vi "Register gRPC Messages.vi"(8 "error in (no error)":errorcluster, 11 "gRPC ID":T1) -> (0 "error out":errorcluster, 3 "gRPC ID Out":T1)   [LabVIEW 2025, in "xnet-grpc_client.lvlib"]
uses:
  xnet-grpc_client.lvlib
  <vilib>/gRPC/LabVIEW gRPC Library/Shared/grpcId.ctl
  <vilib>/gRPC/LabVIEW gRPC Library/Server API/typeDefs/Message Metadata.ctl
  <vilib>/gRPC/LabVIEW gRPC Library/Server API/typeDefs/Message Element Metadata.ctl
  <vilib>/gRPC/LabVIEW gRPC Library/Server API/typeDefs/Message Element Type.ctl
  <vilib>/gRPC/LabVIEW gRPC Library/Server API/typeDefs/Enum Metadata.ctl
  <vilib>/gRPC/LabVIEW gRPC Library/grpc-lvsupport-release.lvlib
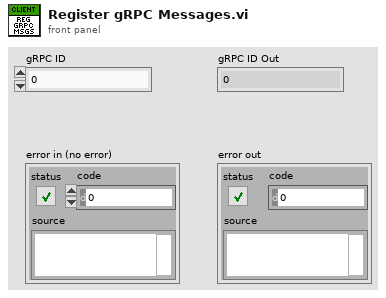
[diagram p1: front panel]
types:
  T1 = typedef "grpc-lvsupport-release.lvlib/grpcId.ctl" = u64
  T2 = typedef "grpc-lvsupport-release.lvlib/Enum Metadata.ctl" = cluster{"Version":i32, "Name":string, "Type Url":string, "Enum Values":string, "Allow Alias":bool}
  T3 = typedef "grpc-lvsupport-release.lvlib/Message Metadata.ctl" = cluster{"Version":i32, "Name":string, "Type Url":string, "Elements":T4[], "Has Oneof":bool}
  T4 = typedef "grpc-lvsupport-release.lvlib/Message Element Metadata.ctl" = cluster{"Field Name":string, "Embedded Message Name":string, "Protobuf Index":i32, "MessageElementType":T5, "Repeated":bool, "Is in Oneof":bool, "Oneof Container Name":string}
  T5 = typedef "grpc-lvsupport-release.lvlib/Message Element Type.ctl" = enum32{"Int32Value", "FloatValue", "DoubleValue", "BoolValue", "StringValue", "MessageValue", "Int64Value", "UInt32Value", "UInt64Value", "EnumValue", "Bytes", "Fixed64", "Fixed32", "SFixed64", "SFixed32", "SInt64", "SInt32"}
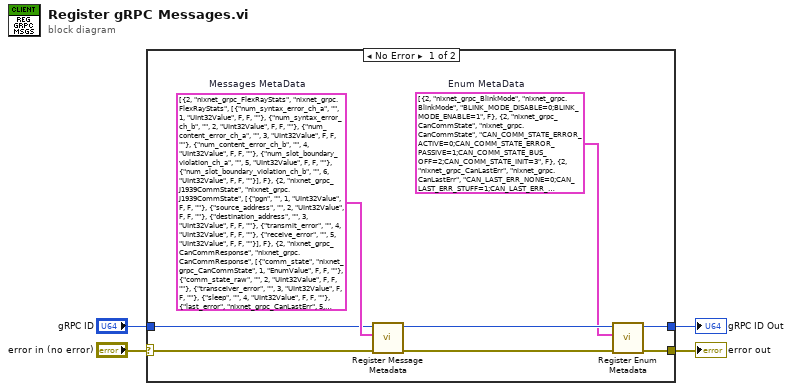
[diagram p0: block diagram]
diagram:
  n1 = case shown="No Error" "error in (no error)" {
    selector: "error in (no error)" -> [w10 w13]
    tunnel: [w9 w12] -> w1
    tunnel: [w6 w13] -> w4
    tunnel: "gRPC ID" -> [w9 w12]
    frame No Error {
      w5 = T2[] [{"Version"=2, "Name"="nixnet_grpc_BlinkMode", "Type Url"="nixnet_grpc.BlinkMode", "Enum Values"="BLINK_MODE_DISABLE=0;BLINK_MODE_ENABLE=1", "Allow Alias"=FALSE}, {"Version"=2, "Name"="nixnet_grpc_CanCommState", "Type Url"="nixnet_grpc.CanCommState", "Enum Values"="CAN_COMM_STATE_ERROR_ACTIVE=0;CAN_COMM_STATE_ERROR_PASSIVE=1;CAN_COMM_STATE_BUS_OFF=2;CAN_COMM_STATE_INIT=3", "Allow Alias"=FALSE}, {"Version"=2, "Name"="nixnet_grpc_CanLastErr", "Type Url"="nixnet_grpc.CanLastErr", "Enum Values"="CAN_LAST_ERR_NONE=0;CAN_LAST_ERR_STUFF=1;CAN_LAST_ERR_FORM=2;CAN_LAST_ERR_ACK=3;CAN_LAST_ERR_BIT_1=4;CAN_LAST_ERR_BIT_0=5;CAN_LAST_ERR_CRC=6", "Allow Alias"=FALSE}, {"Version"=2, "Name"="nixnet_grpc_CopyMode", "Type Url"="nixnet_grpc.CopyMode", "Enum Values"="COPY_MODE_DB_MERGE_COPY_USE_SOURCE=0;COPY_MODE_DB_MERGE_COPY_USE_TARGET=1;COPY_MODE_DB_MERGE_MERGE_USE_SOURCE=2;COPY_MODE_DB_MERGE_MERGE_USE_TARGET=3", "Allow Alias"=FALSE}, {"Version"=2, "Name"="nixnet_grpc_CreateSessionMode", "Type Url"="nixnet_grpc.CreateSessionMode", "Enum Values"="CREATE_SESSION_MODE_SIGNAL_IN_SINGLE_POINT=0;CREATE_SESSION_MODE_SIGNAL_IN_WAVEFORM=1;CREATE_SESSION_MODE_SIGNAL_IN_XY=2;CREATE_SESSION_MODE_SIGNAL_OUT_SINGLE_POINT=3;CREATE_SESSION_MODE_SIGNAL_OUT_WAVEFORM=4;CREATE_SESSION_MODE_SIGNAL_OUT_XY=5;CREATE_SESSION_MODE_FRAME_IN_STREAM=6;CREATE_SESSION_MODE_FRAME_IN_QUEUED=7;CREATE_SESSION_MODE_FRAME_IN_SINGLE_POINT=8;CREATE_SESSION_MODE_FRAME_OUT_STREAM=9;CREATE_SESSION_MODE_FRAME_OUT_QUEUED=10;CREATE_SESSION_MODE_FRAME_OUT_SINGLE_POINT=11;CREATE_SESSION_MODE_SIGNAL_CONVERSION_SINGLE_POINT=12", "Allow Alias"=FALSE}, {"Version"=2, "Name"="nixnet_grpc_DBProperty", "Type Url"="nixnet_grpc.DBProperty", "Enum Values"="DB_PROPERTY_UNSPECIFIED=0;DB_PROPERTY_DATABASE_CLST_REFS=100663298;DB_PROPERTY_DATABASE_NAME=50331649;DB_PROPERTY_DATABASE_SHOW_INVALID_FROM_OPEN=33554435;DB_PROPERTY_CLST_BAUD_RATE_64=151060481;DB_PROPERTY_CLST_APPLICATION_PROTOCOL=65651;DB_PROPERTY_CLST_BAUD_RATE=65537;DB_PROPERTY_CLST_CAN_FD_BAUD_RATE_64=151060497;DB_PROPERTY_CLST_CAN_FD_BAUD_RATE=65553;DB_PROPERTY_CLST_CAN_FD_ISO_MODE=65652;DB_PROPERTY_CLST_CAN_IO_MODE=65552;DB_PROPERTY_CLST_COMMENT=50397192;DB_PROPERTY_CLST_CONFIG_STATUS=65545;DB_PROPERTY_CLST_DATABASE_REF=83951618;DB_PROPERTY_CLST_ECU_REFS=100728835;DB_PROPERTY_CLST_FLEX_RAY_ACT_PT_OFF=65568;DB_PROPERTY_CLST_FLEX_RAY_ALW_PASS_ACT=65650;DB_PROPERTY_CLST_FLEX_RAY_CAS_RX_L_MAX=65569;DB_PROPERTY_CLST_FLEX_RAY_CHANNELS=65570;DB_PROPERTY_CLST_FLEX_RAY_CLST_DRIFT_DMP=65571;DB_PROPERTY_CLST_FLEX_RAY_COLD_ST_ATS=65572;DB_PROPERTY_CLST_FLEX_RAY_CYCLE=65573;DB_PROPERTY_CLST_FLEX_RAY_DYN_SEG_START=65574;DB_PROPERTY_CLST_FLEX_RAY_DYN_SLOT_IDL_PH=65575;DB_PROPERTY_CLST_FLEX_RAY_LATEST_GUAR_DYN=65579;DB_PROPERTY_CLST_FLEX_RAY_LATEST_USABLE_DYN=65578;DB_PROPERTY_CLST_FLEX_RAY_LIS_NOISE=65576;DB_PROPERTY_CLST_FLEX_RAY_MACRO_PER_CYCLE=65577;DB_PROPERTY_CLST_FLEX_RAY_MACROTICK=16842800;DB_PROPERTY_CLST_FLEX_RAY_MAX_WO_CLK_COR_FAT=65585;DB_PROPERTY_CLST_FLEX_RAY_MAX_WO_CLK_COR_PAS=65586;DB_PROPERTY_CLST_FLEX_RAY_MINISLOT=65588;DB_PROPERTY_CLST_FLEX_RAY_MINISLOT_ACT_PT=65587;DB_PROPERTY_CLST_FLEX_RAY_NIT=65590;DB_PROPERTY_CLST_FLEX_RAY_NIT_START=65591;DB_PROPERTY_CLST_FLEX_RAY_NM_VEC_LEN=65589;DB_PROPERTY_CLST_FLEX_RAY_NUM_MINISLT=65592;DB_PROPERTY_CLST_FLEX_RAY_NUM_STAT_SLT=65593;DB_PROPERTY_CLST_FLEX_RAY_OFF_COR_ST=65600;DB_PROPERTY_CLST_FLEX_RAY_PAYLD_LEN_DYN_MAX=65601;DB_PROPERTY_CLST_FLEX_RAY_PAYLD_LEN_MAX=65602;DB_PROPERTY_CLST_FLEX_RAY_PAYLD_LEN_ST=65603;DB_PROPERTY_CLST_FLEX_RAY_STAT_SLOT=65605;DB_PROPERTY_CLST_FLEX_RAY_SYM_WIN=65606;DB_PROPERTY_CLST_FLEX_RAY_SYM_WIN_START=65607;DB_PROPERTY_CLST_FLEX_RAY_SYNC_NODE_MAX=65608;DB_PROPERTY_CLST_FLEX_RAY_TSS_TX=65609;DB_PROPERTY_CLST_FLEX_RAY_USE_WAKEUP=33620053;DB_PROPERTY_CLST_FLEX_RAY_WAKE_SYM_RX_IDL=65616;DB_PROPERTY_CLST_FLEX_RAY_WAKE_SYM_RX_LOW=65617;DB_PROPERTY_CLST_FLEX_RAY_WAKE_SYM_RX_WIN=65618;DB_PROPERTY_CLST_FLEX_RAY_WAKE_SYM_TX_IDL=65619;DB_PROPERTY_CLST_FLEX_RAY_WAKE_SYM_TX_LOW=65620;DB_PROPERTY_CLST_FRM_REFS=100728836;DB_PROPERTY_CLST_LIN_SCHEDULES=100728944;DB_PROPERTY_CLST_LIN_TICK=16842865;DB_PROPERTY_CLST_NAME=50397189;DB_PROPERTY_CLST_PDU_REFS=100728840;DB_PROPERTY_CLST_PD_US_REQD=33619978;DB_PROPERTY_CLST_PROTOCOL=65542;DB_PROPERTY_CLST_SIG_REFS=100728839;DB_PROPERTY_FRM_APPLICATION_PROTOCOL=131172;DB_PROPERTY_FRM_CAN_EXT_ID=33685520;DB_PROPERTY_FRM_CAN_IO_MODE=131174;DB_PROPERTY_FRM_CAN_TIMING_TYPE=131089;DB_PROPERTY_FRM_CAN_TX_TIME=16908306;DB_PROPERTY_FRM_CLUSTER_REF=84017153;DB_PROPERTY_FRM_COMMENT=50462722;DB_PROPERTY_FRM_CONFIG_STATUS=131081;DB_PROPERTY_FRM_DEFAULT_PAYLOAD=167903237;DB_PROPERTY_FRM_FLEX_RAY_BASE_CYCLE=131104;DB_PROPERTY_FRM_FLEX_RAY_CH_ASSIGN=131105;DB_PROPERTY_FRM_FLEX_RAY_CYCLE_REP=131106;DB_PROPERTY_FRM_FLEX_RAY_IN_CYC_REP_CH_ASSIGNS=134348850;DB_PROPERTY_FRM_FLEX_RAY_IN_CYC_REP_ENABLED=33685552;DB_PROPERTY_FRM_FLEX_RAY_IN_CYC_REP_IDS=134348849;DB_PROPERTY_FRM_FLEX_RAY_PREAMBLE=33685539;DB_PROPERTY_FRM_FLEX_RAY_STARTUP=33685540;DB_PROPERTY_FRM_FLEX_RAY_SYNC=33685541;DB_PROPERTY_FRM_FLEX_RAY_TIMING_TYPE=131110;DB_PROPERTY_FRM_ID=131075;DB_PROPERTY_FRM_LIN_CHECKSUM=131152;DB_PROPERTY_FRM_MUX_DATA_MUX_SIG_REF=84017217;DB_PROPERTY_FRM_MUX_IS_MUXED=33685568;DB_PROPERTY_FRM_MUX_STATIC_SIG_REFS=100794434;DB_PROPERTY_FRM_MUX_SUBFRAME_REFS=100794435;DB_PROPERTY_FRM_NAME=50462724;DB_PROPERTY_FRM_PDU_START_BITS=134348897;DB_PROPERTY_FRM_PDU_UPDATE_BITS=134348899;DB_PROPERTY_FRM_PDU_REFS=100794464;DB_PROPERTY_FRM_PAYLOAD_LEN=131079;DB_PROPERTY_FRM_SIG_REFS=100794376;DB_PROPERTY_FRM_VARIABLE_PAYLOAD=33685605;DB_PROPERTY_SIG_BYTE_ORDR=196609;DB_PROPERTY_SIG_COMMENT=50528258;DB_PROPERTY_SIG_CONFIG_STATUS=196617;DB_PROPERTY_SIG_DATA_TYPE=196611;DB_PROPERTY_SIG_DEFAULT=16973828;DB_PROPERTY_SIG_FRAME_REF=84082693;DB_PROPERTY_SIG_MAX=16973830;DB_PROPERTY_SIG_MIN=16973831;DB_PROPERTY_SIG_MUX_IS_DATA_MUX=33751088;DB_PROPERTY_SIG_MUX_IS_DYNAMIC=33751089;DB_PROPERTY_SIG_MUX_VALUE=196658;DB_PROPERTY_SIG_MUX_SUBFRM_REF=84082739;DB_PROPERTY_SIG_NAME=50528264;DB_PROPERTY_SIG_NAME_UNIQUE_TO_CLUSTER=50528272;DB_PROPERTY_SIG_NUM_BITS=196626;DB_PROPERTY_SIG_PDU_REF=84082705;DB_PROPERTY_SIG_SCALE_FAC=16973843;DB_PROPERTY_SIG_SCALE_OFF=16973844;DB_PROPERTY_SIG_START_BIT=196629;DB_PROPERTY_SIG_UNIT=50528278;DB_PROPERTY_SUBFRM_CONFIG_STATUS=262153;DB_PROPERTY_SUBFRM_DYN_SIG_REFS=100925441;DB_PROPERTY_SUBFRM_FRM_REF=84148226;DB_PROPERTY_SUBFRM_MUX_VALUE=262147;DB_PROPERTY_SUBFRM_NAME=50593796;DB_PROPERTY_SUBFRM_NAME_UNIQUE_TO_CLUSTER=50593799;DB_PROPERTY_SUBFRM_PDU_REF=84148229;DB_PROPERTY_ECU_CLST_REF=84213761;DB_PROPERTY_ECU_COMMENT=50659333;DB_PROPERTY_ECU_CONFIG_STATUS=327689;DB_PROPERTY_ECU_FLEX_RAY_IS_COLDSTART=33882128;DB_PROPERTY_ECU_FLEX_RAY_CONNECTED_CHS=327700;DB_PROPERTY_ECU_FLEX_RAY_STARTUP_FRAME_REF=84213777;DB_PROPERTY_ECU_FLEX_RAY_WAKEUP_CHS=327699;DB_PROPERTY_ECU_FLEX_RAY_WAKEUP_PTRN=327698;DB_PROPERTY_ECU_RX_FRM_REFS=100990979;DB_PROPERTY_ECU_TX_FRM_REFS=100990980;DB_PROPERTY_ECU_LIN_CONFIG_NAD=327715;DB_PROPERTY_ECU_LIN_FUNCTION_ID=327717;DB_PROPERTY_ECU_LIN_INITIAL_NAD=327714;DB_PROPERTY_ECU_LIN_MASTER=33882144;DB_PROPERTY_ECU_LINP2MIN=17104934;DB_PROPERTY_ECU_LIN_PROTOCOL_VER=327713;DB_PROPERTY_ECU_LINS_TMIN=17104935;DB_PROPERTY_ECU_LIN_SUPPLIER_ID=327716;DB_PROPERTY_ECU_NAME=50659330;DB_PROPERTY_ECU_J1939_NODE_NAME=151322665;DB_PROPERTY_ECU_J1939_PREFERRED_ADDRESS=327720;DB_PROPERTY_LIN_SCHED_CLST_REF=84279301;DB_PROPERTY_LIN_SCHED_COMMENT=50724870;DB_PROPERTY_LIN_SCHED_CONFIG_STATUS=393223;DB_PROPERTY_LIN_SCHED_ENTRIES=101056513;DB_PROPERTY_LIN_SCHED_NAME=50724866;DB_PROPERTY_LIN_SCHED_PRIORITY=393219;DB_PROPERTY_LIN_SCHED_RUN_MODE=393220;DB_PROPERTY_LIN_SCHED_ENTRY_COLLISION_RES_SCHED=84344833;DB_PROPERTY_LIN_SCHED_ENTRY_DELAY=17235970;DB_PROPERTY_LIN_SCHED_ENTRY_EVENT_ID=458755;DB_PROPERTY_LIN_SCHED_ENTRY_FRAMES=101122052;DB_PROPERTY_LIN_SCHED_ENTRY_NAME=50790406;DB_PROPERTY_LIN_SCHED_ENTRY_NAME_UNIQUE_TO_CLUSTER=50790408;DB_PROPERTY_LIN_SCHED_ENTRY_NC_FF_DATA_BYTES=168230921;DB_PROPERTY_LIN_SCHED_ENTRY_SCHED=84344839;DB_PROPERTY_LIN_SCHED_ENTRY_TYPE=458757;DB_PROPERTY_PDU_CLUSTER_REF=84410372;DB_PROPERTY_PDU_COMMENT=50855938;DB_PROPERTY_PDU_CONFIG_STATUS=524295;DB_PROPERTY_PDU_DEFAULT_PAYLOAD=168296453;DB_PROPERTY_PDU_FRM_REFS=101187590;DB_PROPERTY_PDU_MUX_DATA_MUX_SIG_REF=84410377;DB_PROPERTY_PDU_MUX_IS_MUXED=34078728;DB_PROPERTY_PDU_MUX_STATIC_SIG_REFS=101187594;DB_PROPERTY_PDU_MUX_SUBFRAME_REFS=101187595;DB_PROPERTY_PDU_NAME=50855937;DB_PROPERTY_PDU_PAYLOAD_LEN=524291;DB_PROPERTY_PDU_SIG_REFS=101187589", "Allow Alias"=FALSE}, {"Version"=2, "Name"="nixnet_grpc_DBPropertyValue", "Type Url"="nixnet_grpc.DBPropertyValue", "Enum Values"="DB_PROPERTY_VALUE_UNSPECIFIED=0;DB_PROPERTY_VALUE_CAN_IO_MODE_CAN=1;DB_PROPERTY_VALUE_CAN_IO_MODE_CAN_FD=2;DB_PROPERTY_VALUE_CAN_IO_MODE_CAN_FD_BRS=3;DB_PROPERTY_VALUE_PROTOCOL_UNKNOWN=4;DB_PROPERTY_VALUE_PROTOCOL_CAN=5;DB_PROPERTY_VALUE_PROTOCOL_FLEX_RAY=6;DB_PROPERTY_VALUE_PROTOCOL_LIN=7;DB_PROPERTY_VALUE_PROTOCOL_ETHERNET=8;DB_PROPERTY_VALUE_APP_PROTOCOL_NONE=9;DB_PROPERTY_VALUE_APP_PROTOCOL_J1939=10;DB_PROPERTY_VALUE_FRM_FLEX_RAY_CH_ASSIGN_A=11;DB_PROPERTY_VALUE_FRM_FLEX_RAY_CH_ASSIGN_B=12;DB_PROPERTY_VALUE_FRM_FLEX_RAY_CH_ASSIGN_A_AND_B=13;DB_PROPERTY_VALUE_FRM_FLEX_RAY_CH_ASSIGN_NONE=14;DB_PROPERTY_VALUE_CLST_FLEX_RAY_SAMP_CLK_PER_P0125US=15;DB_PROPERTY_VALUE_CLST_FLEX_RAY_SAMP_CLK_PER_P025US=16;DB_PROPERTY_VALUE_CLST_FLEX_RAY_SAMP_CLK_PER_P05US=17;DB_PROPERTY_VALUE_SIG_BYTE_ORDR_LITTLE_ENDIAN=18;DB_PROPERTY_VALUE_SIG_BYTE_ORDR_BIG_ENDIAN=19;DB_PROPERTY_VALUE_SIG_DATA_TYPE_SIGNED=20;DB_PROPERTY_VALUE_SIG_DATA_TYPE_UNSIGNED=21;DB_PROPERTY_VALUE_SIG_DATA_TYPE_IEEE_FLOAT=22;DB_PROPERTY_VALUE_SIG_DATA_TYPE_BYTE_ARRAY=23;DB_PROPERTY_VALUE_LIN_PROTOCOL_VER_1_2=24;DB_PROPERTY_VALUE_LIN_PROTOCOL_VER_1_3=25;DB_PROPERTY_VALUE_LIN_PROTOCOL_VER_2_0=26;DB_PROPERTY_VALUE_LIN_PROTOCOL_VER_2_1=27;DB_PROPERTY_VALUE_LIN_PROTOCOL_VER_2_2=28;DB_PROPERTY_VALUE_LIN_SCHED_RUN_MODE_CONTINUOUS=29;DB_PROPERTY_VALUE_LIN_SCHED_RUN_MODE_ONCE=30;DB_PROPERTY_VALUE_LIN_SCHED_RUN_MODE_NULL=31;DB_PROPERTY_VALUE_LIN_SCHED_ENTRY_TYPE_UNCONDITIONAL=32;DB_PROPERTY_VALUE_LIN_SCHED_ENTRY_TYPE_SPORADIC=33;DB_PROPERTY_VALUE_LIN_SCHED_ENTRY_TYPE_EVENT_TRIGGERED=34;DB_PROPERTY_VALUE_LIN_SCHED_ENTRY_TYPE_NODE_CONFIG_SERVICE=35", "Allow Alias"=FALSE}, {"Version"=2, "Name"="nixnet_grpc_EnetFlags", "Type Url"="nixnet_grpc.EnetFlags", "Enum Values"="ENET_FLAGS_UNSPECIFIED=0;ENET_FLAGS_TRANSMIT=1;ENET_FLAGS_RECEIVE=2;ENET_FLAGS_NETWORK_SYNCED=3;ENET_FLAGS_ERROR=4", "Allow Alias"=FALSE}, {"Version"=2, "Name"="nixnet_grpc_EnetFrameType", "Type Url"="nixnet_grpc.EnetFrameType", "Enum Values"="ENET_FRAME_TYPE_DATA=0;ENET_FRAME_TYPE_DELAY=225;ENET_FRAME_TYPE_FUTURE_TIME_WAIT=226", "Allow Alias"=FALSE}, {"Version"=2, "Name"="nixnet_grpc_FlexRayPocState", "Type Url"="nixnet_grpc.FlexRayPocState", "Enum Values"="FLEX_RAY_POC_STATE_DEFAULT_CONFIG=0;FLEX_RAY_POC_STATE_READY=1;FLEX_RAY_POC_STATE_NORMAL_ACTIVE=2;FLEX_RAY_POC_STATE_NORMAL_PASSIVE=3;FLEX_RAY_POC_STATE_HALT=4;FLEX_RAY_POC_STATE_MONITOR=5;FLEX_RAY_POC_STATE_CONFIG=15", "Allow Alias"=FALSE}, {"Version"=2, "Name"="nixnet_grpc_FlexRaySymbol", "Type Url"="nixnet_grpc.FlexRaySymbol", "Enum Values"="FLEX_RAY_SYMBOL_MTS=0;FLEX_RAY_SYMBOL_WAKEUP=1", "Allow Alias"=FALSE}, {"Version"=2, "Name"="nixnet_grpc_FrameFlags", "Type Url"="nixnet_grpc.FrameFlags", "Enum Values"="FRAME_FLAGS_UNSPECIFIED=0;FRAME_FLAGS_FLEX_RAY_STARTUP=1;FRAME_FLAGS_FLEX_RAY_SYNC=2;FRAME_FLAGS_FLEX_RAY_PREAMBLE=4;FRAME_FLAGS_FLEX_RAY_CH_A=16;FRAME_FLAGS_FLEX_RAY_CH_B=32;FRAME_FLAGS_LIN_EVENT_SLOT=1;FRAME_FLAGS_TRANSMIT_ECHO=128", "Allow Alias"=TRUE}, {"Version"=2, "Name"="nixnet_grpc_FrameType", "Type Url"="nixnet_grpc.FrameType", "Enum Values"="FRAME_TYPE_CAN_DATA=0;FRAME_TYPE_CAN_REMOTE=1;FRAME_TYPE_CAN_BUS_ERROR=2;FRAME_TYPE_CAN20_DATA=8;FRAME_TYPE_CANFD_DATA=16;FRAME_TYPE_CANFDBRS_DATA=24;FRAME_TYPE_FLEX_RAY_DATA=32;FRAME_TYPE_FLEX_RAY_NULL=33;FRAME_TYPE_FLEX_RAY_SYMBOL=34;FRAME_TYPE_LIN_DATA=64;FRAME_TYPE_LIN_BUS_ERROR=65;FRAME_TYPE_LIN_NO_RESPONSE=66;FRAME_TYPE_J1939_DATA=192;FRAME_TYPE_SPECIAL_DELAY=224;FRAME_TYPE_SPECIAL_LOG_TRIGGER=225;FRAME_TYPE_SPECIAL_START_TRIGGER=226", "Allow Alias"=FALSE}, {"Version"=2, "Name"="nixnet_grpc_GetDBCAttributeMode", "Type Url"="nixnet_grpc.GetDBCAttributeMode", "Enum Values"="GET_DBC_ATTRIBUTE_MODE_ATTRIBUTE=0;GET_DBC_ATTRIBUTE_MODE_ENUMERATION_LIST=1;GET_DBC_ATTRIBUTE_MODE_ATTRIBUTE_LIST=2;GET_DBC_ATTRIBUTE_MODE_VALUE_TABLE_LIST=3", "Allow Alias"=FALSE}, {"Version"=2, "Name"="nixnet_grpc_LinCommState", "Type Url"="nixnet_grpc.LinCommState", "Enum Values"="LIN_COMM_STATE_IDLE=0;LIN_COMM_STATE_ACTIVE=1;LIN_COMM_STATE_INACTIVE=2", "Allow Alias"=FALSE}, {"Version"=2, "Name"="nixnet_grpc_LinDiagnosticSchedule", "Type Url"="nixnet_grpc.LinDiagnosticSchedule", "Enum Values"="LIN_DIAGNOSTIC_SCHEDULE_NULL=0;LIN_DIAGNOSTIC_SCHEDULE_MASTER_REQ=1;LIN_DIAGNOSTIC_SCHEDULE_SLAVE_RESP=2", "Allow Alias"=FALSE}, {"Version"=2, "Name"="nixnet_grpc_LinLastErrCode", "Type Url"="nixnet_grpc.LinLastErrCode", "Enum Values"="LIN_LAST_ERR_CODE_NONE=0;LIN_LAST_ERR_CODE_UNKNOWN_ID=1;LIN_LAST_ERR_CODE_FORM=2;LIN_LAST_ERR_CODE_FRAMING=3;LIN_LAST_ERR_CODE_READBACK=4;LIN_LAST_ERR_CODE_TIMEOUT=5;LIN_LAST_ERR_CODE_CRC=6", "Allow Alias"=FALSE}, {"Version"=2, "Name"="nixnet_grpc_Property", "Type Url"="nixnet_grpc.Property", "Enum Values"="PROPERTY_UNSPECIFIED=0;PROPERTY_SESSION_APPLICATION_PROTOCOL=1048721;PROPERTY_SESSION_AUTO_START=34603009;PROPERTY_SESSION_CLUSTER_NAME=51380234;PROPERTY_SESSION_DATABASE_NAME=51380226;PROPERTY_SESSION_ENET_FRAME_FILTER=51380468;PROPERTY_SESSION_ENET_LOG_ERROR=34603197;PROPERTY_SESSION_ENET_LOG_FILE=51380410;PROPERTY_SESSION_ENET_LOG_MODE=1048761;PROPERTY_SESSION_ENET_LOG_ENABLE_MULTIPLE_FILES=34603257;PROPERTY_SESSION_ENET_LOG_FILE_SIZE_THRESHOLD=152043770;PROPERTY_SESSION_ENET_LOG_OPERATION=1048763;PROPERTY_SESSION_ENET_NUM_FRAMES_RECEIVED=152043759;PROPERTY_SESSION_ENET_SOURCE_MAC_ADDRESS_AUTO=34603177;PROPERTY_SESSION_INTF_BAUD_RATE_64=152043542;PROPERTY_SESSION_INTF_ADJUST_LOCAL_TIME=152043691;PROPERTY_SESSION_INTF_BAUD_RATE=1048598;PROPERTY_SESSION_INTF_BUS_ERR_TO_IN_STRM=34603029;PROPERTY_SESSION_INTF_CAN_FD_BAUD_RATE_64=152043559;PROPERTY_SESSION_INTF_CAN_DISABLE_PROT_EXCEPTION_HANDLING=34603172;PROPERTY_SESSION_INTF_CAN_EDGE_FILTER=34603170;PROPERTY_SESSION_INTF_CAN_EXT_TCVR_CONFIG=1048611;PROPERTY_SESSION_INTF_CAN_FD_BAUD_RATE=1048615;PROPERTY_SESSION_INTF_CAN_FD_ISO_MODE=1048638;PROPERTY_SESSION_INTF_CAN_IO_MODE=1048614;PROPERTY_SESSION_INTF_CAN_LSTN_ONLY=34603042;PROPERTY_SESSION_INTF_CAN_PEND_TX_ORDER=1048608;PROPERTY_SESSION_INTF_CAN_SING_SHOT=34603044;PROPERTY_SESSION_INTF_CAN_TERM=1048613;PROPERTY_SESSION_INTF_CAN_TCVR_STATE=1048616;PROPERTY_SESSION_INTF_CAN_TCVR_TYPE=1048617;PROPERTY_SESSION_INTF_CAN_TX_IO_MODE=1048633;PROPERTY_SESSION_INTF_CAN_TRANSMIT_PAUSE=34603171;PROPERTY_SESSION_INTF_ECHO_TX=34603024;PROPERTY_SESSION_INTF_ENET_EPT_RECEIVE_FILTER=202375356;PROPERTY_SESSION_INTF_ENET_EPT_TRANSMIT_BANDWIDTH=152043711;PROPERTY_SESSION_INTF_ENET_IPV4_ADDRESS=51380459;PROPERTY_SESSION_INTF_ENET_JUMBO_FRAMES=1048819;PROPERTY_SESSION_INTF_ENET_LINK_SPEED=1048818;PROPERTY_SESSION_INTF_ENET_LINK_SPEED_CONFIGURED=1048817;PROPERTY_SESSION_INTF_ENET_MAC_ADDRESS=51380392;PROPERTY_SESSION_INTF_ENET_OS_NETWORK_ADAPTER_DESCRIPTION=51380461;PROPERTY_SESSION_INTF_ENET_OS_NETWORK_ADAPTER_NAME=51380460;PROPERTY_SESSION_INTF_ENET_OPERATIONAL_STATUS=1048746;PROPERTY_SESSION_INTF_ENET_OUT_STRM_TIMESCALE=1048823;PROPERTY_SESSION_INTF_ENET_PHY_POWER_MODE=1048825;PROPERTY_SESSION_INTF_ENET_PHY_STATE=1048743;PROPERTY_SESSION_INTF_ENET_PORT_MODE=1048742;PROPERTY_SESSION_INTF_ENET_SIGNAL_QUALITY=235929846;PROPERTY_SESSION_INTF_ENET_SLEEP_CAPABILITY=1048824;PROPERTY_SESSION_INTF_ENET_STATS_COUNTER_NAMES=68157612;PROPERTY_SESSION_INTF_ENET_STATS_COUNTER_VALUES=68157613;PROPERTY_SESSION_INTF_ENET_STATS_RX_BAD_FRAMES=152043702;PROPERTY_SESSION_INTF_ENET_STATS_RX_BYTES=152043694;PROPERTY_SESSION_INTF_ENET_STATS_RX_GOOD_FRAMES=152043695;PROPERTY_SESSION_INTF_ENET_STATS_TX_BYTES=152043703;PROPERTY_SESSION_INTF_ENET_STATS_TX_GOOD_FRAMES=152043704;PROPERTY_SESSION_INTF_ENET_STATS_PHY_COUNTER_NAMES=68157693;PROPERTY_SESSION_INTF_ENET_STATS_PHY_COUNTER_VALUES=68157694;PROPERTY_SESSION_INTF_ENET_STATS_PHY_LOW_POWER_SLEEP=152043777;PROPERTY_SESSION_INTF_ENET_STATS_PHY_SLEEP_FAILURE=152043779;PROPERTY_SESSION_INTF_ENET_STATS_PHY_WAKEUP_FAILURE=152043778;PROPERTY_SESSION_INTF_ENET_STATS_PHY_WAKEUP_PULSE=152043775;PROPERTY_SESSION_INTF_ENET_STATS_PHY_WAKEUP_REQUEST=152043776;PROPERTY_SESSION_INTF_ENET_TIME_ADJUST_NETWORK_TIME=152043729;PROPERTY_SESSION_INTF_ENET_TIME_BMCA_ENABLED=34603202;PROPERTY_SESSION_INTF_ENET_TIME_CLK_ACCURACY=1048774;PROPERTY_SESSION_INTF_ENET_TIME_CLK_CLASS=1048773;PROPERTY_SESSION_INTF_ENET_TIME_CLK_ID=51380420;PROPERTY_SESSION_INTF_ENET_TIME_CLK_OFFSET_VAR=1048775;PROPERTY_SESSION_INTF_ENET_TIME_GM_CLK_ACCURACY=1048781;PROPERTY_SESSION_INTF_ENET_TIME_GM_CLK_CLASS=1048780;PROPERTY_SESSION_INTF_ENET_TIME_GM_CLK_ID=51380427;PROPERTY_SESSION_INTF_ENET_TIME_GM_CLK_OFFSET_VAR=1048782;PROPERTY_SESSION_INTF_ENET_TIME_GM_PRIORITY_1=1048783;PROPERTY_SESSION_INTF_ENET_TIME_GM_PRIORITY_2=1048784;PROPERTY_SESSION_INTF_ENET_TIME_OFFSET_FROM_MASTER=152043715;PROPERTY_SESSION_INTF_ENET_TIME_PORT_AS_CAPABLE=34603233;PROPERTY_SESSION_INTF_ENET_TIME_PORT_ANNOUNCE_RECEIPT_TIMEOUT=1048800;PROPERTY_SESSION_INTF_ENET_TIME_PORT_ANNOUNCE_TRANSMIT_ENABLED=34603231;PROPERTY_SESSION_INTF_ENET_TIME_PORT_LOG_ANNOUNCE_INTERVAL=1048798;PROPERTY_SESSION_INTF_ENET_TIME_PORT_LOG_ANNOUNCE_INTERVAL_CONFIGURED=1048797;PROPERTY_SESSION_INTF_ENET_TIME_PORT_LOG_PDELAY_INTERVAL=1048793;PROPERTY_SESSION_INTF_ENET_TIME_PORT_LOG_PDELAY_INTERVAL_CONFIGURED=1048792;PROPERTY_SESSION_INTF_ENET_TIME_PORT_LOG_SYNC_INTERVAL=1048795;PROPERTY_SESSION_INTF_ENET_TIME_PORT_LOG_SYNC_INTERVAL_CONFIGURED=1048794;PROPERTY_SESSION_INTF_ENET_TIME_PORT_PDELAY_ENABLED=34603223;PROPERTY_SESSION_INTF_ENET_TIME_PORT_STATE=1048787;PROPERTY_SESSION_INTF_ENET_TIME_PORT_STATE_CONFIGURED=1048786;PROPERTY_SESSION_INTF_ENET_TIME_PORT_PROP_DELAY=17826004;PROPERTY_SESSION_INTF_ENET_TIME_PORT_PROP_DELAY_CONFIGURED=17826005;PROPERTY_SESSION_INTF_ENET_TIME_PORT_PROP_DELAY_THRESHOLD=17826006;PROPERTY_SESSION_INTF_ENET_TIME_PORT_STATS_COUNTER_NAMES=68157667;PROPERTY_SESSION_INTF_ENET_TIME_PORT_STATS_COUNTER_VALUES=68157668;PROPERTY_SESSION_INTF_ENET_TIME_PORT_STATS_RX_ANNOUNCE=152043750;PROPERTY_SESSION_INTF_ENET_TIME_PORT_STATS_RX_PDELAY_REQUEST=152043751;PROPERTY_SESSION_INTF_ENET_TIME_PORT_STATS_RX_SYNC=152043749;PROPERTY_SESSION_INTF_ENET_TIME_PORT_STATS_TX_ANNOUNCE=152043753;PROPERTY_SESSION_INTF_ENET_TIME_PORT_STATS_TX_PDELAY_REQUEST=152043754;PROPERTY_SESSION_INTF_ENET_TIME_PORT_STATS_TX_SYNC=152043752;PROPERTY_SESSION_INTF_ENET_TIME_PORT_SYNC_RECEIPT_TIMEOUT=1048796;PROPERTY_SESSION_INTF_ENET_TIME_PORT_SYNC_STATUS=1048816;PROPERTY_SESSION_INTF_ENET_TIME_PORT_SYNCED=34603234;PROPERTY_SESSION_INTF_ENET_TIME_PRIORITY_1=1048776;PROPERTY_SESSION_INTF_ENET_TIME_PRIORITY_2=1048777;PROPERTY_SESSION_INTF_ENET_TIME_PROTOCOL=1048768;PROPERTY_SESSION_INTF_ENET_TIME_PROTOCOL_ENABLED=34603201;PROPERTY_SESSION_INTF_ENET_TIME_STEPS_TO_GM=1048778;PROPERTY_SESSION_INTF_ENET_TRIGGER_PPS_SYNCED=34603268;PROPERTY_SESSION_INTF_FLEX_RAY_ACC_START_RNG=1048624;PROPERTY_SESSION_INTF_FLEX_RAY_ALW_HLT_CLK=34603057;PROPERTY_SESSION_INTF_FLEX_RAY_ALW_PASS_ACT=1048626;PROPERTY_SESSION_INTF_FLEX_RAY_AUTO_ASLP_WHN_STP=34603066;PROPERTY_SESSION_INTF_FLEX_RAY_CLST_DRIFT_DMP=1048627;PROPERTY_SESSION_INTF_FLEX_RAY_COLDSTART=34603060;PROPERTY_SESSION_INTF_FLEX_RAY_CONNECTED_CHS=1048636;PROPERTY_SESSION_INTF_FLEX_RAY_DEC_CORR=1048629;PROPERTY_SESSION_INTF_FLEX_RAY_DELAY_COMP_A=1048630;PROPERTY_SESSION_INTF_FLEX_RAY_DELAY_COMP_B=1048631;PROPERTY_SESSION_INTF_FLEX_RAY_KEY_SLOT_ID=1048632;PROPERTY_SESSION_INTF_FLEX_RAY_LATEST_TX=1048641;PROPERTY_SESSION_INTF_FLEX_RAY_LIST_TIMO=1048642;PROPERTY_SESSION_INTF_FLEX_RAY_MAC_INIT_OFF_A=1048643;PROPERTY_SESSION_INTF_FLEX_RAY_MAC_INIT_OFF_B=1048644;PROPERTY_SESSION_INTF_FLEX_RAY_MAX_DRIFT=1048647;PROPERTY_SESSION_INTF_FLEX_RAY_MIC_INIT_OFF_A=1048645;PROPERTY_SESSION_INTF_FLEX_RAY_MIC_INIT_OFF_B=1048646;PROPERTY_SESSION_INTF_FLEX_RAY_MICROTICK=1048648;PROPERTY_SESSION_INTF_FLEX_RAY_NULL_TO_IN_STRM=34603081;PROPERTY_SESSION_INTF_FLEX_RAY_OFF_CORR=1048664;PROPERTY_SESSION_INTF_FLEX_RAY_OFF_CORR_OUT=1048656;PROPERTY_SESSION_INTF_FLEX_RAY_RATE_CORR=1048665;PROPERTY_SESSION_INTF_FLEX_RAY_RATE_CORR_OUT=1048658;PROPERTY_SESSION_INTF_FLEX_RAY_SAMP_PER_MICRO=1048659;PROPERTY_SESSION_INTF_FLEX_RAY_SING_SLOT_EN=34603092;PROPERTY_SESSION_INTF_FLEX_RAY_SLEEP=1048635;PROPERTY_SESSION_INTF_FLEX_RAY_STATISTICS_EN=34603098;PROPERTY_SESSION_INTF_FLEX_RAY_SYM_TO_IN_STRM=34603069;PROPERTY_SESSION_INTF_FLEX_RAY_SYNC_STATUS=1048671;PROPERTY_SESSION_INTF_FLEX_RAY_SYNC_CH_A_EVEN=135266395;PROPERTY_SESSION_INTF_FLEX_RAY_SYNC_CH_A_ODD=135266396;PROPERTY_SESSION_INTF_FLEX_RAY_SYNC_CH_B_EVEN=135266397;PROPERTY_SESSION_INTF_FLEX_RAY_SYNC_CH_B_ODD=135266398;PROPERTY_SESSION_INTF_FLEX_RAY_TERM=1048663;PROPERTY_SESSION_INTF_FLEX_RAY_WAKEUP_CH=1048661;PROPERTY_SESSION_INTF_FLEX_RAY_WAKEUP_PTRN=1048662;PROPERTY_SESSION_INTF_NAME=51380243;PROPERTY_SESSION_INTF_LIN_BREAK_DELIMITER_LENGTH=1048821;PROPERTY_SESSION_INTF_LIN_BREAK_LENGTH=1048688;PROPERTY_SESSION_INTF_LIN_CHECKSUM_TO_IN_STRM=34603137;PROPERTY_SESSION_INTF_LIN_DIAG_P2_MIN=17825911;PROPERTY_SESSION_INTF_LIN_DIAG_ST_MIN=17825910;PROPERTY_SESSION_INTF_LIN_MASTER=34603122;PROPERTY_SESSION_INTF_LIN_NO_RESPONSE_TO_IN_STRM=34603136;PROPERTY_SESSION_INTF_LINO_STR_SLV_RSP_LST_BY_NAD=135266425;PROPERTY_SESSION_INTF_LIN_SCHED_NAMES=68157557;PROPERTY_SESSION_INTF_LIN_SLEEP=1048691;PROPERTY_SESSION_INTF_LIN_ALW_START_WO_BUS_PWR=34603128;PROPERTY_SESSION_INTF_LIN_TERM=1048692;PROPERTY_SESSION_INTF_OUT_STRM_LIST=101711889;PROPERTY_SESSION_INTF_OUT_STRM_LIST_BY_ID=135266337;PROPERTY_SESSION_INTF_OUT_STRM_TIMNG=1048594;PROPERTY_SESSION_INTF_SRC_TERM_START_TRIGGER=51380368;PROPERTY_SESSION_INTF_START_TRIG_TO_IN_STRM=34603028;PROPERTY_SESSION_LIST=68157443;PROPERTY_SESSION_MODE=1048580;PROPERTY_SESSION_NUM_IN_LIST=1048581;PROPERTY_SESSION_NUM_FRAMES=1048589;PROPERTY_SESSION_NUM_PEND=1048582;PROPERTY_SESSION_NUM_UNUSED=1048587;PROPERTY_SESSION_PAYLD_LEN_MAX=1048585;PROPERTY_SESSION_PROTOCOL=1048584;PROPERTY_SESSION_QUEUE_SIZE=1048588;PROPERTY_SESSION_RESAMP_RATE=17825799;PROPERTY_SESSION_J1939_ECU=84934803;PROPERTY_SESSION_J1939_ECU_BUSY=34603169;PROPERTY_SESSION_J1939_FILL_BYTE=1048735;PROPERTY_SESSION_J1939_INCLUDE_DEST_ADDR_IN_PGN=34603173;PROPERTY_SESSION_J1939_MAX_REPEAT_CTS=1048734;PROPERTY_SESSION_J1939_ADDRESS=1048722;PROPERTY_SESSION_J1939_NAME=152043668;PROPERTY_SESSION_J1939_NUM_PACKETS_RECV=1048732;PROPERTY_SESSION_J1939_NUM_PACKETS_RESP=1048733;PROPERTY_SESSION_J1939_HOLD_TIME_TH=17825947;PROPERTY_SESSION_J1939_RESPONSE_TIME_TR_GD=17825946;PROPERTY_SESSION_J1939_RESPONSE_TIME_TR_SD=17825945;PROPERTY_SESSION_J1939_TIMEOUT_T1=17825941;PROPERTY_SESSION_J1939_TIMEOUT_T2=17825942;PROPERTY_SESSION_J1939_TIMEOUT_T3=17825943;PROPERTY_SESSION_J1939_TIMEOUT_T4=17825944;PROPERTY_SESSION_J1939_WRITE_QUEUE_SIZE=1048736;PROPERTY_SYS_CDAQ_PKT_TIME=17891340;PROPERTY_SYS_DEV_REFS=101777410;PROPERTY_SYS_INTF_REFS=101777411;PROPERTY_SYS_INTF_REFS_ALL=101777421;PROPERTY_SYS_INTF_REFS_CAN=101777412;PROPERTY_SYS_INTF_REFS_ETHERNET=101777409;PROPERTY_SYS_INTF_REFS_FLEX_RAY=101777413;PROPERTY_SYS_INTF_REFS_LIN=101777415;PROPERTY_SYS_VER_BUILD=1114118;PROPERTY_SYS_VER_MAJOR=1114120;PROPERTY_SYS_VER_MINOR=1114121;PROPERTY_SYS_VER_PHASE=1114122;PROPERTY_SYS_VER_UPDATE=1114123;PROPERTY_DEV_FORM_FAC=1179649;PROPERTY_DEV_INTF_REFS=101842946;PROPERTY_DEV_INTF_REFS_ALL=101842952;PROPERTY_DEV_NUM_PORTS=1179652;PROPERTY_DEV_NUM_PORTS_ALL=1179655;PROPERTY_DEV_NAME=51511299;PROPERTY_DEV_PRODUCT_NUM=1179656;PROPERTY_DEV_SER_NUM=1179653;PROPERTY_DEV_SLOT_NUM=1179654;PROPERTY_INTF_CAN_TERM_CAP=1245192;PROPERTY_INTF_CAN_TCVR_CAP=1245191;PROPERTY_INTF_DEV_REF=85131265;PROPERTY_INTF_DONGLE_COMPATIBLE_FIRMWARE_VERSION=1245199;PROPERTY_INTF_DONGLE_COMPATIBLE_REVISION=1245198;PROPERTY_INTF_DONGLE_FIRMWARE_VERSION=1245197;PROPERTY_INTF_DONGLE_ID=1245194;PROPERTY_INTF_DONGLE_REVISION=1245196;PROPERTY_INTF_DONGLE_STATE=1245193;PROPERTY_INTF_NAME=51576834;PROPERTY_INTF_NUM=1245187;PROPERTY_INTF_PORT_NUM=1245188;PROPERTY_INTF_PROTOCOL=1245189", "Allow Alias"=FALSE}, {"Version"=2, "Name"="nixnet_grpc_PropertyValue", "Type Url"="nixnet_grpc.PropertyValue", "Enum Values"="PROPERTY_VALUE_UNSPECIFIED=0;PROPERTY_VALUE_CAN_FD_MODE_ISO=1;PROPERTY_VALUE_CAN_FD_MODE_NON_ISO=2;PROPERTY_VALUE_CAN_FD_MODE_ISO_LEGACY=3;PROPERTY_VALUE_CAN_IO_MODE_CAN=4;PROPERTY_VALUE_CAN_IO_MODE_CAN_FD=5;PROPERTY_VALUE_CAN_IO_MODE_CAN_FD_BRS=6;PROPERTY_VALUE_EPT_RX_FILTER_USE_FLAGS_VID=7;PROPERTY_VALUE_EPT_RX_FILTER_USE_FLAGS_PRIORITY=8;PROPERTY_VALUE_EPT_RX_FILTER_USE_FLAGS_DESTINATION_MAC=9;PROPERTY_VALUE_PHASE_DEVELOPMENT=10;PROPERTY_VALUE_PHASE_ALPHA=11;PROPERTY_VALUE_PHASE_BETA=12;PROPERTY_VALUE_PHASE_RELEASE=13;PROPERTY_VALUE_DEV_FORM_PXI=14;PROPERTY_VALUE_DEV_FORM_PCI=15;PROPERTY_VALUE_DEV_FORM_C_SERIES=16;PROPERTY_VALUE_DEV_FORM_PXIE=17;PROPERTY_VALUE_DEV_FORM_USB=18;PROPERTY_VALUE_DEV_FORM_PCIE=19;PROPERTY_VALUE_CAN_TERM_CAP_NO=20;PROPERTY_VALUE_CAN_TERM_CAP_YES=21;PROPERTY_VALUE_CAN_TCVR_CAP_HS=22;PROPERTY_VALUE_CAN_TCVR_CAP_LS=23;PROPERTY_VALUE_CAN_TCVR_CAP_XS=24;PROPERTY_VALUE_CAN_TCVR_CAP_XS_HS_LS=25;PROPERTY_VALUE_CAN_TCVR_CAP_UNKNOWN=26;PROPERTY_VALUE_PROTOCOL_UNKNOWN=27;PROPERTY_VALUE_PROTOCOL_CAN=28;PROPERTY_VALUE_PROTOCOL_FLEX_RAY=29;PROPERTY_VALUE_PROTOCOL_LIN=30;PROPERTY_VALUE_PROTOCOL_ETHERNET=31;PROPERTY_VALUE_APP_PROTOCOL_NONE=32;PROPERTY_VALUE_APP_PROTOCOL_J1939=33;PROPERTY_VALUE_DONGLE_STATE_NO_DONGLE_NO_EXT_POWER=34;PROPERTY_VALUE_DONGLE_STATE_NO_DONGLE_EXT_POWER=35;PROPERTY_VALUE_DONGLE_STATE_DONGLE_NO_EXT_POWER=36;PROPERTY_VALUE_DONGLE_STATE_READY=37;PROPERTY_VALUE_DONGLE_STATE_BUSY=38;PROPERTY_VALUE_DONGLE_STATE_COMM_ERROR=39;PROPERTY_VALUE_DONGLE_STATE_OVER_CURRENT=40;PROPERTY_VALUE_DONGLE_ID_LS_CAN=41;PROPERTY_VALUE_DONGLE_ID_HS_CAN=42;PROPERTY_VALUE_DONGLE_ID_SW_CAN=43;PROPERTY_VALUE_DONGLE_ID_XS_CAN=44;PROPERTY_VALUE_DONGLE_ID_LIN=45;PROPERTY_VALUE_DONGLE_ID_DONGLE_LESS=46;PROPERTY_VALUE_DONGLE_ID_UNKNOWN=47;PROPERTY_VALUE_CAN_TERM_OFF=48;PROPERTY_VALUE_CAN_TERM_ON=49;PROPERTY_VALUE_CAN_TCVR_STATE_NORMAL=50;PROPERTY_VALUE_CAN_TCVR_STATE_SLEEP=51;PROPERTY_VALUE_CAN_TCVR_STATE_SW_WAKEUP=52;PROPERTY_VALUE_CAN_TCVR_STATE_SW_HIGH_SPEED=53;PROPERTY_VALUE_CAN_TCVR_TYPE_HS=54;PROPERTY_VALUE_CAN_TCVR_TYPE_LS=55;PROPERTY_VALUE_CAN_TCVR_TYPE_SW=56;PROPERTY_VALUE_CAN_TCVR_TYPE_EXT=57;PROPERTY_VALUE_CAN_TCVR_TYPE_DISC=58;PROPERTY_VALUE_FLEX_RAY_SAMP_PER_MICRO_1=59;PROPERTY_VALUE_FLEX_RAY_SAMP_PER_MICRO_2=60;PROPERTY_VALUE_FLEX_RAY_SAMP_PER_MICRO_4=61;PROPERTY_VALUE_FLEX_RAY_TERM_OFF=62;PROPERTY_VALUE_FLEX_RAY_TERM_ON=63;PROPERTY_VALUE_LIN_SLEEP_REMOTE_SLEEP=64;PROPERTY_VALUE_LIN_SLEEP_REMOTE_WAKE=65;PROPERTY_VALUE_LIN_SLEEP_LOCAL_SLEEP=66;PROPERTY_VALUE_LIN_SLEEP_LOCAL_WAKE=67;PROPERTY_VALUE_LIN_TERM_OFF=68;PROPERTY_VALUE_LIN_TERM_ON=69;PROPERTY_VALUE_OUT_STRM_TIMNG_IMMEDIATE=70;PROPERTY_VALUE_OUT_STRM_TIMNG_REPLAY_EXCLUSIVE=71;PROPERTY_VALUE_OUT_STRM_TIMNG_REPLAY_INCLUSIVE=72;PROPERTY_VALUE_CAN_PEND_TX_ORDER_AS_SUBMITTED=73;PROPERTY_VALUE_CAN_PEND_TX_ORDER_BY_IDENTIFIER=74;PROPERTY_VALUE_FLEX_RAY_SLEEP_LOCAL_SLEEP=75;PROPERTY_VALUE_FLEX_RAY_SLEEP_LOCAL_WAKE=76;PROPERTY_VALUE_FLEX_RAY_SLEEP_REMOTE_WAKE=77;PROPERTY_VALUE_CAN_EXT_TCVR_CONFIG_NORMAL_SUPPORTED=78;PROPERTY_VALUE_CAN_EXT_TCVR_CONFIG_SLEEP_SUPPORTED=79;PROPERTY_VALUE_CAN_EXT_TCVR_CONFIG_SW_WAKEUP_SUPPORTED=80;PROPERTY_VALUE_CAN_EXT_TCVR_CONFIG_SW_HIGH_SPEED_SUPPORTED=81;PROPERTY_VALUE_CAN_EXT_TCVR_CONFIG_POWER_ON_SUPPORTED=82;PROPERTY_VALUE_CAN_EXT_TCVR_CONFIG_NORMAL_OUTPUT_0_SET=83;PROPERTY_VALUE_CAN_EXT_TCVR_CONFIG_SLEEP_OUTPUT_0_SET=84;PROPERTY_VALUE_CAN_EXT_TCVR_CONFIG_SW_WAKEUP_OUTPUT_0_SET=85;PROPERTY_VALUE_CAN_EXT_TCVR_CONFIG_SW_HIGH_SPEED_OUTPUT_0_SET=86;PROPERTY_VALUE_CAN_EXT_TCVR_CONFIG_POWER_ON_OUTPUT_0_SET=87;PROPERTY_VALUE_CAN_EXT_TCVR_CONFIG_NORMAL_OUTPUT_1_SET=88;PROPERTY_VALUE_CAN_EXT_TCVR_CONFIG_SLEEP_OUTPUT_1_SET=89;PROPERTY_VALUE_CAN_EXT_TCVR_CONFIG_SW_WAKEUP_OUTPUT_1_SET=90;PROPERTY_VALUE_CAN_EXT_TCVR_CONFIG_SW_HIGH_SPEED_OUTPUT_1_SET=91;PROPERTY_VALUE_CAN_EXT_TCVR_CONFIG_POWER_ON_OUTPUT_1_SET=92;PROPERTY_VALUE_CAN_EXT_TCVR_CONFIG_N_ERR_CONNECTED=93;PROPERTY_VALUE_ENET_PORT_MODE_DIRECT=94;PROPERTY_VALUE_ENET_PORT_MODE_TAP=95;PROPERTY_VALUE_ENET_PHY_STATE_SLAVE=96;PROPERTY_VALUE_ENET_PHY_STATE_MASTER=97;PROPERTY_VALUE_ENET_PHY_STATE_AUTO=98;PROPERTY_VALUE_ENET_LINK_SPEED_LINK_DOWN=99;PROPERTY_VALUE_ENET_LINK_SPEED_100_MBPS=100;PROPERTY_VALUE_ENET_LINK_SPEED_1000_MBPS=101;PROPERTY_VALUE_ENET_JUMBO_FRAMES_DISABLED=102;PROPERTY_VALUE_ENET_JUMBO_FRAMES_9018_BYTES=103;PROPERTY_VALUE_ENET_OPERATIONAL_STATUS_DOWN=104;PROPERTY_VALUE_ENET_OPERATIONAL_STATUS_UP=105;PROPERTY_VALUE_ENET_LOG_MODE_OFF=106;PROPERTY_VALUE_ENET_LOG_MODE_LOG=107;PROPERTY_VALUE_ENET_LOG_OPERATION_CREATE_OR_REPLACE=108;PROPERTY_VALUE_ENET_LOG_OPERATION_CREATE=109;PROPERTY_VALUE_ENET_TIME_PROTOCOL_IEEE_8021AS=110;PROPERTY_VALUE_ENET_TIME_CLK_ACCURACY_WITHIN_25NSEC=111;PROPERTY_VALUE_ENET_TIME_CLK_ACCURACY_WITHIN_100NSEC=112;PROPERTY_VALUE_ENET_TIME_CLK_ACCURACY_WITHIN_250NSEC=113;PROPERTY_VALUE_ENET_TIME_CLK_ACCURACY_WITHIN_1USEC=114;PROPERTY_VALUE_ENET_TIME_CLK_ACCURACY_WITHIN_2500NSEC=115;PROPERTY_VALUE_ENET_TIME_CLK_ACCURACY_WITHIN_10USEC=116;PROPERTY_VALUE_ENET_TIME_CLK_ACCURACY_WITHIN_25USEC=117;PROPERTY_VALUE_ENET_TIME_CLK_ACCURACY_WITHIN_100USEC=118;PROPERTY_VALUE_ENET_TIME_CLK_ACCURACY_WITHIN_250USEC=119;PROPERTY_VALUE_ENET_TIME_CLK_ACCURACY_WITHIN_1MSEC=120;PROPERTY_VALUE_ENET_TIME_CLK_ACCURACY_WITHIN_2500USEC=121;PROPERTY_VALUE_ENET_TIME_CLK_ACCURACY_WITHIN_10MSEC=122;PROPERTY_VALUE_ENET_TIME_CLK_ACCURACY_WITHIN_25MSEC=123;PROPERTY_VALUE_ENET_TIME_CLK_ACCURACY_WITHIN_100MSEC=124;PROPERTY_VALUE_ENET_TIME_CLK_ACCURACY_WITHIN_250MSEC=125;PROPERTY_VALUE_ENET_TIME_CLK_ACCURACY_WITHIN_1SEC=126;PROPERTY_VALUE_ENET_TIME_CLK_ACCURACY_WITHIN_10SEC=127;PROPERTY_VALUE_ENET_TIME_CLK_ACCURACY_GREATHER_THAN_10SEC=128;PROPERTY_VALUE_ENET_TIME_CLK_ACCURACY_UNKNOWN=129;PROPERTY_VALUE_ENET_TIME_PORT_SYNC_STATUS_SYNCED=130;PROPERTY_VALUE_ENET_TIME_PORT_SYNC_STATUS_ENET_LINK_DOWN=131;PROPERTY_VALUE_ENET_TIME_PORT_SYNC_STATUS_PROTOCOL_DISABLED=132;PROPERTY_VALUE_ENET_TIME_PORT_SYNC_STATUS_MEASURING_PROP_DELAY=133;PROPERTY_VALUE_ENET_TIME_PORT_SYNC_STATUS_MASTER_PENDING_ANNOUNCE=134;PROPERTY_VALUE_ENET_TIME_PORT_SYNC_STATUS_WAITING_FOR_MASTER=135;PROPERTY_VALUE_ENET_TIME_PORT_SYNC_STATUS_SYNCING_TO_MASTER=136;PROPERTY_VALUE_ENET_TIME_PORT_SYNC_STATUS_PEER_NOT_PROTO_CAPABLE=137;PROPERTY_VALUE_ENET_TIME_PORT_SYNC_STATUS_PROP_DELAY_EXCEEDS_TRESHOLD=138;PROPERTY_VALUE_ENET_TIME_PORT_SYNC_STATUS_SYNC_RECEIPT_TIMEOUT=139;PROPERTY_VALUE_ENET_TIME_PORT_SYNC_STATUS_FREQUENCY_OUT_OF_RANGE=140;PROPERTY_VALUE_ENET_TIME_PORT_SYNC_STATUS_SYNC_INTERVAL_OUT_OF_RANGE=141;PROPERTY_VALUE_ENET_TIME_PORT_SYNC_STATUS_MULTIPLE_MASTERS_DETECTED=142;PROPERTY_VALUE_ENET_TIME_PORT_STATE_DISABLED=143;PROPERTY_VALUE_ENET_TIME_PORT_STATE_MASTER=144;PROPERTY_VALUE_ENET_TIME_PORT_STATE_PASSIVE=145;PROPERTY_VALUE_ENET_TIME_PORT_STATE_SLAVE=146;PROPERTY_VALUE_ENET_TIME_P_DELAY_REQ_INTERVAL_125MS=147;PROPERTY_VALUE_ENET_TIME_P_DELAY_REQ_INTERVAL_250MS=148;PROPERTY_VALUE_ENET_TIME_P_DELAY_REQ_INTERVAL_500MS=149;PROPERTY_VALUE_ENET_TIME_P_DELAY_REQ_INTERVAL_1S=150;PROPERTY_VALUE_ENET_TIME_P_DELAY_REQ_INTERVAL_2S=151;PROPERTY_VALUE_ENET_TIME_SYNC_INTERVAL_125MS=152;PROPERTY_VALUE_ENET_TIME_SYNC_INTERVAL_250MS=153;PROPERTY_VALUE_ENET_TIME_SYNC_INTERVAL_500MS=154;PROPERTY_VALUE_ENET_TIME_SYNC_INTERVAL_1S=155;PROPERTY_VALUE_ENET_TIME_SYNC_INTERVAL_2S=156;PROPERTY_VALUE_ENET_TIME_ANNOUNCE_INTERVAL_125MS=157;PROPERTY_VALUE_ENET_TIME_ANNOUNCE_INTERVAL_250MS=158;PROPERTY_VALUE_ENET_TIME_ANNOUNCE_INTERVAL_500MS=159;PROPERTY_VALUE_ENET_TIME_ANNOUNCE_INTERVAL_1S=160;PROPERTY_VALUE_ENET_TIME_ANNOUNCE_INTERVAL_2S=161;PROPERTY_VALUE_ENET_SLEEP_CAPABILITY_DISABLED_OR_NOT_AVAILABLE=162;PROPERTY_VALUE_ENET_SLEEP_CAPABILITY_ENABLED=163;PROPERTY_VALUE_ENET_PHY_POWER_MODE_NORMAL=164;PROPERTY_VALUE_ENET_PHY_POWER_MODE_SLEEP=165", "Allow Alias"=FALSE}, {"Version"=2, "Name"="nixnet_grpc_ReadState", "Type Url"="nixnet_grpc.ReadState", "Enum Values"="READ_STATE_UNSPECIFIED=0;READ_STATE_TIME_CURRENT=118685697;READ_STATE_TIME_COMMUNICATING=118685698;READ_STATE_TIME_START=118685699;READ_STATE_SESSION_INFO=1245188;READ_STATE_TIME_CURRENT_2=202571781;READ_STATE_TIME_COMMUNICATING_2=202571782;READ_STATE_TIME_START_2=202571783;READ_STATE_CAN_COMM=1245200;READ_STATE_FLEX_RAY_COMM=1245216;READ_STATE_FLEX_RAY_STATS=135462945;READ_STATE_LIN_COMM=1245232;READ_STATE_J1939_COMM=1245248", "Allow Alias"=FALSE}, {"Version"=2, "Name"="nixnet_grpc_SessionInfoState", "Type Url"="nixnet_grpc.SessionInfoState", "Enum Values"="SESSION_INFO_STATE_STOPPED=0;SESSION_INFO_STATE_STARTED=1;SESSION_INFO_STATE_MIX=2", "Allow Alias"=FALSE}, {"Version"=2, "Name"="nixnet_grpc_StartStopScope", "Type Url"="nixnet_grpc.StartStopScope", "Enum Values"="START_STOP_SCOPE_NORMAL=0;START_STOP_SCOPE_SESSION_ONLY=1;START_STOP_SCOPE_INTERFACE_ONLY=2;START_STOP_SCOPE_SESSION_ONLY_BLOCKING=3", "Allow Alias"=FALSE}, {"Version"=2, "Name"="nixnet_grpc_SubProperty", "Type Url"="nixnet_grpc.SubProperty", "Enum Values"="SUB_PROPERTY_UNSPECIFIED=0;SUB_PROPERTY_SESSION_SUB_CAN_START_TIME_OFF=17825921;SUB_PROPERTY_SESSION_SUB_CAN_TX_TIME=17825922;SUB_PROPERTY_SESSION_SUB_LIN_TX_N_CORRUPTED_CHKSUMS=1048709;SUB_PROPERTY_SESSION_SUB_OUTPUT_QUEUE_UPDATE_FREQ=1048708;SUB_PROPERTY_SESSION_SUB_J1939_ADDR_FILTER=51380358;SUB_PROPERTY_SESSION_SUB_SKIP_N_CYCLIC_FRAMES=1048707", "Allow Alias"=FALSE}, {"Version"=2, "Name"="nixnet_grpc_SubPropertyValue", "Type Url"="nixnet_grpc.SubPropertyValue", "Enum Values"="SUB_PROPERTY_VALUE_FRM_FLEX_RAY_TIMING_CYCLIC=0;SUB_PROPERTY_VALUE_FRM_FLEX_RAY_CH_ASSIGN_A=1;SUB_PROPERTY_VALUE_FRM_FLEX_RAY_CH_ASSIGN_B=2;SUB_PROPERTY_VALUE_FRM_FLEX_RAY_CH_ASSIGN_A_AND_B=3;SUB_PROPERTY_VALUE_FRM_FLEX_RAY_CH_ASSIGN_NONE=4;SUB_PROPERTY_VALUE_FRM_FLEX_RAY_TIMING_EVENT=1;SUB_PROPERTY_VALUE_FRM_CAN_TIMING_CYCLIC_DATA=0;SUB_PROPERTY_VALUE_FRM_CAN_TIMING_EVENT_DATA=1;SUB_PROPERTY_VALUE_FRM_CAN_TIMING_CYCLIC_REMOTE=2;SUB_PROPERTY_VALUE_FRM_CAN_TIMING_EVENT_REMOTE=3;SUB_PROPERTY_VALUE_FRM_CAN_TIMING_CYCLIC_EVENT=4;SUB_PROPERTY_VALUE_FRM_LIN_CHECKSUM_CLASSIC=0;SUB_PROPERTY_VALUE_FRM_LIN_CHECKSUM_ENHANCED=1", "Allow Alias"=TRUE}, {"Version"=2, "Name"="nixnet_grpc_TerminalName", "Type Url"="nixnet_grpc.TerminalName", "Enum Values"="TERMINAL_NAME_UNSPECIFIED=0;TERMINAL_NAME_PXI_TRIG_0=1;TERMINAL_NAME_PXI_TRIG_1=2;TERMINAL_NAME_PXI_TRIG_2=3;TERMINAL_NAME_PXI_TRIG_3=4;TERMINAL_NAME_PXI_TRIG_4=5;TERMINAL_NAME_PXI_TRIG_5=6;TERMINAL_NAME_PXI_TRIG_6=7;TERMINAL_NAME_PXI_TRIG_7=8;TERMINAL_NAME_FRONT_PANEL_0=9;TERMINAL_NAME_FRONT_PANEL_1=10;TERMINAL_NAME_PXI_STAR=11;TERMINAL_NAME_PXI_CLK_10=12;TERMINAL_NAME_10_MHZ_TIMEBASE=13;TERMINAL_NAME_1_MHZ_TIMEBASE=14;TERMINAL_NAME_MASTER_TIMEBASE=15;TERMINAL_NAME_COMM_TRIGGER=16;TERMINAL_NAME_START_TRIGGER=17;TERMINAL_NAME_FLEX_RAY_START_CYCLE=18;TERMINAL_NAME_FLEX_RAY_MACROTICK=19;TERMINAL_NAME_LOG_TRIGGER=20;TERMINAL_NAME_TIME_TRIGGER=21;TERMINAL_NAME_NETWORK_TIME_PPS=22;TERMINAL_NAME_NETWORK_TIME_1_MHZ=23", "Allow Alias"=FALSE}, {"Version"=2, "Name"="nixnet_grpc_TimeOut", "Type Url"="nixnet_grpc.TimeOut", "Enum Values"="TIME_OUT_NONE=0;TIME_OUT_INFINITE=-1", "Allow Alias"=FALSE}, {"Version"=2, "Name"="nixnet_grpc_TimeScale", "Type Url"="nixnet_grpc.TimeScale", "Enum Values"="TIME_SCALE_LOCAL_TIME=0;TIME_SCALE_NETWORK_TIME=1", "Allow Alias"=FALSE}, {"Version"=2, "Name"="nixnet_grpc_WaitCondition", "Type Url"="nixnet_grpc.WaitCondition", "Enum Values"="WAIT_CONDITION_UNSPECIFIED=0;WAIT_CONDITION_TRANSMIT_COMPLETE=32769;WAIT_CONDITION_INTF_COMMUNICATING=32770;WAIT_CONDITION_INTF_REMOTE_WAKEUP=32771;WAIT_CONDITION_ETHERNET_SYNCED=32772", "Allow Alias"=FALSE}, {"Version"=2, "Name"="nixnet_grpc_WriteState", "Type Url"="nixnet_grpc.WriteState", "Enum Values"="WRITE_STATE_UNSPECIFIED=0;WRITE_STATE_LIN_SCHEDULE_CHANGE=1245313;WRITE_STATE_LIN_DIAGNOSTIC_SCHEDULE_CHANGE=1245315;WRITE_STATE_FLEX_RAY_SYMBOL=1245314;WRITE_STATE_ETHERNET_SLEEP=1245316;WRITE_STATE_ETHERNET_WAKE=1245317", "Allow Alias"=FALSE}, {"Version"=2, "Name"="nixnet_grpc_Protocol", "Type Url"="nixnet_grpc.Protocol", "Enum Values"="PROTOCOL_UNSPECIFIED=0;PROTOCOL_CAN=1;PROTOCOL_LIN=2;PROTOCOL_FLEX_RAY=3;PROTOCOL_J1939=4;PROTOCOL_ENET=5", "Allow Alias"=FALSE}, {"Version"=2, "Name"="nidevice_grpc_SessionInitializationBehavior", "Type Url"="nidevice_grpc.SessionInitializationBehavior", "Enum Values"="SESSION_INITIALIZATION_BEHAVIOR_UNSPECIFIED=0;SESSION_INITIALIZATION_BEHAVIOR_INITIALIZE_NEW=1;SESSION_INITIALIZATION_BEHAVIOR_ATTACH_TO_EXISTING=2", "Allow Alias"=FALSE}]  # Enum MetaData
      w11 = T3[] [{"Version"=2, "Name"="nixnet_grpc_FlexRayStats", "Type Url"="nixnet_grpc.FlexRayStats", "Elements"=[{"Field Name"="num_syntax_error_ch_a", "Embedded Message Name"="", "Protobuf Index"=1, "MessageElementType"=enum."UInt32Value", "Repeated"=FALSE, "Is in Oneof"=FALSE, "Oneof Container Name"=""}, {"Field Name"="num_syntax_error_ch_b", "Embedded Message Name"="", "Protobuf Index"=2, "MessageElementType"=enum."UInt32Value", "Repeated"=FALSE, "Is in Oneof"=FALSE, "Oneof Container Name"=""}, {"Field Name"="num_content_error_ch_a", "Embedded Message Name"="", "Protobuf Index"=3, "MessageElementType"=enum."UInt32Value", "Repeated"=FALSE, "Is in Oneof"=FALSE, "Oneof Container Name"=""}, {"Field Name"="num_content_error_ch_b", "Embedded Message Name"="", "Protobuf Index"=4, "MessageElementType"=enum."UInt32Value", "Repeated"=FALSE, "Is in Oneof"=FALSE, "Oneof Container Name"=""}, {"Field Name"="num_slot_boundary_violation_ch_a", "Embedded Message Name"="", "Protobuf Index"=5, "MessageElementType"=enum."UInt32Value", "Repeated"=FALSE, "Is in Oneof"=FALSE, "Oneof Container Name"=""}, {"Field Name"="num_slot_boundary_violation_ch_b", "Embedded Message Name"="", "Protobuf Index"=6, "MessageElementType"=enum."UInt32Value", "Repeated"=FALSE, "Is in Oneof"=FALSE, "Oneof Container Name"=""}], "Has Oneof"=FALSE}, {"Version"=2, "Name"="nixnet_grpc_J1939CommState", "Type Url"="nixnet_grpc.J1939CommState", "Elements"=[{"Field Name"="pgn", "Embedded Message Name"="", "Protobuf Index"=1, "MessageElementType"=enum."UInt32Value", "Repeated"=FALSE, "Is in Oneof"=FALSE, "Oneof Container Name"=""}, {"Field Name"="source_address", "Embedded Message Name"="", "Protobuf Index"=2, "MessageElementType"=enum."UInt32Value", "Repeated"=FALSE, "Is in Oneof"=FALSE, "Oneof Container Name"=""}, {"Field Name"="destination_address", "Embedded Message Name"="", "Protobuf Index"=3, "MessageElementType"=enum."UInt32Value", "Repeated"=FALSE, "Is in Oneof"=FALSE, "Oneof Container Name"=""}, {"Field Name"="transmit_error", "Embedded Message Name"="", "Protobuf Index"=4, "MessageElementType"=enum."UInt32Value", "Repeated"=FALSE, "Is in Oneof"=FALSE, "Oneof Container Name"=""}, {"Field Name"="receive_error", "Embedded Message Name"="", "Protobuf Index"=5, "MessageElementType"=enum."UInt32Value", "Repeated"=FALSE, "Is in Oneof"=FALSE, "Oneof Container Name"=""}], "Has Oneof"=FALSE}, {"Version"=2, "Name"="nixnet_grpc_CanCommResponse", "Type Url"="nixnet_grpc.CanCommResponse", "Elements"=[{"Field Name"="comm_state", "Embedded Message Name"="nixnet_grpc_CanCommState", "Protobuf Index"=1, "MessageElementType"=enum."EnumValue", "Repeated"=FALSE, "Is in Oneof"=FALSE, "Oneof Container Name"=""}, {"Field Name"="comm_state_raw", "Embedded Message Name"="", "Protobuf Index"=2, "MessageElementType"=enum."UInt32Value", "Repeated"=FALSE, "Is in Oneof"=FALSE, "Oneof Container Name"=""}, {"Field Name"="transceiver_error", "Embedded Message Name"="", "Protobuf Index"=3, "MessageElementType"=enum."UInt32Value", "Repeated"=FALSE, "Is in Oneof"=FALSE, "Oneof Container Name"=""}, {"Field Name"="sleep", "Embedded Message Name"="", "Protobuf Index"=4, "MessageElementType"=enum."UInt32Value", "Repeated"=FALSE, "Is in Oneof"=FALSE, "Oneof Container Name"=""}, {"Field Name"="last_error", "Embedded Message Name"="nixnet_grpc_CanLastErr", "Protobuf Index"=5, "MessageElementType"=enum."EnumValue", "Repeated"=FALSE, "Is in Oneof"=FALSE, "Oneof Container Name"=""}, {"Field Name"="last_error_raw", "Embedded Message Name"="", "Protobuf Index"=6, "MessageElementType"=enum."UInt32Value", "Repeated"=FALSE, "Is in Oneof"=FALSE, "Oneof Container Name"=""}, {"Field Name"="transmit_error_counter", "Embedded Message Name"="", "Protobuf Index"=7, "MessageElementType"=enum."UInt32Value", "Repeated"=FALSE, "Is in Oneof"=FALSE, "Oneof Container Name"=""}, {"Field Name"="receive_error_counter", "Embedded Message Name"="", "Protobuf Index"=8, "MessageElementType"=enum."UInt32Value", "Repeated"=FALSE, "Is in Oneof"=FALSE, "Oneof Container Name"=""}], "Has Oneof"=FALSE}, {"Version"=2, "Name"="nixnet_grpc_FlexRayCommResponse", "Type Url"="nixnet_grpc.FlexRayCommResponse", "Elements"=[{"Field Name"="poc_state", "Embedded Message Name"="nixnet_grpc_FlexRayPocState", "Protobuf Index"=1, "MessageElementType"=enum."EnumValue", "Repeated"=FALSE, "Is in Oneof"=FALSE, "Oneof Container Name"=""}, {"Field Name"="poc_state_raw", "Embedded Message Name"="", "Protobuf Index"=2, "MessageElementType"=enum."UInt32Value", "Repeated"=FALSE, "Is in Oneof"=FALSE, "Oneof Container Name"=""}, {"Field Name"="clock_correction_failed", "Embedded Message Name"="", "Protobuf Index"=3, "MessageElementType"=enum."UInt32Value", "Repeated"=FALSE, "Is in Oneof"=FALSE, "Oneof Container Name"=""}, {"Field Name"="passive_to_active_count", "Embedded Message Name"="", "Protobuf Index"=4, "MessageElementType"=enum."UInt32Value", "Repeated"=FALSE, "Is in Oneof"=FALSE, "Oneof Container Name"=""}, {"Field Name"="channel_a_sleep", "Embedded Message Name"="", "Protobuf Index"=5, "MessageElementType"=enum."UInt32Value", "Repeated"=FALSE, "Is in Oneof"=FALSE, "Oneof Container Name"=""}, {"Field Name"="channel_b_sleep", "Embedded Message Name"="", "Protobuf Index"=6, "MessageElementType"=enum."UInt32Value", "Repeated"=FALSE, "Is in Oneof"=FALSE, "Oneof Container Name"=""}], "Has Oneof"=FALSE}, {"Version"=2, "Name"="nixnet_grpc_LinCommResponse", "Type Url"="nixnet_grpc.LinCommResponse", "Elements"=[{"Field Name"="sleep", "Embedded Message Name"="", "Protobuf Index"=1, "MessageElementType"=enum."UInt32Value", "Repeated"=FALSE, "Is in Oneof"=FALSE, "Oneof Container Name"=""}, {"Field Name"="comm_state", "Embedded Message Name"="nixnet_grpc_LinCommState", "Protobuf Index"=2, "MessageElementType"=enum."EnumValue", "Repeated"=FALSE, "Is in Oneof"=FALSE, "Oneof Container Name"=""}, {"Field Name"="comm_state_raw", "Embedded Message Name"="", "Protobuf Index"=3, "MessageElementType"=enum."UInt32Value", "Repeated"=FALSE, "Is in Oneof"=FALSE, "Oneof Container Name"=""}, {"Field Name"="last_error", "Embedded Message Name"="", "Protobuf Index"=4, "MessageElementType"=enum."UInt32Value", "Repeated"=FALSE, "Is in Oneof"=FALSE, "Oneof Container Name"=""}, {"Field Name"="last_error_received", "Embedded Message Name"="", "Protobuf Index"=5, "MessageElementType"=enum."UInt32Value", "Repeated"=FALSE, "Is in Oneof"=FALSE, "Oneof Container Name"=""}, {"Field Name"="last_error_expected", "Embedded Message Name"="", "Protobuf Index"=6, "MessageElementType"=enum."UInt32Value", "Repeated"=FALSE, "Is in Oneof"=FALSE, "Oneof Container Name"=""}, {"Field Name"="last_error_id", "Embedded Message Name"="", "Protobuf Index"=7, "MessageElementType"=enum."UInt32Value", "Repeated"=FALSE, "Is in Oneof"=FALSE, "Oneof Container Name"=""}, {"Field Name"="transceiver_ready", "Embedded Message Name"="", "Protobuf Index"=8, "MessageElementType"=enum."UInt32Value", "Repeated"=FALSE, "Is in Oneof"=FALSE, "Oneof Container Name"=""}, {"Field Name"="schedule_index", "Embedded Message Name"="", "Protobuf Index"=9, "MessageElementType"=enum."UInt32Value", "Repeated"=FALSE, "Is in Oneof"=FALSE, "Oneof Container Name"=""}], "Has Oneof"=FALSE}, {"Version"=2, "Name"="nixnet_grpc_SessionInfoResponse", "Type Url"="nixnet_grpc.SessionInfoResponse", "Elements"=[{"Field Name"="info", "Embedded Message Name"="nixnet_grpc_SessionInfoState", "Protobuf Index"=1, "MessageElementType"=enum."EnumValue", "Repeated"=FALSE, "Is in Oneof"=FALSE, "Oneof Container Name"=""}, {"Field Name"="info_raw", "Embedded Message Name"="", "Protobuf Index"=2, "MessageElementType"=enum."UInt32Value", "Repeated"=FALSE, "Is in Oneof"=FALSE, "Oneof Container Name"=""}], "Has Oneof"=FALSE}, {"Version"=2, "Name"="nixnet_grpc_ReadStateValue", "Type Url"="nixnet_grpc.ReadStateValue", "Elements"=[{"Field Name"="selected_index", "Embedded Message Name"="", "Protobuf Index"=-1, "MessageElementType"=enum."Int32Value", "Repeated"=FALSE, "Is in Oneof"=TRUE, "Oneof Container Name"="nixnet_grpc_ReadStateValue_value"}, {"Field Name"="time_current", "Embedded Message Name"="", "Protobuf Index"=1, "MessageElementType"=enum."UInt64Value", "Repeated"=FALSE, "Is in Oneof"=TRUE, "Oneof Container Name"="nixnet_grpc_ReadStateValue_value"}, {"Field Name"="time_communicating", "Embedded Message Name"="", "Protobuf Index"=2, "MessageElementType"=enum."UInt64Value", "Repeated"=FALSE, "Is in Oneof"=TRUE, "Oneof Container Name"="nixnet_grpc_ReadStateValue_value"}, {"Field Name"="time_start", "Embedded Message Name"="", "Protobuf Index"=3, "MessageElementType"=enum."UInt64Value", "Repeated"=FALSE, "Is in Oneof"=TRUE, "Oneof Container Name"="nixnet_grpc_ReadStateValue_value"}, {"Field Name"="can_comm", "Embedded Message Name"="nixnet_grpc_CanCommResponse", "Protobuf Index"=4, "MessageElementType"=enum."MessageValue", "Repeated"=FALSE, "Is in Oneof"=TRUE, "Oneof Container Name"="nixnet_grpc_ReadStateValue_value"}, {"Field Name"="flex_ray_comm", "Embedded Message Name"="nixnet_grpc_FlexRayCommResponse", "Protobuf Index"=5, "MessageElementType"=enum."MessageValue", "Repeated"=FALSE, "Is in Oneof"=TRUE, "Oneof Container Name"="nixnet_grpc_ReadStateValue_value"}, {"Field Name"="flex_ray_stats", "Embedded Message Name"="nixnet_grpc_FlexRayStats", "Protobuf Index"=6, "MessageElementType"=enum."MessageValue", "Repeated"=FALSE, "Is in Oneof"=TRUE, "Oneof Container Name"="nixnet_grpc_ReadStateValue_value"}, {"Field Name"="lin_comm", "Embedded Message Name"="nixnet_grpc_LinCommResponse", "Protobuf Index"=7, "MessageElementType"=enum."MessageValue", "Repeated"=FALSE, "Is in Oneof"=TRUE, "Oneof Container Name"="nixnet_grpc_ReadStateValue_value"}, {"Field Name"="session_info", "Embedded Message Name"="nixnet_grpc_SessionInfoResponse", "Protobuf Index"=8, "MessageElementType"=enum."MessageValue", "Repeated"=FALSE, "Is in Oneof"=TRUE, "Oneof Container Name"="nixnet_grpc_ReadStateValue_value"}, {"Field Name"="j1939_comm_state", "Embedded Message Name"="nixnet_grpc_J1939CommState", "Protobuf Index"=9, "MessageElementType"=enum."MessageValue", "Repeated"=FALSE, "Is in Oneof"=TRUE, "Oneof Container Name"="nixnet_grpc_ReadStateValue_value"}, {"Field Name"="time_current2", "Embedded Message Name"="nixnet_grpc_TimeLocalNetwork", "Protobuf Index"=10, "MessageElementType"=enum."MessageValue", "Repeated"=FALSE, "Is in Oneof"=TRUE, "Oneof Container Name"="nixnet_grpc_ReadStateValue_value"}, {"Field Name"="time_communicating2", "Embedded Message Name"="nixnet_grpc_TimeLocalNetwork", "Protobuf Index"=11, "MessageElementType"=enum."MessageValue", "Repeated"=FALSE, "Is in Oneof"=TRUE, "Oneof Container Name"="nixnet_grpc_ReadStateValue_value"}, {"Field Name"="time_start2", "Embedded Message Name"="nixnet_grpc_TimeLocalNetwork", "Protobuf Index"=12, "MessageElementType"=enum."MessageValue", "Repeated"=FALSE, "Is in Oneof"=TRUE, "Oneof Container Name"="nixnet_grpc_ReadStateValue_value"}, {"Field Name"="state_value_raw", "Embedded Message Name"="", "Protobuf Index"=13, "MessageElementType"=enum."Bytes", "Repeated"=FALSE, "Is in Oneof"=FALSE, "Oneof Container Name"=""}], "Has Oneof"=TRUE}, {"Version"=2, "Name"="nixnet_grpc_LinDiagnosticScheduleChangeRequest", "Type Url"="nixnet_grpc.LinDiagnosticScheduleChangeRequest", "Elements"=[{"Field Name"="selected_index", "Embedded Message Name"="", "Protobuf Index"=-1, "MessageElementType"=enum."Int32Value", "Repeated"=FALSE, "Is in Oneof"=TRUE, "Oneof Container Name"="nixnet_grpc_LinDiagnosticScheduleChangeRequest_schedule_enum"}, {"Field Name"="schedule", "Embedded Message Name"="nixnet_grpc_LinDiagnosticSchedule", "Protobuf Index"=1, "MessageElementType"=enum."EnumValue", "Repeated"=FALSE, "Is in Oneof"=TRUE, "Oneof Container Name"="nixnet_grpc_LinDiagnosticScheduleChangeRequest_schedule_enum"}, {"Field Name"="schedule_raw", "Embedded Message Name"="", "Protobuf Index"=2, "MessageElementType"=enum."UInt32Value", "Repeated"=FALSE, "Is in Oneof"=TRUE, "Oneof Container Name"="nixnet_grpc_LinDiagnosticScheduleChangeRequest_schedule_enum"}], "Has Oneof"=TRUE}, {"Version"=2, "Name"="nixnet_grpc_WriteStateValue", "Type Url"="nixnet_grpc.WriteStateValue", "Elements"=[{"Field Name"="selected_index", "Embedded Message Name"="", "Protobuf Index"=-1, "MessageElementType"=enum."Int32Value", "Repeated"=FALSE, "Is in Oneof"=TRUE, "Oneof Container Name"="nixnet_grpc_WriteStateValue_value"}, {"Field Name"="lin_schedule_change", "Embedded Message Name"="", "Protobuf Index"=1, "MessageElementType"=enum."UInt32Value", "Repeated"=FALSE, "Is in Oneof"=TRUE, "Oneof Container Name"="nixnet_grpc_WriteStateValue_value"}, {"Field Name"="flex_ray_symbol", "Embedded Message Name"="", "Protobuf Index"=2, "MessageElementType"=enum."UInt32Value", "Repeated"=FALSE, "Is in Oneof"=TRUE, "Oneof Container Name"="nixnet_grpc_WriteStateValue_value"}, {"Field Name"="lin_diagnostic_schedule_change", "Embedded Message Name"="nixnet_grpc_LinDiagnosticScheduleChangeRequest", "Protobuf Index"=3, "MessageElementType"=enum."MessageValue", "Repeated"=FALSE, "Is in Oneof"=TRUE, "Oneof Container Name"="nixnet_grpc_WriteStateValue_value"}, {"Field Name"="ethernet_sleep", "Embedded Message Name"="", "Protobuf Index"=4, "MessageElementType"=enum."UInt32Value", "Repeated"=FALSE, "Is in Oneof"=TRUE, "Oneof Container Name"="nixnet_grpc_WriteStateValue_value"}, {"Field Name"="ethernet_wake", "Embedded Message Name"="", "Protobuf Index"=5, "MessageElementType"=enum."UInt32Value", "Repeated"=FALSE, "Is in Oneof"=TRUE, "Oneof Container Name"="nixnet_grpc_WriteStateValue_value"}], "Has Oneof"=TRUE}, {"Version"=2, "Name"="nixnet_grpc_U32Array", "Type Url"="nixnet_grpc.U32Array", "Elements"=[{"Field Name"="u32_array", "Embedded Message Name"="", "Protobuf Index"=1, "MessageElementType"=enum."UInt32Value", "Repeated"=TRUE, "Is in Oneof"=FALSE, "Oneof Container Name"=""}], "Has Oneof"=FALSE}, {"Version"=2, "Name"="nixnet_grpc_DbRefArray", "Type Url"="nixnet_grpc.DbRefArray", "Elements"=[{"Field Name"="db_ref", "Embedded Message Name"="nidevice_grpc_Session", "Protobuf Index"=1, "MessageElementType"=enum."MessageValue", "Repeated"=TRUE, "Is in Oneof"=FALSE, "Oneof Container Name"=""}], "Has Oneof"=FALSE}, {"Version"=2, "Name"="nixnet_grpc_DeviceRefArray", "Type Url"="nixnet_grpc.DeviceRefArray", "Elements"=[{"Field Name"="dev_ref", "Embedded Message Name"="nidevice_grpc_Session", "Protobuf Index"=1, "MessageElementType"=enum."MessageValue", "Repeated"=TRUE, "Is in Oneof"=FALSE, "Oneof Container Name"=""}], "Has Oneof"=FALSE}, {"Version"=2, "Name"="nixnet_grpc_InterfaceRefArray", "Type Url"="nixnet_grpc.InterfaceRefArray", "Elements"=[{"Field Name"="intf_ref", "Embedded Message Name"="nidevice_grpc_Session", "Protobuf Index"=1, "MessageElementType"=enum."MessageValue", "Repeated"=TRUE, "Is in Oneof"=FALSE, "Oneof Container Name"=""}], "Has Oneof"=FALSE}, {"Version"=2, "Name"="nixnet_grpc_EptRxFilter", "Type Url"="nixnet_grpc.EptRxFilter", "Elements"=[{"Field Name"="use_flags", "Embedded Message Name"="", "Protobuf Index"=1, "MessageElementType"=enum."UInt32Value", "Repeated"=FALSE, "Is in Oneof"=FALSE, "Oneof Container Name"=""}, {"Field Name"="vid", "Embedded Message Name"="", "Protobuf Index"=2, "MessageElementType"=enum."UInt32Value", "Repeated"=FALSE, "Is in Oneof"=FALSE, "Oneof Container Name"=""}, {"Field Name"="priority", "Embedded Message Name"="", "Protobuf Index"=3, "MessageElementType"=enum."UInt32Value", "Repeated"=FALSE, "Is in Oneof"=FALSE, "Oneof Container Name"=""}, {"Field Name"="destination_mac", "Embedded Message Name"="", "Protobuf Index"=4, "MessageElementType"=enum."StringValue", "Repeated"=FALSE, "Is in Oneof"=FALSE, "Oneof Container Name"=""}], "Has Oneof"=FALSE}, {"Version"=2, "Name"="nixnet_grpc_EptRxFilterArray", "Type Url"="nixnet_grpc.EptRxFilterArray", "Elements"=[{"Field Name"="ept_rx_filter", "Embedded Message Name"="nixnet_grpc_EptRxFilter", "Protobuf Index"=1, "MessageElementType"=enum."MessageValue", "Repeated"=TRUE, "Is in Oneof"=FALSE, "Oneof Container Name"=""}], "Has Oneof"=FALSE}, {"Version"=2, "Name"="nixnet_grpc_GetPropertyRequest", "Type Url"="nixnet_grpc.GetPropertyRequest", "Elements"=[{"Field Name"="selected_index", "Embedded Message Name"="", "Protobuf Index"=-1, "MessageElementType"=enum."Int32Value", "Repeated"=FALSE, "Is in Oneof"=TRUE, "Oneof Container Name"="nixnet_grpc_GetPropertyRequest_session_repository"}, {"Field Name"="device", "Embedded Message Name"="nidevice_grpc_Session", "Protobuf Index"=1, "MessageElementType"=enum."MessageValue", "Repeated"=FALSE, "Is in Oneof"=TRUE, "Oneof Container Name"="nixnet_grpc_GetPropertyRequest_session_repository"}, {"Field Name"="interface_ref", "Embedded Message Name"="nidevice_grpc_Session", "Protobuf Index"=2, "MessageElementType"=enum."MessageValue", "Repeated"=FALSE, "Is in Oneof"=TRUE, "Oneof Container Name"="nixnet_grpc_GetPropertyRequest_session_repository"}, {"Field Name"="session", "Embedded Message Name"="nidevice_grpc_Session", "Protobuf Index"=3, "MessageElementType"=enum."MessageValue", "Repeated"=FALSE, "Is in Oneof"=TRUE, "Oneof Container Name"="nixnet_grpc_GetPropertyRequest_session_repository"}, {"Field Name"="selected_index", "Embedded Message Name"="", "Protobuf Index"=-1, "MessageElementType"=enum."Int32Value", "Repeated"=FALSE, "Is in Oneof"=TRUE, "Oneof Container Name"="nixnet_grpc_GetPropertyRequest_property_id_enum"}, {"Field Name"="property_id", "Embedded Message Name"="nixnet_grpc_Property", "Protobuf Index"=4, "MessageElementType"=enum."EnumValue", "Repeated"=FALSE, "Is in Oneof"=TRUE, "Oneof Container Name"="nixnet_grpc_GetPropertyRequest_property_id_enum"}, {"Field Name"="property_id_raw", "Embedded Message Name"="", "Protobuf Index"=5, "MessageElementType"=enum."UInt32Value", "Repeated"=FALSE, "Is in Oneof"=TRUE, "Oneof Container Name"="nixnet_grpc_GetPropertyRequest_property_id_enum"}], "Has Oneof"=TRUE}, {"Version"=2, "Name"="nixnet_grpc_GetPropertyResponse", "Type Url"="nixnet_grpc.GetPropertyResponse", "Elements"=[{"Field Name"="status", "Embedded Message Name"="", "Protobuf Index"=1, "MessageElementType"=enum."Int32Value", "Repeated"=FALSE, "Is in Oneof"=FALSE, "Oneof Container Name"=""}, {"Field Name"="selected_index", "Embedded Message Name"="", "Protobuf Index"=-1, "MessageElementType"=enum."Int32Value", "Repeated"=FALSE, "Is in Oneof"=TRUE, "Oneof Container Name"="nixnet_grpc_GetPropertyResponse_property_value"}, {"Field Name"="u32_scalar", "Embedded Message Name"="", "Protobuf Index"=2, "MessageElementType"=enum."UInt32Value", "Repeated"=FALSE, "Is in Oneof"=TRUE, "Oneof Container Name"="nixnet_grpc_GetPropertyResponse_property_value"}, {"Field Name"="bool_scalar", "Embedded Message Name"="", "Protobuf Index"=3, "MessageElementType"=enum."BoolValue", "Repeated"=FALSE, "Is in Oneof"=TRUE, "Oneof Container Name"="nixnet_grpc_GetPropertyResponse_property_value"}, {"Field Name"="str", "Embedded Message Name"="", "Protobuf Index"=4, "MessageElementType"=enum."StringValue", "Repeated"=FALSE, "Is in Oneof"=TRUE, "Oneof Container Name"="nixnet_grpc_GetPropertyResponse_property_value"}, {"Field Name"="u64_scalar", "Embedded Message Name"="", "Protobuf Index"=5, "MessageElementType"=enum."UInt64Value", "Repeated"=FALSE, "Is in Oneof"=TRUE, "Oneof Container Name"="nixnet_grpc_GetPropertyResponse_property_value"}, {"Field Name"="i32_scalar", "Embedded Message Name"="", "Protobuf Index"=6, "MessageElementType"=enum."Int32Value", "Repeated"=FALSE, "Is in Oneof"=TRUE, "Oneof Container Name"="nixnet_grpc_GetPropertyResponse_property_value"}, {"Field Name"="f64_scalar", "Embedded Message Name"="", "Protobuf Index"=7, "MessageElementType"=enum."DoubleValue", "Repeated"=FALSE, "Is in Oneof"=TRUE, "Oneof Container Name"="nixnet_grpc_GetPropertyResponse_property_value"}, {"Field Name"="string_array", "Embedded Message Name"="", "Protobuf Index"=8, "MessageElementType"=enum."StringValue", "Repeated"=FALSE, "Is in Oneof"=TRUE, "Oneof Container Name"="nixnet_grpc_GetPropertyResponse_property_value"}, {"Field Name"="u32_array", "Embedded Message Name"="nixnet_grpc_U32Array", "Protobuf Index"=9, "MessageElementType"=enum."MessageValue", "Repeated"=FALSE, "Is in Oneof"=TRUE, "Oneof Container Name"="nixnet_grpc_GetPropertyResponse_property_value"}, {"Field Name"="db_ref", "Embedded Message Name"="nidevice_grpc_Session", "Protobuf Index"=10, "MessageElementType"=enum."MessageValue", "Repeated"=FALSE, "Is in Oneof"=TRUE, "Oneof Container Name"="nixnet_grpc_GetPropertyResponse_property_value"}, {"Field Name"="db_ref_array", "Embedded Message Name"="nixnet_grpc_DbRefArray", "Protobuf Index"=11, "MessageElementType"=enum."MessageValue", "Repeated"=FALSE, "Is in Oneof"=TRUE, "Oneof Container Name"="nixnet_grpc_GetPropertyResponse_property_value"}, {"Field Name"="dev_ref", "Embedded Message Name"="nidevice_grpc_Session", "Protobuf Index"=12, "MessageElementType"=enum."MessageValue", "Repeated"=FALSE, "Is in Oneof"=TRUE, "Oneof Container Name"="nixnet_grpc_GetPropertyResponse_property_value"}, {"Field Name"="dev_ref_array", "Embedded Message Name"="nixnet_grpc_DeviceRefArray", "Protobuf Index"=13, "MessageElementType"=enum."MessageValue", "Repeated"=FALSE, "Is in Oneof"=TRUE, "Oneof Container Name"="nixnet_grpc_GetPropertyResponse_property_value"}, {"Field Name"="intf_ref_array", "Embedded Message Name"="nixnet_grpc_InterfaceRefArray", "Protobuf Index"=14, "MessageElementType"=enum."MessageValue", "Repeated"=FALSE, "Is in Oneof"=TRUE, "Oneof Container Name"="nixnet_grpc_GetPropertyResponse_property_value"}, {"Field Name"="ept_rx_filter_array", "Embedded Message Name"="nixnet_grpc_EptRxFilterArray", "Protobuf Index"=15, "MessageElementType"=enum."MessageValue", "Repeated"=FALSE, "Is in Oneof"=TRUE, "Oneof Container Name"="nixnet_grpc_GetPropertyResponse_property_value"}], "Has Oneof"=TRUE}, {"Version"=2, "Name"="nixnet_grpc_SetPropertyRequest", "Type Url"="nixnet_grpc.SetPropertyRequest", "Elements"=[{"Field Name"="session", "Embedded Message Name"="nidevice_grpc_Session", "Protobuf Index"=1, "MessageElementType"=enum."MessageValue", "Repeated"=FALSE, "Is in Oneof"=FALSE, "Oneof Container Name"=""}, {"Field Name"="selected_index", "Embedded Message Name"="", "Protobuf Index"=-1, "MessageElementType"=enum."Int32Value", "Repeated"=FALSE, "Is in Oneof"=TRUE, "Oneof Container Name"="nixnet_grpc_SetPropertyRequest_property_id_enum"}, {"Field Name"="property_id", "Embedded Message Name"="nixnet_grpc_Property", "Protobuf Index"=2, "MessageElementType"=enum."EnumValue", "Repeated"=FALSE, "Is in Oneof"=TRUE, "Oneof Container Name"="nixnet_grpc_SetPropertyRequest_property_id_enum"}, {"Field Name"="property_id_raw", "Embedded Message Name"="", "Protobuf Index"=3, "MessageElementType"=enum."UInt32Value", "Repeated"=FALSE, "Is in Oneof"=TRUE, "Oneof Container Name"="nixnet_grpc_SetPropertyRequest_property_id_enum"}, {"Field Name"="selected_index", "Embedded Message Name"="", "Protobuf Index"=-1, "MessageElementType"=enum."Int32Value", "Repeated"=FALSE, "Is in Oneof"=TRUE, "Oneof Container Name"="nixnet_grpc_SetPropertyRequest_property_value"}, {"Field Name"="u32_scalar", "Embedded Message Name"="", "Protobuf Index"=4, "MessageElementType"=enum."UInt32Value", "Repeated"=FALSE, "Is in Oneof"=TRUE, "Oneof Container Name"="nixnet_grpc_SetPropertyRequest_property_value"}, {"Field Name"="bool_scalar", "Embedded Message Name"="", "Protobuf Index"=5, "MessageElementType"=enum."BoolValue", "Repeated"=FALSE, "Is in Oneof"=TRUE, "Oneof Container Name"="nixnet_grpc_SetPropertyRequest_property_value"}, {"Field Name"="str", "Embedded Message Name"="", "Protobuf Index"=6, "MessageElementType"=enum."StringValue", "Repeated"=FALSE, "Is in Oneof"=TRUE, "Oneof Container Name"="nixnet_grpc_SetPropertyRequest_property_value"}, {"Field Name"="u64_scalar", "Embedded Message Name"="", "Protobuf Index"=7, "MessageElementType"=enum."UInt64Value", "Repeated"=FALSE, "Is in Oneof"=TRUE, "Oneof Container Name"="nixnet_grpc_SetPropertyRequest_property_value"}, {"Field Name"="i32_scalar", "Embedded Message Name"="", "Protobuf Index"=8, "MessageElementType"=enum."Int32Value", "Repeated"=FALSE, "Is in Oneof"=TRUE, "Oneof Container Name"="nixnet_grpc_SetPropertyRequest_property_value"}, {"Field Name"="f64_scalar", "Embedded Message Name"="", "Protobuf Index"=9, "MessageElementType"=enum."DoubleValue", "Repeated"=FALSE, "Is in Oneof"=TRUE, "Oneof Container Name"="nixnet_grpc_SetPropertyRequest_property_value"}, {"Field Name"="string_array", "Embedded Message Name"="", "Protobuf Index"=10, "MessageElementType"=enum."StringValue", "Repeated"=FALSE, "Is in Oneof"=TRUE, "Oneof Container Name"="nixnet_grpc_SetPropertyRequest_property_value"}, {"Field Name"="u32_array", "Embedded Message Name"="nixnet_grpc_U32Array", "Protobuf Index"=11, "MessageElementType"=enum."MessageValue", "Repeated"=FALSE, "Is in Oneof"=TRUE, "Oneof Container Name"="nixnet_grpc_SetPropertyRequest_property_value"}, {"Field Name"="db_ref", "Embedded Message Name"="nidevice_grpc_Session", "Protobuf Index"=12, "MessageElementType"=enum."MessageValue", "Repeated"=FALSE, "Is in Oneof"=TRUE, "Oneof Container Name"="nixnet_grpc_SetPropertyRequest_property_value"}, {"Field Name"="db_ref_array", "Embedded Message Name"="nixnet_grpc_DbRefArray", "Protobuf Index"=13, "MessageElementType"=enum."MessageValue", "Repeated"=FALSE, "Is in Oneof"=TRUE, "Oneof Container Name"="nixnet_grpc_SetPropertyRequest_property_value"}, {"Field Name"="ept_rx_filter_array", "Embedded Message Name"="nixnet_grpc_EptRxFilterArray", "Protobuf Index"=14, "MessageElementType"=enum."MessageValue", "Repeated"=FALSE, "Is in Oneof"=TRUE, "Oneof Container Name"="nixnet_grpc_SetPropertyRequest_property_value"}], "Has Oneof"=TRUE}, {"Version"=2, "Name"="nixnet_grpc_SetPropertyResponse", "Type Url"="nixnet_grpc.SetPropertyResponse", "Elements"=[{"Field Name"="status", "Embedded Message Name"="", "Protobuf Index"=1, "MessageElementType"=enum."Int32Value", "Repeated"=FALSE, "Is in Oneof"=FALSE, "Oneof Container Name"=""}], "Has Oneof"=FALSE}, {"Version"=2, "Name"="nixnet_grpc_GetSubPropertyRequest", "Type Url"="nixnet_grpc.GetSubPropertyRequest", "Elements"=[{"Field Name"="session", "Embedded Message Name"="nidevice_grpc_Session", "Protobuf Index"=1, "MessageElementType"=enum."MessageValue", "Repeated"=FALSE, "Is in Oneof"=FALSE, "Oneof Container Name"=""}, {"Field Name"="active_index", "Embedded Message Name"="", "Protobuf Index"=2, "MessageElementType"=enum."UInt32Value", "Repeated"=FALSE, "Is in Oneof"=FALSE, "Oneof Container Name"=""}, {"Field Name"="selected_index", "Embedded Message Name"="", "Protobuf Index"=-1, "MessageElementType"=enum."Int32Value", "Repeated"=FALSE, "Is in Oneof"=TRUE, "Oneof Container Name"="nixnet_grpc_GetSubPropertyRequest_subproperty_id_enum"}, {"Field Name"="property_id", "Embedded Message Name"="nixnet_grpc_SubProperty", "Protobuf Index"=3, "MessageElementType"=enum."EnumValue", "Repeated"=FALSE, "Is in Oneof"=TRUE, "Oneof Container Name"="nixnet_grpc_GetSubPropertyRequest_subproperty_id_enum"}, {"Field Name"="property_id_raw", "Embedded Message Name"="", "Protobuf Index"=4, "MessageElementType"=enum."UInt32Value", "Repeated"=FALSE, "Is in Oneof"=TRUE, "Oneof Container Name"="nixnet_grpc_GetSubPropertyRequest_subproperty_id_enum"}], "Has Oneof"=TRUE}, {"Version"=2, "Name"="nixnet_grpc_GetSubPropertyResponse", "Type Url"="nixnet_grpc.GetSubPropertyResponse", "Elements"=[{"Field Name"="status", "Embedded Message Name"="", "Protobuf Index"=1, "MessageElementType"=enum."Int32Value", "Repeated"=FALSE, "Is in Oneof"=FALSE, "Oneof Container Name"=""}, {"Field Name"="selected_index", "Embedded Message Name"="", "Protobuf Index"=-1, "MessageElementType"=enum."Int32Value", "Repeated"=FALSE, "Is in Oneof"=TRUE, "Oneof Container Name"="nixnet_grpc_GetSubPropertyResponse_property_value"}, {"Field Name"="u32_scalar", "Embedded Message Name"="", "Protobuf Index"=2, "MessageElementType"=enum."UInt32Value", "Repeated"=FALSE, "Is in Oneof"=TRUE, "Oneof Container Name"="nixnet_grpc_GetSubPropertyResponse_property_value"}, {"Field Name"="str", "Embedded Message Name"="", "Protobuf Index"=3, "MessageElementType"=enum."StringValue", "Repeated"=FALSE, "Is in Oneof"=TRUE, "Oneof Container Name"="nixnet_grpc_GetSubPropertyResponse_property_value"}, {"Field Name"="f64_scalar", "Embedded Message Name"="", "Protobuf Index"=9, "MessageElementType"=enum."DoubleValue", "Repeated"=FALSE, "Is in Oneof"=TRUE, "Oneof Container Name"="nixnet_grpc_GetSubPropertyResponse_property_value"}], "Has Oneof"=TRUE}, {"Version"=2, "Name"="nixnet_grpc_DbGetPropertyRequest", "Type Url"="nixnet_grpc.DbGetPropertyRequest", "Elements"=[{"Field Name"="dbobject", "Embedded Message Name"="nidevice_grpc_Session", "Protobuf Index"=1, "MessageElementType"=enum."MessageValue", "Repeated"=FALSE, "Is in Oneof"=FALSE, "Oneof Container Name"=""}, {"Field Name"="selected_index", "Embedded Message Name"="", "Protobuf Index"=-1, "MessageElementType"=enum."Int32Value", "Repeated"=FALSE, "Is in Oneof"=TRUE, "Oneof Container Name"="nixnet_grpc_DbGetPropertyRequest_dbproperty_id_enum"}, {"Field Name"="property_id", "Embedded Message Name"="nixnet_grpc_DBProperty", "Protobuf Index"=2, "MessageElementType"=enum."EnumValue", "Repeated"=FALSE, "Is in Oneof"=TRUE, "Oneof Container Name"="nixnet_grpc_DbGetPropertyRequest_dbproperty_id_enum"}, {"Field Name"="property_id_raw", "Embedded Message Name"="", "Protobuf Index"=3, "MessageElementType"=enum."UInt32Value", "Repeated"=FALSE, "Is in Oneof"=TRUE, "Oneof Container Name"="nixnet_grpc_DbGetPropertyRequest_dbproperty_id_enum"}], "Has Oneof"=TRUE}, {"Version"=2, "Name"="nixnet_grpc_DbGetPropertyResponse", "Type Url"="nixnet_grpc.DbGetPropertyResponse", "Elements"=[{"Field Name"="status", "Embedded Message Name"="", "Protobuf Index"=1, "MessageElementType"=enum."Int32Value", "Repeated"=FALSE, "Is in Oneof"=FALSE, "Oneof Container Name"=""}, {"Field Name"="selected_index", "Embedded Message Name"="", "Protobuf Index"=-1, "MessageElementType"=enum."Int32Value", "Repeated"=FALSE, "Is in Oneof"=TRUE, "Oneof Container Name"="nixnet_grpc_DbGetPropertyResponse_property_value"}, {"Field Name"="u32_scalar", "Embedded Message Name"="", "Protobuf Index"=2, "MessageElementType"=enum."UInt32Value", "Repeated"=FALSE, "Is in Oneof"=TRUE, "Oneof Container Name"="nixnet_grpc_DbGetPropertyResponse_property_value"}, {"Field Name"="bool_scalar", "Embedded Message Name"="", "Protobuf Index"=3, "MessageElementType"=enum."BoolValue", "Repeated"=FALSE, "Is in Oneof"=TRUE, "Oneof Container Name"="nixnet_grpc_DbGetPropertyResponse_property_value"}, {"Field Name"="str", "Embedded Message Name"="", "Protobuf Index"=4, "MessageElementType"=enum."StringValue", "Repeated"=FALSE, "Is in Oneof"=TRUE, "Oneof Container Name"="nixnet_grpc_DbGetPropertyResponse_property_value"}, {"Field Name"="u64_scalar", "Embedded Message Name"="", "Protobuf Index"=5, "MessageElementType"=enum."UInt64Value", "Repeated"=FALSE, "Is in Oneof"=TRUE, "Oneof Container Name"="nixnet_grpc_DbGetPropertyResponse_property_value"}, {"Field Name"="f64_scalar", "Embedded Message Name"="", "Protobuf Index"=6, "MessageElementType"=enum."DoubleValue", "Repeated"=FALSE, "Is in Oneof"=TRUE, "Oneof Container Name"="nixnet_grpc_DbGetPropertyResponse_property_value"}, {"Field Name"="u32_array", "Embedded Message Name"="nixnet_grpc_U32Array", "Protobuf Index"=7, "MessageElementType"=enum."MessageValue", "Repeated"=FALSE, "Is in Oneof"=TRUE, "Oneof Container Name"="nixnet_grpc_DbGetPropertyResponse_property_value"}, {"Field Name"="u8_array", "Embedded Message Name"="", "Protobuf Index"=8, "MessageElementType"=enum."Bytes", "Repeated"=FALSE, "Is in Oneof"=TRUE, "Oneof Container Name"="nixnet_grpc_DbGetPropertyResponse_property_value"}, {"Field Name"="db_ref", "Embedded Message Name"="nidevice_grpc_Session", "Protobuf Index"=9, "MessageElementType"=enum."MessageValue", "Repeated"=FALSE, "Is in Oneof"=TRUE, "Oneof Container Name"="nixnet_grpc_DbGetPropertyResponse_property_value"}, {"Field Name"="db_ref_array", "Embedded Message Name"="nixnet_grpc_DbRefArray", "Protobuf Index"=10, "MessageElementType"=enum."MessageValue", "Repeated"=FALSE, "Is in Oneof"=TRUE, "Oneof Container Name"="nixnet_grpc_DbGetPropertyResponse_property_value"}], "Has Oneof"=TRUE}, {"Version"=2, "Name"="nixnet_grpc_SetSubPropertyRequest", "Type Url"="nixnet_grpc.SetSubPropertyRequest", "Elements"=[{"Field Name"="session", "Embedded Message Name"="nidevice_grpc_Session", "Protobuf Index"=1, "MessageElementType"=enum."MessageValue", "Repeated"=FALSE, "Is in Oneof"=FALSE, "Oneof Container Name"=""}, {"Field Name"="active_index", "Embedded Message Name"="", "Protobuf Index"=2, "MessageElementType"=enum."UInt32Value", "Repeated"=FALSE, "Is in Oneof"=FALSE, "Oneof Container Name"=""}, {"Field Name"="selected_index", "Embedded Message Name"="", "Protobuf Index"=-1, "MessageElementType"=enum."Int32Value", "Repeated"=FALSE, "Is in Oneof"=TRUE, "Oneof Container Name"="nixnet_grpc_SetSubPropertyRequest_subproperty_id_enum"}, {"Field Name"="property_id", "Embedded Message Name"="nixnet_grpc_SubProperty", "Protobuf Index"=3, "MessageElementType"=enum."EnumValue", "Repeated"=FALSE, "Is in Oneof"=TRUE, "Oneof Container Name"="nixnet_grpc_SetSubPropertyRequest_subproperty_id_enum"}, {"Field Name"="property_id_raw", "Embedded Message Name"="", "Protobuf Index"=4, "MessageElementType"=enum."UInt32Value", "Repeated"=FALSE, "Is in Oneof"=TRUE, "Oneof Container Name"="nixnet_grpc_SetSubPropertyRequest_subproperty_id_enum"}, {"Field Name"="selected_index", "Embedded Message Name"="", "Protobuf Index"=-1, "MessageElementType"=enum."Int32Value", "Repeated"=FALSE, "Is in Oneof"=TRUE, "Oneof Container Name"="nixnet_grpc_SetSubPropertyRequest_property_value"}, {"Field Name"="u32_scalar", "Embedded Message Name"="", "Protobuf Index"=5, "MessageElementType"=enum."UInt32Value", "Repeated"=FALSE, "Is in Oneof"=TRUE, "Oneof Container Name"="nixnet_grpc_SetSubPropertyRequest_property_value"}, {"Field Name"="str", "Embedded Message Name"="", "Protobuf Index"=6, "MessageElementType"=enum."StringValue", "Repeated"=FALSE, "Is in Oneof"=TRUE, "Oneof Container Name"="nixnet_grpc_SetSubPropertyRequest_property_value"}, {"Field Name"="f64_scalar", "Embedded Message Name"="", "Protobuf Index"=7, "MessageElementType"=enum."DoubleValue", "Repeated"=FALSE, "Is in Oneof"=TRUE, "Oneof Container Name"="nixnet_grpc_SetSubPropertyRequest_property_value"}], "Has Oneof"=TRUE}, {"Version"=2, "Name"="nixnet_grpc_SetSubPropertyResponse", "Type Url"="nixnet_grpc.SetSubPropertyResponse", "Elements"=[{"Field Name"="status", "Embedded Message Name"="", "Protobuf Index"=1, "MessageElementType"=enum."Int32Value", "Repeated"=FALSE, "Is in Oneof"=FALSE, "Oneof Container Name"=""}], "Has Oneof"=FALSE}, {"Version"=2, "Name"="nixnet_grpc_DbSetPropertyRequest", "Type Url"="nixnet_grpc.DbSetPropertyRequest", "Elements"=[{"Field Name"="dbobject", "Embedded Message Name"="nidevice_grpc_Session", "Protobuf Index"=1, "MessageElementType"=enum."MessageValue", "Repeated"=FALSE, "Is in Oneof"=FALSE, "Oneof Container Name"=""}, {"Field Name"="selected_index", "Embedded Message Name"="", "Protobuf Index"=-1, "MessageElementType"=enum."Int32Value", "Repeated"=FALSE, "Is in Oneof"=TRUE, "Oneof Container Name"="nixnet_grpc_DbSetPropertyRequest_dbproperty_id_enum"}, {"Field Name"="property_id", "Embedded Message Name"="nixnet_grpc_DBProperty", "Protobuf Index"=2, "MessageElementType"=enum."EnumValue", "Repeated"=FALSE, "Is in Oneof"=TRUE, "Oneof Container Name"="nixnet_grpc_DbSetPropertyRequest_dbproperty_id_enum"}, {"Field Name"="property_id_raw", "Embedded Message Name"="", "Protobuf Index"=3, "MessageElementType"=enum."UInt32Value", "Repeated"=FALSE, "Is in Oneof"=TRUE, "Oneof Container Name"="nixnet_grpc_DbSetPropertyRequest_dbproperty_id_enum"}, {"Field Name"="selected_index", "Embedded Message Name"="", "Protobuf Index"=-1, "MessageElementType"=enum."Int32Value", "Repeated"=FALSE, "Is in Oneof"=TRUE, "Oneof Container Name"="nixnet_grpc_DbSetPropertyRequest_property_value"}, {"Field Name"="u32_scalar", "Embedded Message Name"="", "Protobuf Index"=4, "MessageElementType"=enum."UInt32Value", "Repeated"=FALSE, "Is in Oneof"=TRUE, "Oneof Container Name"="nixnet_grpc_DbSetPropertyRequest_property_value"}, {"Field Name"="bool_scalar", "Embedded Message Name"="", "Protobuf Index"=5, "MessageElementType"=enum."BoolValue", "Repeated"=FALSE, "Is in Oneof"=TRUE, "Oneof Container Name"="nixnet_grpc_DbSetPropertyRequest_property_value"}, {"Field Name"="str", "Embedded Message Name"="", "Protobuf Index"=6, "MessageElementType"=enum."StringValue", "Repeated"=FALSE, "Is in Oneof"=TRUE, "Oneof Container Name"="nixnet_grpc_DbSetPropertyRequest_property_value"}, {"Field Name"="u64_scalar", "Embedded Message Name"="", "Protobuf Index"=7, "MessageElementType"=enum."UInt64Value", "Repeated"=FALSE, "Is in Oneof"=TRUE, "Oneof Container Name"="nixnet_grpc_DbSetPropertyRequest_property_value"}, {"Field Name"="f64_scalar", "Embedded Message Name"="", "Protobuf Index"=8, "MessageElementType"=enum."DoubleValue", "Repeated"=FALSE, "Is in Oneof"=TRUE, "Oneof Container Name"="nixnet_grpc_DbSetPropertyRequest_property_value"}, {"Field Name"="u32_array", "Embedded Message Name"="nixnet_grpc_U32Array", "Protobuf Index"=9, "MessageElementType"=enum."MessageValue", "Repeated"=FALSE, "Is in Oneof"=TRUE, "Oneof Container Name"="nixnet_grpc_DbSetPropertyRequest_property_value"}, {"Field Name"="u8_array", "Embedded Message Name"="", "Protobuf Index"=10, "MessageElementType"=enum."Bytes", "Repeated"=FALSE, "Is in Oneof"=TRUE, "Oneof Container Name"="nixnet_grpc_DbSetPropertyRequest_property_value"}, {"Field Name"="db_ref", "Embedded Message Name"="nidevice_grpc_Session", "Protobuf Index"=11, "MessageElementType"=enum."MessageValue", "Repeated"=FALSE, "Is in Oneof"=TRUE, "Oneof Container Name"="nixnet_grpc_DbSetPropertyRequest_property_value"}, {"Field Name"="db_ref_array", "Embedded Message Name"="nixnet_grpc_DbRefArray", "Protobuf Index"=12, "MessageElementType"=enum."MessageValue", "Repeated"=FALSE, "Is in Oneof"=TRUE, "Oneof Container Name"="nixnet_grpc_DbSetPropertyRequest_property_value"}], "Has Oneof"=TRUE}, {"Version"=2, "Name"="nixnet_grpc_DbSetPropertyResponse", "Type Url"="nixnet_grpc.DbSetPropertyResponse", "Elements"=[{"Field Name"="status", "Embedded Message Name"="", "Protobuf Index"=1, "MessageElementType"=enum."Int32Value", "Repeated"=FALSE, "Is in Oneof"=FALSE, "Oneof Container Name"=""}], "Has Oneof"=FALSE}, {"Version"=2, "Name"="nixnet_grpc_FrameRequest", "Type Url"="nixnet_grpc.FrameRequest", "Elements"=[{"Field Name"="timestamp", "Embedded Message Name"="", "Protobuf Index"=1, "MessageElementType"=enum."UInt64Value", "Repeated"=FALSE, "Is in Oneof"=FALSE, "Oneof Container Name"=""}, {"Field Name"="identifier", "Embedded Message Name"="", "Protobuf Index"=2, "MessageElementType"=enum."UInt32Value", "Repeated"=FALSE, "Is in Oneof"=FALSE, "Oneof Container Name"=""}, {"Field Name"="selected_index", "Embedded Message Name"="", "Protobuf Index"=-1, "MessageElementType"=enum."Int32Value", "Repeated"=FALSE, "Is in Oneof"=TRUE, "Oneof Container Name"="nixnet_grpc_FrameRequest_type_enum"}, {"Field Name"="type", "Embedded Message Name"="nixnet_grpc_FrameType", "Protobuf Index"=3, "MessageElementType"=enum."EnumValue", "Repeated"=FALSE, "Is in Oneof"=TRUE, "Oneof Container Name"="nixnet_grpc_FrameRequest_type_enum"}, {"Field Name"="type_raw", "Embedded Message Name"="", "Protobuf Index"=4, "MessageElementType"=enum."UInt32Value", "Repeated"=FALSE, "Is in Oneof"=TRUE, "Oneof Container Name"="nixnet_grpc_FrameRequest_type_enum"}, {"Field Name"="flags", "Embedded Message Name"="nixnet_grpc_FrameFlags", "Protobuf Index"=5, "MessageElementType"=enum."EnumValue", "Repeated"=TRUE, "Is in Oneof"=FALSE, "Oneof Container Name"=""}, {"Field Name"="info", "Embedded Message Name"="", "Protobuf Index"=6, "MessageElementType"=enum."UInt32Value", "Repeated"=FALSE, "Is in Oneof"=FALSE, "Oneof Container Name"=""}, {"Field Name"="payload", "Embedded Message Name"="", "Protobuf Index"=7, "MessageElementType"=enum."Bytes", "Repeated"=FALSE, "Is in Oneof"=FALSE, "Oneof Container Name"=""}], "Has Oneof"=TRUE}, {"Version"=2, "Name"="nixnet_grpc_FrameResponse", "Type Url"="nixnet_grpc.FrameResponse", "Elements"=[{"Field Name"="timestamp", "Embedded Message Name"="", "Protobuf Index"=1, "MessageElementType"=enum."UInt64Value", "Repeated"=FALSE, "Is in Oneof"=FALSE, "Oneof Container Name"=""}, {"Field Name"="identifier", "Embedded Message Name"="", "Protobuf Index"=2, "MessageElementType"=enum."UInt32Value", "Repeated"=FALSE, "Is in Oneof"=FALSE, "Oneof Container Name"=""}, {"Field Name"="type", "Embedded Message Name"="nixnet_grpc_FrameType", "Protobuf Index"=3, "MessageElementType"=enum."EnumValue", "Repeated"=FALSE, "Is in Oneof"=FALSE, "Oneof Container Name"=""}, {"Field Name"="type_raw", "Embedded Message Name"="", "Protobuf Index"=4, "MessageElementType"=enum."UInt32Value", "Repeated"=FALSE, "Is in Oneof"=FALSE, "Oneof Container Name"=""}, {"Field Name"="flags", "Embedded Message Name"="nixnet_grpc_FrameFlags", "Protobuf Index"=5, "MessageElementType"=enum."EnumValue", "Repeated"=TRUE, "Is in Oneof"=FALSE, "Oneof Container Name"=""}, {"Field Name"="flags_raw", "Embedded Message Name"="", "Protobuf Index"=6, "MessageElementType"=enum."UInt32Value", "Repeated"=FALSE, "Is in Oneof"=FALSE, "Oneof Container Name"=""}, {"Field Name"="info", "Embedded Message Name"="", "Protobuf Index"=7, "MessageElementType"=enum."UInt32Value", "Repeated"=FALSE, "Is in Oneof"=FALSE, "Oneof Container Name"=""}, {"Field Name"="payload", "Embedded Message Name"="", "Protobuf Index"=8, "MessageElementType"=enum."Bytes", "Repeated"=FALSE, "Is in Oneof"=FALSE, "Oneof Container Name"=""}], "Has Oneof"=FALSE}, {"Version"=2, "Name"="nixnet_grpc_EnetFrameRequest", "Type Url"="nixnet_grpc.EnetFrameRequest", "Elements"=[{"Field Name"="selected_index", "Embedded Message Name"="", "Protobuf Index"=-1, "MessageElementType"=enum."Int32Value", "Repeated"=FALSE, "Is in Oneof"=TRUE, "Oneof Container Name"="nixnet_grpc_EnetFrameRequest_type_enum"}, {"Field Name"="type", "Embedded Message Name"="nixnet_grpc_EnetFrameType", "Protobuf Index"=1, "MessageElementType"=enum."EnumValue", "Repeated"=FALSE, "Is in Oneof"=TRUE, "Oneof Container Name"="nixnet_grpc_EnetFrameRequest_type_enum"}, {"Field Name"="type_raw", "Embedded Message Name"="", "Protobuf Index"=2, "MessageElementType"=enum."UInt32Value", "Repeated"=FALSE, "Is in Oneof"=TRUE, "Oneof Container Name"="nixnet_grpc_EnetFrameRequest_type_enum"}, {"Field Name"="device_timestamp", "Embedded Message Name"="", "Protobuf Index"=3, "MessageElementType"=enum."UInt64Value", "Repeated"=FALSE, "Is in Oneof"=FALSE, "Oneof Container Name"=""}, {"Field Name"="network_timestamp", "Embedded Message Name"="", "Protobuf Index"=4, "MessageElementType"=enum."UInt64Value", "Repeated"=FALSE, "Is in Oneof"=FALSE, "Oneof Container Name"=""}, {"Field Name"="flags_mapped", "Embedded Message Name"="nixnet_grpc_EnetFlags", "Protobuf Index"=5, "MessageElementType"=enum."EnumValue", "Repeated"=TRUE, "Is in Oneof"=FALSE, "Oneof Container Name"=""}, {"Field Name"="frame_data", "Embedded Message Name"="", "Protobuf Index"=6, "MessageElementType"=enum."Bytes", "Repeated"=FALSE, "Is in Oneof"=FALSE, "Oneof Container Name"=""}], "Has Oneof"=TRUE}, {"Version"=2, "Name"="nixnet_grpc_EnetFrameResponse", "Type Url"="nixnet_grpc.EnetFrameResponse", "Elements"=[{"Field Name"="type", "Embedded Message Name"="nixnet_grpc_EnetFrameType", "Protobuf Index"=1, "MessageElementType"=enum."EnumValue", "Repeated"=FALSE, "Is in Oneof"=FALSE, "Oneof Container Name"=""}, {"Field Name"="type_raw", "Embedded Message Name"="", "Protobuf Index"=2, "MessageElementType"=enum."UInt32Value", "Repeated"=FALSE, "Is in Oneof"=FALSE, "Oneof Container Name"=""}, {"Field Name"="device_timestamp", "Embedded Message Name"="", "Protobuf Index"=3, "MessageElementType"=enum."UInt64Value", "Repeated"=FALSE, "Is in Oneof"=FALSE, "Oneof Container Name"=""}, {"Field Name"="network_timestamp", "Embedded Message Name"="", "Protobuf Index"=4, "MessageElementType"=enum."UInt64Value", "Repeated"=FALSE, "Is in Oneof"=FALSE, "Oneof Container Name"=""}, {"Field Name"="flags_mapped", "Embedded Message Name"="nixnet_grpc_EnetFlags", "Protobuf Index"=5, "MessageElementType"=enum."EnumValue", "Repeated"=TRUE, "Is in Oneof"=FALSE, "Oneof Container Name"=""}, {"Field Name"="flags_raw", "Embedded Message Name"="", "Protobuf Index"=6, "MessageElementType"=enum."UInt32Value", "Repeated"=FALSE, "Is in Oneof"=FALSE, "Oneof Container Name"=""}, {"Field Name"="frame_data", "Embedded Message Name"="", "Protobuf Index"=7, "MessageElementType"=enum."Bytes", "Repeated"=FALSE, "Is in Oneof"=FALSE, "Oneof Container Name"=""}], "Has Oneof"=FALSE}, {"Version"=2, "Name"="nixnet_grpc_FrameBufferRequest", "Type Url"="nixnet_grpc.FrameBufferRequest", "Elements"=[{"Field Name"="selected_index", "Embedded Message Name"="", "Protobuf Index"=-1, "MessageElementType"=enum."Int32Value", "Repeated"=FALSE, "Is in Oneof"=TRUE, "Oneof Container Name"="nixnet_grpc_FrameBufferRequest_frame"}, {"Field Name"="can", "Embedded Message Name"="nixnet_grpc_FrameRequest", "Protobuf Index"=1, "MessageElementType"=enum."MessageValue", "Repeated"=FALSE, "Is in Oneof"=TRUE, "Oneof Container Name"="nixnet_grpc_FrameBufferRequest_frame"}, {"Field Name"="lin", "Embedded Message Name"="nixnet_grpc_FrameRequest", "Protobuf Index"=2, "MessageElementType"=enum."MessageValue", "Repeated"=FALSE, "Is in Oneof"=TRUE, "Oneof Container Name"="nixnet_grpc_FrameBufferRequest_frame"}, {"Field Name"="flex_ray", "Embedded Message Name"="nixnet_grpc_FrameRequest", "Protobuf Index"=3, "MessageElementType"=enum."MessageValue", "Repeated"=FALSE, "Is in Oneof"=TRUE, "Oneof Container Name"="nixnet_grpc_FrameBufferRequest_frame"}, {"Field Name"="j1939", "Embedded Message Name"="nixnet_grpc_FrameRequest", "Protobuf Index"=4, "MessageElementType"=enum."MessageValue", "Repeated"=FALSE, "Is in Oneof"=TRUE, "Oneof Container Name"="nixnet_grpc_FrameBufferRequest_frame"}, {"Field Name"="enet", "Embedded Message Name"="nixnet_grpc_EnetFrameRequest", "Protobuf Index"=5, "MessageElementType"=enum."MessageValue", "Repeated"=FALSE, "Is in Oneof"=TRUE, "Oneof Container Name"="nixnet_grpc_FrameBufferRequest_frame"}], "Has Oneof"=TRUE}, {"Version"=2, "Name"="nixnet_grpc_FrameBufferResponse", "Type Url"="nixnet_grpc.FrameBufferResponse", "Elements"=[{"Field Name"="selected_index", "Embedded Message Name"="", "Protobuf Index"=-1, "MessageElementType"=enum."Int32Value", "Repeated"=FALSE, "Is in Oneof"=TRUE, "Oneof Container Name"="nixnet_grpc_FrameBufferResponse_frame"}, {"Field Name"="can", "Embedded Message Name"="nixnet_grpc_FrameResponse", "Protobuf Index"=1, "MessageElementType"=enum."MessageValue", "Repeated"=FALSE, "Is in Oneof"=TRUE, "Oneof Container Name"="nixnet_grpc_FrameBufferResponse_frame"}, {"Field Name"="lin", "Embedded Message Name"="nixnet_grpc_FrameResponse", "Protobuf Index"=2, "MessageElementType"=enum."MessageValue", "Repeated"=FALSE, "Is in Oneof"=TRUE, "Oneof Container Name"="nixnet_grpc_FrameBufferResponse_frame"}, {"Field Name"="flex_ray", "Embedded Message Name"="nixnet_grpc_FrameResponse", "Protobuf Index"=3, "MessageElementType"=enum."MessageValue", "Repeated"=FALSE, "Is in Oneof"=TRUE, "Oneof Container Name"="nixnet_grpc_FrameBufferResponse_frame"}, {"Field Name"="j1939", "Embedded Message Name"="nixnet_grpc_FrameResponse", "Protobuf Index"=4, "MessageElementType"=enum."MessageValue", "Repeated"=FALSE, "Is in Oneof"=TRUE, "Oneof Container Name"="nixnet_grpc_FrameBufferResponse_frame"}, {"Field Name"="enet", "Embedded Message Name"="nixnet_grpc_EnetFrameResponse", "Protobuf Index"=5, "MessageElementType"=enum."MessageValue", "Repeated"=FALSE, "Is in Oneof"=TRUE, "Oneof Container Name"="nixnet_grpc_FrameBufferResponse_frame"}], "Has Oneof"=TRUE}, {"Version"=2, "Name"="nixnet_grpc_TimeLocalNetwork", "Type Url"="nixnet_grpc.TimeLocalNetwork", "Elements"=[{"Field Name"="local_time", "Embedded Message Name"="", "Protobuf Index"=1, "MessageElementType"=enum."UInt64Value", "Repeated"=FALSE, "Is in Oneof"=FALSE, "Oneof Container Name"=""}, {"Field Name"="network_time", "Embedded Message Name"="", "Protobuf Index"=2, "MessageElementType"=enum."UInt64Value", "Repeated"=FALSE, "Is in Oneof"=FALSE, "Oneof Container Name"=""}, {"Field Name"="flags", "Embedded Message Name"="", "Protobuf Index"=3, "MessageElementType"=enum."UInt32Value", "Repeated"=FALSE, "Is in Oneof"=FALSE, "Oneof Container Name"=""}], "Has Oneof"=FALSE}, {"Version"=2, "Name"="nixnet_grpc_BlinkRequest", "Type Url"="nixnet_grpc.BlinkRequest", "Elements"=[{"Field Name"="interface_ref", "Embedded Message Name"="nidevice_grpc_Session", "Protobuf Index"=1, "MessageElementType"=enum."MessageValue", "Repeated"=FALSE, "Is in Oneof"=FALSE, "Oneof Container Name"=""}, {"Field Name"="selected_index", "Embedded Message Name"="", "Protobuf Index"=-1, "MessageElementType"=enum."Int32Value", "Repeated"=FALSE, "Is in Oneof"=TRUE, "Oneof Container Name"="nixnet_grpc_BlinkRequest_modifier_enum"}, {"Field Name"="modifier", "Embedded Message Name"="nixnet_grpc_BlinkMode", "Protobuf Index"=2, "MessageElementType"=enum."EnumValue", "Repeated"=FALSE, "Is in Oneof"=TRUE, "Oneof Container Name"="nixnet_grpc_BlinkRequest_modifier_enum"}, {"Field Name"="modifier_raw", "Embedded Message Name"="", "Protobuf Index"=3, "MessageElementType"=enum."UInt32Value", "Repeated"=FALSE, "Is in Oneof"=TRUE, "Oneof Container Name"="nixnet_grpc_BlinkRequest_modifier_enum"}], "Has Oneof"=TRUE}, {"Version"=2, "Name"="nixnet_grpc_BlinkResponse", "Type Url"="nixnet_grpc.BlinkResponse", "Elements"=[{"Field Name"="status", "Embedded Message Name"="", "Protobuf Index"=1, "MessageElementType"=enum."Int32Value", "Repeated"=FALSE, "Is in Oneof"=FALSE, "Oneof Container Name"=""}], "Has Oneof"=FALSE}, {"Version"=2, "Name"="nixnet_grpc_ClearRequest", "Type Url"="nixnet_grpc.ClearRequest", "Elements"=[{"Field Name"="session", "Embedded Message Name"="nidevice_grpc_Session", "Protobuf Index"=1, "MessageElementType"=enum."MessageValue", "Repeated"=FALSE, "Is in Oneof"=FALSE, "Oneof Container Name"=""}], "Has Oneof"=FALSE}, {"Version"=2, "Name"="nixnet_grpc_ClearResponse", "Type Url"="nixnet_grpc.ClearResponse", "Elements"=[{"Field Name"="status", "Embedded Message Name"="", "Protobuf Index"=1, "MessageElementType"=enum."Int32Value", "Repeated"=FALSE, "Is in Oneof"=FALSE, "Oneof Container Name"=""}], "Has Oneof"=FALSE}, {"Version"=2, "Name"="nixnet_grpc_ConnectTerminalsRequest", "Type Url"="nixnet_grpc.ConnectTerminalsRequest", "Elements"=[{"Field Name"="session", "Embedded Message Name"="nidevice_grpc_Session", "Protobuf Index"=1, "MessageElementType"=enum."MessageValue", "Repeated"=FALSE, "Is in Oneof"=FALSE, "Oneof Container Name"=""}, {"Field Name"="selected_index", "Embedded Message Name"="", "Protobuf Index"=-1, "MessageElementType"=enum."Int32Value", "Repeated"=FALSE, "Is in Oneof"=TRUE, "Oneof Container Name"="nixnet_grpc_ConnectTerminalsRequest_source_enum"}, {"Field Name"="source_mapped", "Embedded Message Name"="nixnet_grpc_TerminalName", "Protobuf Index"=2, "MessageElementType"=enum."EnumValue", "Repeated"=FALSE, "Is in Oneof"=TRUE, "Oneof Container Name"="nixnet_grpc_ConnectTerminalsRequest_source_enum"}, {"Field Name"="source_raw", "Embedded Message Name"="", "Protobuf Index"=3, "MessageElementType"=enum."StringValue", "Repeated"=FALSE, "Is in Oneof"=TRUE, "Oneof Container Name"="nixnet_grpc_ConnectTerminalsRequest_source_enum"}, {"Field Name"="selected_index", "Embedded Message Name"="", "Protobuf Index"=-1, "MessageElementType"=enum."Int32Value", "Repeated"=FALSE, "Is in Oneof"=TRUE, "Oneof Container Name"="nixnet_grpc_ConnectTerminalsRequest_destination_enum"}, {"Field Name"="destination_mapped", "Embedded Message Name"="nixnet_grpc_TerminalName", "Protobuf Index"=4, "MessageElementType"=enum."EnumValue", "Repeated"=FALSE, "Is in Oneof"=TRUE, "Oneof Container Name"="nixnet_grpc_ConnectTerminalsRequest_destination_enum"}, {"Field Name"="destination_raw", "Embedded Message Name"="", "Protobuf Index"=5, "MessageElementType"=enum."StringValue", "Repeated"=FALSE, "Is in Oneof"=TRUE, "Oneof Container Name"="nixnet_grpc_ConnectTerminalsRequest_destination_enum"}], "Has Oneof"=TRUE}, {"Version"=2, "Name"="nixnet_grpc_ConnectTerminalsResponse", "Type Url"="nixnet_grpc.ConnectTerminalsResponse", "Elements"=[{"Field Name"="status", "Embedded Message Name"="", "Protobuf Index"=1, "MessageElementType"=enum."Int32Value", "Repeated"=FALSE, "Is in Oneof"=FALSE, "Oneof Container Name"=""}], "Has Oneof"=FALSE}, {"Version"=2, "Name"="nixnet_grpc_ConvertByteArrayToFramesSinglePointRequest", "Type Url"="nixnet_grpc.ConvertByteArrayToFramesSinglePointRequest", "Elements"=[{"Field Name"="session", "Embedded Message Name"="nidevice_grpc_Session", "Protobuf Index"=1, "MessageElementType"=enum."MessageValue", "Repeated"=FALSE, "Is in Oneof"=FALSE, "Oneof Container Name"=""}, {"Field Name"="value_buffer", "Embedded Message Name"="", "Protobuf Index"=2, "MessageElementType"=enum."Bytes", "Repeated"=FALSE, "Is in Oneof"=FALSE, "Oneof Container Name"=""}, {"Field Name"="number_of_frames", "Embedded Message Name"="", "Protobuf Index"=3, "MessageElementType"=enum."UInt32Value", "Repeated"=FALSE, "Is in Oneof"=FALSE, "Oneof Container Name"=""}, {"Field Name"="max_payload_per_frame", "Embedded Message Name"="", "Protobuf Index"=4, "MessageElementType"=enum."UInt32Value", "Repeated"=FALSE, "Is in Oneof"=FALSE, "Oneof Container Name"=""}, {"Field Name"="selected_index", "Embedded Message Name"="", "Protobuf Index"=-1, "MessageElementType"=enum."Int32Value", "Repeated"=FALSE, "Is in Oneof"=TRUE, "Oneof Container Name"="nixnet_grpc_ConvertByteArrayToFramesSinglePointRequest_protocol_enum"}, {"Field Name"="protocol", "Embedded Message Name"="nixnet_grpc_Protocol", "Protobuf Index"=5, "MessageElementType"=enum."EnumValue", "Repeated"=FALSE, "Is in Oneof"=TRUE, "Oneof Container Name"="nixnet_grpc_ConvertByteArrayToFramesSinglePointRequest_protocol_enum"}, {"Field Name"="protocol_raw", "Embedded Message Name"="", "Protobuf Index"=6, "MessageElementType"=enum."UInt32Value", "Repeated"=FALSE, "Is in Oneof"=TRUE, "Oneof Container Name"="nixnet_grpc_ConvertByteArrayToFramesSinglePointRequest_protocol_enum"}], "Has Oneof"=TRUE}, {"Version"=2, "Name"="nixnet_grpc_ConvertByteArrayToFramesSinglePointResponse", "Type Url"="nixnet_grpc.ConvertByteArrayToFramesSinglePointResponse", "Elements"=[{"Field Name"="status", "Embedded Message Name"="", "Protobuf Index"=1, "MessageElementType"=enum."Int32Value", "Repeated"=FALSE, "Is in Oneof"=FALSE, "Oneof Container Name"=""}, {"Field Name"="buffer", "Embedded Message Name"="nixnet_grpc_FrameBufferResponse", "Protobuf Index"=2, "MessageElementType"=enum."MessageValue", "Repeated"=TRUE, "Is in Oneof"=FALSE, "Oneof Container Name"=""}], "Has Oneof"=FALSE}, {"Version"=2, "Name"="nixnet_grpc_ConvertFramesToByteArraySinglePointRequest", "Type Url"="nixnet_grpc.ConvertFramesToByteArraySinglePointRequest", "Elements"=[{"Field Name"="session", "Embedded Message Name"="nidevice_grpc_Session", "Protobuf Index"=1, "MessageElementType"=enum."MessageValue", "Repeated"=FALSE, "Is in Oneof"=FALSE, "Oneof Container Name"=""}, {"Field Name"="frame_buffer", "Embedded Message Name"="nixnet_grpc_FrameBufferRequest", "Protobuf Index"=2, "MessageElementType"=enum."MessageValue", "Repeated"=TRUE, "Is in Oneof"=FALSE, "Oneof Container Name"=""}, {"Field Name"="size_of_value_buffer", "Embedded Message Name"="", "Protobuf Index"=3, "MessageElementType"=enum."UInt32Value", "Repeated"=FALSE, "Is in Oneof"=FALSE, "Oneof Container Name"=""}], "Has Oneof"=FALSE}, {"Version"=2, "Name"="nixnet_grpc_ConvertFramesToByteArraySinglePointResponse", "Type Url"="nixnet_grpc.ConvertFramesToByteArraySinglePointResponse", "Elements"=[{"Field Name"="status", "Embedded Message Name"="", "Protobuf Index"=1, "MessageElementType"=enum."Int32Value", "Repeated"=FALSE, "Is in Oneof"=FALSE, "Oneof Container Name"=""}, {"Field Name"="value_buffer", "Embedded Message Name"="", "Protobuf Index"=2, "MessageElementType"=enum."Bytes", "Repeated"=FALSE, "Is in Oneof"=FALSE, "Oneof Container Name"=""}], "Has Oneof"=FALSE}, {"Version"=2, "Name"="nixnet_grpc_ConvertFramesToSignalsSinglePointRequest", "Type Url"="nixnet_grpc.ConvertFramesToSignalsSinglePointRequest", "Elements"=[{"Field Name"="session", "Embedded Message Name"="nidevice_grpc_Session", "Protobuf Index"=1, "MessageElementType"=enum."MessageValue", "Repeated"=FALSE, "Is in Oneof"=FALSE, "Oneof Container Name"=""}, {"Field Name"="number_of_signals", "Embedded Message Name"="", "Protobuf Index"=2, "MessageElementType"=enum."UInt32Value", "Repeated"=FALSE, "Is in Oneof"=FALSE, "Oneof Container Name"=""}, {"Field Name"="frame_buffer", "Embedded Message Name"="nixnet_grpc_FrameBufferRequest", "Protobuf Index"=3, "MessageElementType"=enum."MessageValue", "Repeated"=TRUE, "Is in Oneof"=FALSE, "Oneof Container Name"=""}], "Has Oneof"=FALSE}, {"Version"=2, "Name"="nixnet_grpc_ConvertFramesToSignalsSinglePointResponse", "Type Url"="nixnet_grpc.ConvertFramesToSignalsSinglePointResponse", "Elements"=[{"Field Name"="status", "Embedded Message Name"="", "Protobuf Index"=1, "MessageElementType"=enum."Int32Value", "Repeated"=FALSE, "Is in Oneof"=FALSE, "Oneof Container Name"=""}, {"Field Name"="value_buffer", "Embedded Message Name"="", "Protobuf Index"=2, "MessageElementType"=enum."DoubleValue", "Repeated"=TRUE, "Is in Oneof"=FALSE, "Oneof Container Name"=""}, {"Field Name"="timestamp_buffer", "Embedded Message Name"="", "Protobuf Index"=3, "MessageElementType"=enum."UInt64Value", "Repeated"=TRUE, "Is in Oneof"=FALSE, "Oneof Container Name"=""}], "Has Oneof"=FALSE}, {"Version"=2, "Name"="nixnet_grpc_ConvertSignalsToFramesSinglePointRequest", "Type Url"="nixnet_grpc.ConvertSignalsToFramesSinglePointRequest", "Elements"=[{"Field Name"="session", "Embedded Message Name"="nidevice_grpc_Session", "Protobuf Index"=1, "MessageElementType"=enum."MessageValue", "Repeated"=FALSE, "Is in Oneof"=FALSE, "Oneof Container Name"=""}, {"Field Name"="value_buffer", "Embedded Message Name"="", "Protobuf Index"=2, "MessageElementType"=enum."DoubleValue", "Repeated"=TRUE, "Is in Oneof"=FALSE, "Oneof Container Name"=""}, {"Field Name"="number_of_frames", "Embedded Message Name"="", "Protobuf Index"=3, "MessageElementType"=enum."UInt32Value", "Repeated"=FALSE, "Is in Oneof"=FALSE, "Oneof Container Name"=""}, {"Field Name"="max_payload_per_frame", "Embedded Message Name"="", "Protobuf Index"=4, "MessageElementType"=enum."UInt32Value", "Repeated"=FALSE, "Is in Oneof"=FALSE, "Oneof Container Name"=""}, {"Field Name"="selected_index", "Embedded Message Name"="", "Protobuf Index"=-1, "MessageElementType"=enum."Int32Value", "Repeated"=FALSE, "Is in Oneof"=TRUE, "Oneof Container Name"="nixnet_grpc_ConvertSignalsToFramesSinglePointRequest_protocol_enum"}, {"Field Name"="protocol", "Embedded Message Name"="nixnet_grpc_Protocol", "Protobuf Index"=5, "MessageElementType"=enum."EnumValue", "Repeated"=FALSE, "Is in Oneof"=TRUE, "Oneof Container Name"="nixnet_grpc_ConvertSignalsToFramesSinglePointRequest_protocol_enum"}, {"Field Name"="protocol_raw", "Embedded Message Name"="", "Protobuf Index"=6, "MessageElementType"=enum."UInt32Value", "Repeated"=FALSE, "Is in Oneof"=TRUE, "Oneof Container Name"="nixnet_grpc_ConvertSignalsToFramesSinglePointRequest_protocol_enum"}], "Has Oneof"=TRUE}, {"Version"=2, "Name"="nixnet_grpc_ConvertSignalsToFramesSinglePointResponse", "Type Url"="nixnet_grpc.ConvertSignalsToFramesSinglePointResponse", "Elements"=[{"Field Name"="status", "Embedded Message Name"="", "Protobuf Index"=1, "MessageElementType"=enum."Int32Value", "Repeated"=FALSE, "Is in Oneof"=FALSE, "Oneof Container Name"=""}, {"Field Name"="buffer", "Embedded Message Name"="nixnet_grpc_FrameBufferResponse", "Protobuf Index"=2, "MessageElementType"=enum."MessageValue", "Repeated"=TRUE, "Is in Oneof"=FALSE, "Oneof Container Name"=""}], "Has Oneof"=FALSE}, {"Version"=2, "Name"="nixnet_grpc_ConvertTimestamp100nsTo1nsRequest", "Type Url"="nixnet_grpc.ConvertTimestamp100nsTo1nsRequest", "Elements"=[{"Field Name"="from_timestamp_100ns", "Embedded Message Name"="", "Protobuf Index"=1, "MessageElementType"=enum."UInt64Value", "Repeated"=FALSE, "Is in Oneof"=FALSE, "Oneof Container Name"=""}], "Has Oneof"=FALSE}, {"Version"=2, "Name"="nixnet_grpc_ConvertTimestamp100nsTo1nsResponse", "Type Url"="nixnet_grpc.ConvertTimestamp100nsTo1nsResponse", "Elements"=[{"Field Name"="status", "Embedded Message Name"="", "Protobuf Index"=1, "MessageElementType"=enum."Int32Value", "Repeated"=FALSE, "Is in Oneof"=FALSE, "Oneof Container Name"=""}, {"Field Name"="to_timestamp_1ns", "Embedded Message Name"="", "Protobuf Index"=2, "MessageElementType"=enum."UInt64Value", "Repeated"=FALSE, "Is in Oneof"=FALSE, "Oneof Container Name"=""}], "Has Oneof"=FALSE}, {"Version"=2, "Name"="nixnet_grpc_ConvertTimestamp1nsTo100nsRequest", "Type Url"="nixnet_grpc.ConvertTimestamp1nsTo100nsRequest", "Elements"=[{"Field Name"="from_timestamp_1ns", "Embedded Message Name"="", "Protobuf Index"=1, "MessageElementType"=enum."UInt64Value", "Repeated"=FALSE, "Is in Oneof"=FALSE, "Oneof Container Name"=""}], "Has Oneof"=FALSE}, {"Version"=2, "Name"="nixnet_grpc_ConvertTimestamp1nsTo100nsResponse", "Type Url"="nixnet_grpc.ConvertTimestamp1nsTo100nsResponse", "Elements"=[{"Field Name"="status", "Embedded Message Name"="", "Protobuf Index"=1, "MessageElementType"=enum."Int32Value", "Repeated"=FALSE, "Is in Oneof"=FALSE, "Oneof Container Name"=""}, {"Field Name"="to_timestamp_100ns", "Embedded Message Name"="", "Protobuf Index"=2, "MessageElementType"=enum."UInt64Value", "Repeated"=FALSE, "Is in Oneof"=FALSE, "Oneof Container Name"=""}], "Has Oneof"=FALSE}, {"Version"=2, "Name"="nixnet_grpc_CreateSessionRequest", "Type Url"="nixnet_grpc.CreateSessionRequest", "Elements"=[{"Field Name"="session_name", "Embedded Message Name"="", "Protobuf Index"=1, "MessageElementType"=enum."StringValue", "Repeated"=FALSE, "Is in Oneof"=FALSE, "Oneof Container Name"=""}, {"Field Name"="database_name", "Embedded Message Name"="", "Protobuf Index"=2, "MessageElementType"=enum."StringValue", "Repeated"=FALSE, "Is in Oneof"=FALSE, "Oneof Container Name"=""}, {"Field Name"="cluster_name", "Embedded Message Name"="", "Protobuf Index"=3, "MessageElementType"=enum."StringValue", "Repeated"=FALSE, "Is in Oneof"=FALSE, "Oneof Container Name"=""}, {"Field Name"="list", "Embedded Message Name"="", "Protobuf Index"=4, "MessageElementType"=enum."StringValue", "Repeated"=FALSE, "Is in Oneof"=FALSE, "Oneof Container Name"=""}, {"Field Name"="interface_name", "Embedded Message Name"="", "Protobuf Index"=5, "MessageElementType"=enum."StringValue", "Repeated"=FALSE, "Is in Oneof"=FALSE, "Oneof Container Name"=""}, {"Field Name"="selected_index", "Embedded Message Name"="", "Protobuf Index"=-1, "MessageElementType"=enum."Int32Value", "Repeated"=FALSE, "Is in Oneof"=TRUE, "Oneof Container Name"="nixnet_grpc_CreateSessionRequest_mode_enum"}, {"Field Name"="mode", "Embedded Message Name"="nixnet_grpc_CreateSessionMode", "Protobuf Index"=6, "MessageElementType"=enum."EnumValue", "Repeated"=FALSE, "Is in Oneof"=TRUE, "Oneof Container Name"="nixnet_grpc_CreateSessionRequest_mode_enum"}, {"Field Name"="mode_raw", "Embedded Message Name"="", "Protobuf Index"=7, "MessageElementType"=enum."UInt32Value", "Repeated"=FALSE, "Is in Oneof"=TRUE, "Oneof Container Name"="nixnet_grpc_CreateSessionRequest_mode_enum"}, {"Field Name"="initialization_behavior", "Embedded Message Name"="nidevice_grpc_SessionInitializationBehavior", "Protobuf Index"=8, "MessageElementType"=enum."EnumValue", "Repeated"=FALSE, "Is in Oneof"=FALSE, "Oneof Container Name"=""}], "Has Oneof"=TRUE}, {"Version"=2, "Name"="nixnet_grpc_CreateSessionResponse", "Type Url"="nixnet_grpc.CreateSessionResponse", "Elements"=[{"Field Name"="status", "Embedded Message Name"="", "Protobuf Index"=1, "MessageElementType"=enum."Int32Value", "Repeated"=FALSE, "Is in Oneof"=FALSE, "Oneof Container Name"=""}, {"Field Name"="session", "Embedded Message Name"="nidevice_grpc_Session", "Protobuf Index"=2, "MessageElementType"=enum."MessageValue", "Repeated"=FALSE, "Is in Oneof"=FALSE, "Oneof Container Name"=""}, {"Field Name"="new_session_initialized", "Embedded Message Name"="", "Protobuf Index"=3, "MessageElementType"=enum."BoolValue", "Repeated"=FALSE, "Is in Oneof"=FALSE, "Oneof Container Name"=""}], "Has Oneof"=FALSE}, {"Version"=2, "Name"="nixnet_grpc_CreateSessionByRefRequest", "Type Url"="nixnet_grpc.CreateSessionByRefRequest", "Elements"=[{"Field Name"="session_name", "Embedded Message Name"="", "Protobuf Index"=1, "MessageElementType"=enum."StringValue", "Repeated"=FALSE, "Is in Oneof"=FALSE, "Oneof Container Name"=""}, {"Field Name"="array_of_database_ref", "Embedded Message Name"="nidevice_grpc_Session", "Protobuf Index"=2, "MessageElementType"=enum."MessageValue", "Repeated"=TRUE, "Is in Oneof"=FALSE, "Oneof Container Name"=""}, {"Field Name"="interface_name", "Embedded Message Name"="", "Protobuf Index"=3, "MessageElementType"=enum."StringValue", "Repeated"=FALSE, "Is in Oneof"=FALSE, "Oneof Container Name"=""}, {"Field Name"="selected_index", "Embedded Message Name"="", "Protobuf Index"=-1, "MessageElementType"=enum."Int32Value", "Repeated"=FALSE, "Is in Oneof"=TRUE, "Oneof Container Name"="nixnet_grpc_CreateSessionByRefRequest_mode_enum"}, {"Field Name"="mode", "Embedded Message Name"="nixnet_grpc_CreateSessionMode", "Protobuf Index"=4, "MessageElementType"=enum."EnumValue", "Repeated"=FALSE, "Is in Oneof"=TRUE, "Oneof Container Name"="nixnet_grpc_CreateSessionByRefRequest_mode_enum"}, {"Field Name"="mode_raw", "Embedded Message Name"="", "Protobuf Index"=5, "MessageElementType"=enum."UInt32Value", "Repeated"=FALSE, "Is in Oneof"=TRUE, "Oneof Container Name"="nixnet_grpc_CreateSessionByRefRequest_mode_enum"}, {"Field Name"="initialization_behavior", "Embedded Message Name"="nidevice_grpc_SessionInitializationBehavior", "Protobuf Index"=6, "MessageElementType"=enum."EnumValue", "Repeated"=FALSE, "Is in Oneof"=FALSE, "Oneof Container Name"=""}], "Has Oneof"=TRUE}, {"Version"=2, "Name"="nixnet_grpc_CreateSessionByRefResponse", "Type Url"="nixnet_grpc.CreateSessionByRefResponse", "Elements"=[{"Field Name"="status", "Embedded Message Name"="", "Protobuf Index"=1, "MessageElementType"=enum."Int32Value", "Repeated"=FALSE, "Is in Oneof"=FALSE, "Oneof Container Name"=""}, {"Field Name"="session", "Embedded Message Name"="nidevice_grpc_Session", "Protobuf Index"=2, "MessageElementType"=enum."MessageValue", "Repeated"=FALSE, "Is in Oneof"=FALSE, "Oneof Container Name"=""}, {"Field Name"="new_session_initialized", "Embedded Message Name"="", "Protobuf Index"=3, "MessageElementType"=enum."BoolValue", "Repeated"=FALSE, "Is in Oneof"=FALSE, "Oneof Container Name"=""}], "Has Oneof"=FALSE}, {"Version"=2, "Name"="nixnet_grpc_DbAddAliasRequest", "Type Url"="nixnet_grpc.DbAddAliasRequest", "Elements"=[{"Field Name"="database_alias", "Embedded Message Name"="", "Protobuf Index"=1, "MessageElementType"=enum."StringValue", "Repeated"=FALSE, "Is in Oneof"=FALSE, "Oneof Container Name"=""}, {"Field Name"="database_filepath", "Embedded Message Name"="", "Protobuf Index"=2, "MessageElementType"=enum."StringValue", "Repeated"=FALSE, "Is in Oneof"=FALSE, "Oneof Container Name"=""}, {"Field Name"="default_baud_rate", "Embedded Message Name"="", "Protobuf Index"=3, "MessageElementType"=enum."UInt32Value", "Repeated"=FALSE, "Is in Oneof"=FALSE, "Oneof Container Name"=""}], "Has Oneof"=FALSE}, {"Version"=2, "Name"="nixnet_grpc_DbAddAliasResponse", "Type Url"="nixnet_grpc.DbAddAliasResponse", "Elements"=[{"Field Name"="status", "Embedded Message Name"="", "Protobuf Index"=1, "MessageElementType"=enum."Int32Value", "Repeated"=FALSE, "Is in Oneof"=FALSE, "Oneof Container Name"=""}], "Has Oneof"=FALSE}, {"Version"=2, "Name"="nixnet_grpc_DbAddAlias64Request", "Type Url"="nixnet_grpc.DbAddAlias64Request", "Elements"=[{"Field Name"="database_alias", "Embedded Message Name"="", "Protobuf Index"=1, "MessageElementType"=enum."StringValue", "Repeated"=FALSE, "Is in Oneof"=FALSE, "Oneof Container Name"=""}, {"Field Name"="database_filepath", "Embedded Message Name"="", "Protobuf Index"=2, "MessageElementType"=enum."StringValue", "Repeated"=FALSE, "Is in Oneof"=FALSE, "Oneof Container Name"=""}, {"Field Name"="default_baud_rate", "Embedded Message Name"="", "Protobuf Index"=3, "MessageElementType"=enum."UInt64Value", "Repeated"=FALSE, "Is in Oneof"=FALSE, "Oneof Container Name"=""}], "Has Oneof"=FALSE}, {"Version"=2, "Name"="nixnet_grpc_DbAddAlias64Response", "Type Url"="nixnet_grpc.DbAddAlias64Response", "Elements"=[{"Field Name"="status", "Embedded Message Name"="", "Protobuf Index"=1, "MessageElementType"=enum."Int32Value", "Repeated"=FALSE, "Is in Oneof"=FALSE, "Oneof Container Name"=""}], "Has Oneof"=FALSE}, {"Version"=2, "Name"="nixnet_grpc_DbCloseDatabaseRequest", "Type Url"="nixnet_grpc.DbCloseDatabaseRequest", "Elements"=[{"Field Name"="database", "Embedded Message Name"="nidevice_grpc_Session", "Protobuf Index"=1, "MessageElementType"=enum."MessageValue", "Repeated"=FALSE, "Is in Oneof"=FALSE, "Oneof Container Name"=""}, {"Field Name"="close_all_refs", "Embedded Message Name"="", "Protobuf Index"=2, "MessageElementType"=enum."UInt32Value", "Repeated"=FALSE, "Is in Oneof"=FALSE, "Oneof Container Name"=""}], "Has Oneof"=FALSE}, {"Version"=2, "Name"="nixnet_grpc_DbCloseDatabaseResponse", "Type Url"="nixnet_grpc.DbCloseDatabaseResponse", "Elements"=[{"Field Name"="status", "Embedded Message Name"="", "Protobuf Index"=1, "MessageElementType"=enum."Int32Value", "Repeated"=FALSE, "Is in Oneof"=FALSE, "Oneof Container Name"=""}], "Has Oneof"=FALSE}, {"Version"=2, "Name"="nixnet_grpc_DbCreateObjectRequest", "Type Url"="nixnet_grpc.DbCreateObjectRequest", "Elements"=[{"Field Name"="session_name", "Embedded Message Name"="", "Protobuf Index"=1, "MessageElementType"=enum."StringValue", "Repeated"=FALSE, "Is in Oneof"=FALSE, "Oneof Container Name"=""}, {"Field Name"="parent_object", "Embedded Message Name"="nidevice_grpc_Session", "Protobuf Index"=2, "MessageElementType"=enum."MessageValue", "Repeated"=FALSE, "Is in Oneof"=FALSE, "Oneof Container Name"=""}, {"Field Name"="object_class", "Embedded Message Name"="", "Protobuf Index"=3, "MessageElementType"=enum."UInt32Value", "Repeated"=FALSE, "Is in Oneof"=FALSE, "Oneof Container Name"=""}, {"Field Name"="object_name", "Embedded Message Name"="", "Protobuf Index"=4, "MessageElementType"=enum."StringValue", "Repeated"=FALSE, "Is in Oneof"=FALSE, "Oneof Container Name"=""}], "Has Oneof"=FALSE}, {"Version"=2, "Name"="nixnet_grpc_DbCreateObjectResponse", "Type Url"="nixnet_grpc.DbCreateObjectResponse", "Elements"=[{"Field Name"="status", "Embedded Message Name"="", "Protobuf Index"=1, "MessageElementType"=enum."Int32Value", "Repeated"=FALSE, "Is in Oneof"=FALSE, "Oneof Container Name"=""}, {"Field Name"="db_object", "Embedded Message Name"="nidevice_grpc_Session", "Protobuf Index"=2, "MessageElementType"=enum."MessageValue", "Repeated"=FALSE, "Is in Oneof"=FALSE, "Oneof Container Name"=""}], "Has Oneof"=FALSE}, {"Version"=2, "Name"="nixnet_grpc_DbDeleteObjectRequest", "Type Url"="nixnet_grpc.DbDeleteObjectRequest", "Elements"=[{"Field Name"="db_object", "Embedded Message Name"="nidevice_grpc_Session", "Protobuf Index"=1, "MessageElementType"=enum."MessageValue", "Repeated"=FALSE, "Is in Oneof"=FALSE, "Oneof Container Name"=""}], "Has Oneof"=FALSE}, {"Version"=2, "Name"="nixnet_grpc_DbDeleteObjectResponse", "Type Url"="nixnet_grpc.DbDeleteObjectResponse", "Elements"=[{"Field Name"="status", "Embedded Message Name"="", "Protobuf Index"=1, "MessageElementType"=enum."Int32Value", "Repeated"=FALSE, "Is in Oneof"=FALSE, "Oneof Container Name"=""}], "Has Oneof"=FALSE}, {"Version"=2, "Name"="nixnet_grpc_DbDeployRequest", "Type Url"="nixnet_grpc.DbDeployRequest", "Elements"=[{"Field Name"="ip_address", "Embedded Message Name"="", "Protobuf Index"=1, "MessageElementType"=enum."StringValue", "Repeated"=FALSE, "Is in Oneof"=FALSE, "Oneof Container Name"=""}, {"Field Name"="database_alias", "Embedded Message Name"="", "Protobuf Index"=2, "MessageElementType"=enum."StringValue", "Repeated"=FALSE, "Is in Oneof"=FALSE, "Oneof Container Name"=""}, {"Field Name"="wait_for_complete", "Embedded Message Name"="", "Protobuf Index"=3, "MessageElementType"=enum."UInt32Value", "Repeated"=FALSE, "Is in Oneof"=FALSE, "Oneof Container Name"=""}], "Has Oneof"=FALSE}, {"Version"=2, "Name"="nixnet_grpc_DbDeployResponse", "Type Url"="nixnet_grpc.DbDeployResponse", "Elements"=[{"Field Name"="status", "Embedded Message Name"="", "Protobuf Index"=1, "MessageElementType"=enum."Int32Value", "Repeated"=FALSE, "Is in Oneof"=FALSE, "Oneof Container Name"=""}, {"Field Name"="percent_complete", "Embedded Message Name"="", "Protobuf Index"=2, "MessageElementType"=enum."UInt32Value", "Repeated"=FALSE, "Is in Oneof"=FALSE, "Oneof Container Name"=""}], "Has Oneof"=FALSE}, {"Version"=2, "Name"="nixnet_grpc_DbFindObjectRequest", "Type Url"="nixnet_grpc.DbFindObjectRequest", "Elements"=[{"Field Name"="session_name", "Embedded Message Name"="", "Protobuf Index"=1, "MessageElementType"=enum."StringValue", "Repeated"=FALSE, "Is in Oneof"=FALSE, "Oneof Container Name"=""}, {"Field Name"="parent_object", "Embedded Message Name"="nidevice_grpc_Session", "Protobuf Index"=2, "MessageElementType"=enum."MessageValue", "Repeated"=FALSE, "Is in Oneof"=FALSE, "Oneof Container Name"=""}, {"Field Name"="object_class", "Embedded Message Name"="", "Protobuf Index"=3, "MessageElementType"=enum."UInt32Value", "Repeated"=FALSE, "Is in Oneof"=FALSE, "Oneof Container Name"=""}, {"Field Name"="object_name", "Embedded Message Name"="", "Protobuf Index"=4, "MessageElementType"=enum."StringValue", "Repeated"=FALSE, "Is in Oneof"=FALSE, "Oneof Container Name"=""}], "Has Oneof"=FALSE}, {"Version"=2, "Name"="nixnet_grpc_DbFindObjectResponse", "Type Url"="nixnet_grpc.DbFindObjectResponse", "Elements"=[{"Field Name"="status", "Embedded Message Name"="", "Protobuf Index"=1, "MessageElementType"=enum."Int32Value", "Repeated"=FALSE, "Is in Oneof"=FALSE, "Oneof Container Name"=""}, {"Field Name"="db_object", "Embedded Message Name"="nidevice_grpc_Session", "Protobuf Index"=2, "MessageElementType"=enum."MessageValue", "Repeated"=FALSE, "Is in Oneof"=FALSE, "Oneof Container Name"=""}], "Has Oneof"=FALSE}, {"Version"=2, "Name"="nixnet_grpc_DbGetDBCAttributeRequest", "Type Url"="nixnet_grpc.DbGetDBCAttributeRequest", "Elements"=[{"Field Name"="db_object", "Embedded Message Name"="nidevice_grpc_Session", "Protobuf Index"=1, "MessageElementType"=enum."MessageValue", "Repeated"=FALSE, "Is in Oneof"=FALSE, "Oneof Container Name"=""}, {"Field Name"="selected_index", "Embedded Message Name"="", "Protobuf Index"=-1, "MessageElementType"=enum."Int32Value", "Repeated"=FALSE, "Is in Oneof"=TRUE, "Oneof Container Name"="nixnet_grpc_DbGetDBCAttributeRequest_mode_enum"}, {"Field Name"="mode", "Embedded Message Name"="nixnet_grpc_GetDBCAttributeMode", "Protobuf Index"=2, "MessageElementType"=enum."EnumValue", "Repeated"=FALSE, "Is in Oneof"=TRUE, "Oneof Container Name"="nixnet_grpc_DbGetDBCAttributeRequest_mode_enum"}, {"Field Name"="mode_raw", "Embedded Message Name"="", "Protobuf Index"=3, "MessageElementType"=enum."UInt32Value", "Repeated"=FALSE, "Is in Oneof"=TRUE, "Oneof Container Name"="nixnet_grpc_DbGetDBCAttributeRequest_mode_enum"}, {"Field Name"="attribute_name", "Embedded Message Name"="", "Protobuf Index"=4, "MessageElementType"=enum."StringValue", "Repeated"=FALSE, "Is in Oneof"=FALSE, "Oneof Container Name"=""}], "Has Oneof"=TRUE}, {"Version"=2, "Name"="nixnet_grpc_DbGetDBCAttributeResponse", "Type Url"="nixnet_grpc.DbGetDBCAttributeResponse", "Elements"=[{"Field Name"="status", "Embedded Message Name"="", "Protobuf Index"=1, "MessageElementType"=enum."Int32Value", "Repeated"=FALSE, "Is in Oneof"=FALSE, "Oneof Container Name"=""}, {"Field Name"="attribute_text", "Embedded Message Name"="", "Protobuf Index"=2, "MessageElementType"=enum."StringValue", "Repeated"=FALSE, "Is in Oneof"=FALSE, "Oneof Container Name"=""}, {"Field Name"="is_default", "Embedded Message Name"="", "Protobuf Index"=3, "MessageElementType"=enum."UInt32Value", "Repeated"=FALSE, "Is in Oneof"=FALSE, "Oneof Container Name"=""}], "Has Oneof"=FALSE}, {"Version"=2, "Name"="nixnet_grpc_DbGetDBCAttributeSizeRequest", "Type Url"="nixnet_grpc.DbGetDBCAttributeSizeRequest", "Elements"=[{"Field Name"="db_object", "Embedded Message Name"="nidevice_grpc_Session", "Protobuf Index"=1, "MessageElementType"=enum."MessageValue", "Repeated"=FALSE, "Is in Oneof"=FALSE, "Oneof Container Name"=""}, {"Field Name"="selected_index", "Embedded Message Name"="", "Protobuf Index"=-1, "MessageElementType"=enum."Int32Value", "Repeated"=FALSE, "Is in Oneof"=TRUE, "Oneof Container Name"="nixnet_grpc_DbGetDBCAttributeSizeRequest_mode_enum"}, {"Field Name"="mode", "Embedded Message Name"="nixnet_grpc_GetDBCAttributeMode", "Protobuf Index"=2, "MessageElementType"=enum."EnumValue", "Repeated"=FALSE, "Is in Oneof"=TRUE, "Oneof Container Name"="nixnet_grpc_DbGetDBCAttributeSizeRequest_mode_enum"}, {"Field Name"="mode_raw", "Embedded Message Name"="", "Protobuf Index"=3, "MessageElementType"=enum."UInt32Value", "Repeated"=FALSE, "Is in Oneof"=TRUE, "Oneof Container Name"="nixnet_grpc_DbGetDBCAttributeSizeRequest_mode_enum"}, {"Field Name"="attribute_name", "Embedded Message Name"="", "Protobuf Index"=4, "MessageElementType"=enum."StringValue", "Repeated"=FALSE, "Is in Oneof"=FALSE, "Oneof Container Name"=""}], "Has Oneof"=TRUE}, {"Version"=2, "Name"="nixnet_grpc_DbGetDBCAttributeSizeResponse", "Type Url"="nixnet_grpc.DbGetDBCAttributeSizeResponse", "Elements"=[{"Field Name"="status", "Embedded Message Name"="", "Protobuf Index"=1, "MessageElementType"=enum."Int32Value", "Repeated"=FALSE, "Is in Oneof"=FALSE, "Oneof Container Name"=""}, {"Field Name"="attribute_text_size", "Embedded Message Name"="", "Protobuf Index"=2, "MessageElementType"=enum."UInt32Value", "Repeated"=FALSE, "Is in Oneof"=FALSE, "Oneof Container Name"=""}], "Has Oneof"=FALSE}, {"Version"=2, "Name"="nixnet_grpc_DbGetDatabaseListRequest", "Type Url"="nixnet_grpc.DbGetDatabaseListRequest", "Elements"=[{"Field Name"="ip_address", "Embedded Message Name"="", "Protobuf Index"=1, "MessageElementType"=enum."StringValue", "Repeated"=FALSE, "Is in Oneof"=FALSE, "Oneof Container Name"=""}], "Has Oneof"=FALSE}, {"Version"=2, "Name"="nixnet_grpc_DbGetDatabaseListResponse", "Type Url"="nixnet_grpc.DbGetDatabaseListResponse", "Elements"=[{"Field Name"="status", "Embedded Message Name"="", "Protobuf Index"=1, "MessageElementType"=enum."Int32Value", "Repeated"=FALSE, "Is in Oneof"=FALSE, "Oneof Container Name"=""}, {"Field Name"="alias_buffer", "Embedded Message Name"="", "Protobuf Index"=2, "MessageElementType"=enum."StringValue", "Repeated"=FALSE, "Is in Oneof"=FALSE, "Oneof Container Name"=""}, {"Field Name"="filepath_buffer", "Embedded Message Name"="", "Protobuf Index"=3, "MessageElementType"=enum."StringValue", "Repeated"=FALSE, "Is in Oneof"=FALSE, "Oneof Container Name"=""}, {"Field Name"="number_of_databases", "Embedded Message Name"="", "Protobuf Index"=4, "MessageElementType"=enum."UInt32Value", "Repeated"=FALSE, "Is in Oneof"=FALSE, "Oneof Container Name"=""}], "Has Oneof"=FALSE}, {"Version"=2, "Name"="nixnet_grpc_DbGetDatabaseListSizesRequest", "Type Url"="nixnet_grpc.DbGetDatabaseListSizesRequest", "Elements"=[{"Field Name"="ip_address", "Embedded Message Name"="", "Protobuf Index"=1, "MessageElementType"=enum."StringValue", "Repeated"=FALSE, "Is in Oneof"=FALSE, "Oneof Container Name"=""}], "Has Oneof"=FALSE}, {"Version"=2, "Name"="nixnet_grpc_DbGetDatabaseListSizesResponse", "Type Url"="nixnet_grpc.DbGetDatabaseListSizesResponse", "Elements"=[{"Field Name"="status", "Embedded Message Name"="", "Protobuf Index"=1, "MessageElementType"=enum."Int32Value", "Repeated"=FALSE, "Is in Oneof"=FALSE, "Oneof Container Name"=""}, {"Field Name"="sizeof_alias_buffer", "Embedded Message Name"="", "Protobuf Index"=2, "MessageElementType"=enum."UInt32Value", "Repeated"=FALSE, "Is in Oneof"=FALSE, "Oneof Container Name"=""}, {"Field Name"="sizeof_filepath_buffer", "Embedded Message Name"="", "Protobuf Index"=3, "MessageElementType"=enum."UInt32Value", "Repeated"=FALSE, "Is in Oneof"=FALSE, "Oneof Container Name"=""}], "Has Oneof"=FALSE}, {"Version"=2, "Name"="nixnet_grpc_DbGetPropertySizeRequest", "Type Url"="nixnet_grpc.DbGetPropertySizeRequest", "Elements"=[{"Field Name"="db_object", "Embedded Message Name"="nidevice_grpc_Session", "Protobuf Index"=1, "MessageElementType"=enum."MessageValue", "Repeated"=FALSE, "Is in Oneof"=FALSE, "Oneof Container Name"=""}, {"Field Name"="selected_index", "Embedded Message Name"="", "Protobuf Index"=-1, "MessageElementType"=enum."Int32Value", "Repeated"=FALSE, "Is in Oneof"=TRUE, "Oneof Container Name"="nixnet_grpc_DbGetPropertySizeRequest_property_id_enum"}, {"Field Name"="property_id", "Embedded Message Name"="nixnet_grpc_DBProperty", "Protobuf Index"=2, "MessageElementType"=enum."EnumValue", "Repeated"=FALSE, "Is in Oneof"=TRUE, "Oneof Container Name"="nixnet_grpc_DbGetPropertySizeRequest_property_id_enum"}, {"Field Name"="property_id_raw", "Embedded Message Name"="", "Protobuf Index"=3, "MessageElementType"=enum."UInt32Value", "Repeated"=FALSE, "Is in Oneof"=TRUE, "Oneof Container Name"="nixnet_grpc_DbGetPropertySizeRequest_property_id_enum"}], "Has Oneof"=TRUE}, {"Version"=2, "Name"="nixnet_grpc_DbGetPropertySizeResponse", "Type Url"="nixnet_grpc.DbGetPropertySizeResponse", "Elements"=[{"Field Name"="status", "Embedded Message Name"="", "Protobuf Index"=1, "MessageElementType"=enum."Int32Value", "Repeated"=FALSE, "Is in Oneof"=FALSE, "Oneof Container Name"=""}, {"Field Name"="property_size", "Embedded Message Name"="", "Protobuf Index"=2, "MessageElementType"=enum."UInt32Value", "Repeated"=FALSE, "Is in Oneof"=FALSE, "Oneof Container Name"=""}], "Has Oneof"=FALSE}, {"Version"=2, "Name"="nixnet_grpc_DbMergeRequest", "Type Url"="nixnet_grpc.DbMergeRequest", "Elements"=[{"Field Name"="target_cluster", "Embedded Message Name"="nidevice_grpc_Session", "Protobuf Index"=1, "MessageElementType"=enum."MessageValue", "Repeated"=FALSE, "Is in Oneof"=FALSE, "Oneof Container Name"=""}, {"Field Name"="source_obj", "Embedded Message Name"="nidevice_grpc_Session", "Protobuf Index"=2, "MessageElementType"=enum."MessageValue", "Repeated"=FALSE, "Is in Oneof"=FALSE, "Oneof Container Name"=""}, {"Field Name"="selected_index", "Embedded Message Name"="", "Protobuf Index"=-1, "MessageElementType"=enum."Int32Value", "Repeated"=FALSE, "Is in Oneof"=TRUE, "Oneof Container Name"="nixnet_grpc_DbMergeRequest_copy_mode_enum"}, {"Field Name"="copy_mode", "Embedded Message Name"="nixnet_grpc_CopyMode", "Protobuf Index"=3, "MessageElementType"=enum."EnumValue", "Repeated"=FALSE, "Is in Oneof"=TRUE, "Oneof Container Name"="nixnet_grpc_DbMergeRequest_copy_mode_enum"}, {"Field Name"="copy_mode_raw", "Embedded Message Name"="", "Protobuf Index"=4, "MessageElementType"=enum."UInt32Value", "Repeated"=FALSE, "Is in Oneof"=TRUE, "Oneof Container Name"="nixnet_grpc_DbMergeRequest_copy_mode_enum"}, {"Field Name"="prefix", "Embedded Message Name"="", "Protobuf Index"=5, "MessageElementType"=enum."StringValue", "Repeated"=FALSE, "Is in Oneof"=FALSE, "Oneof Container Name"=""}, {"Field Name"="wait_for_complete", "Embedded Message Name"="", "Protobuf Index"=6, "MessageElementType"=enum."UInt32Value", "Repeated"=FALSE, "Is in Oneof"=FALSE, "Oneof Container Name"=""}], "Has Oneof"=TRUE}, {"Version"=2, "Name"="nixnet_grpc_DbMergeResponse", "Type Url"="nixnet_grpc.DbMergeResponse", "Elements"=[{"Field Name"="status", "Embedded Message Name"="", "Protobuf Index"=1, "MessageElementType"=enum."Int32Value", "Repeated"=FALSE, "Is in Oneof"=FALSE, "Oneof Container Name"=""}, {"Field Name"="percent_complete", "Embedded Message Name"="", "Protobuf Index"=2, "MessageElementType"=enum."UInt32Value", "Repeated"=FALSE, "Is in Oneof"=FALSE, "Oneof Container Name"=""}], "Has Oneof"=FALSE}, {"Version"=2, "Name"="nixnet_grpc_DbOpenDatabaseRequest", "Type Url"="nixnet_grpc.DbOpenDatabaseRequest", "Elements"=[{"Field Name"="session_name", "Embedded Message Name"="", "Protobuf Index"=1, "MessageElementType"=enum."StringValue", "Repeated"=FALSE, "Is in Oneof"=FALSE, "Oneof Container Name"=""}, {"Field Name"="database_name", "Embedded Message Name"="", "Protobuf Index"=2, "MessageElementType"=enum."StringValue", "Repeated"=FALSE, "Is in Oneof"=FALSE, "Oneof Container Name"=""}, {"Field Name"="initialization_behavior", "Embedded Message Name"="nidevice_grpc_SessionInitializationBehavior", "Protobuf Index"=3, "MessageElementType"=enum."EnumValue", "Repeated"=FALSE, "Is in Oneof"=FALSE, "Oneof Container Name"=""}], "Has Oneof"=FALSE}, {"Version"=2, "Name"="nixnet_grpc_DbOpenDatabaseResponse", "Type Url"="nixnet_grpc.DbOpenDatabaseResponse", "Elements"=[{"Field Name"="status", "Embedded Message Name"="", "Protobuf Index"=1, "MessageElementType"=enum."Int32Value", "Repeated"=FALSE, "Is in Oneof"=FALSE, "Oneof Container Name"=""}, {"Field Name"="database", "Embedded Message Name"="nidevice_grpc_Session", "Protobuf Index"=2, "MessageElementType"=enum."MessageValue", "Repeated"=FALSE, "Is in Oneof"=FALSE, "Oneof Container Name"=""}, {"Field Name"="new_session_initialized", "Embedded Message Name"="", "Protobuf Index"=3, "MessageElementType"=enum."BoolValue", "Repeated"=FALSE, "Is in Oneof"=FALSE, "Oneof Container Name"=""}], "Has Oneof"=FALSE}, {"Version"=2, "Name"="nixnet_grpc_DbRemoveAliasRequest", "Type Url"="nixnet_grpc.DbRemoveAliasRequest", "Elements"=[{"Field Name"="database_alias", "Embedded Message Name"="", "Protobuf Index"=1, "MessageElementType"=enum."StringValue", "Repeated"=FALSE, "Is in Oneof"=FALSE, "Oneof Container Name"=""}], "Has Oneof"=FALSE}, {"Version"=2, "Name"="nixnet_grpc_DbRemoveAliasResponse", "Type Url"="nixnet_grpc.DbRemoveAliasResponse", "Elements"=[{"Field Name"="status", "Embedded Message Name"="", "Protobuf Index"=1, "MessageElementType"=enum."Int32Value", "Repeated"=FALSE, "Is in Oneof"=FALSE, "Oneof Container Name"=""}], "Has Oneof"=FALSE}, {"Version"=2, "Name"="nixnet_grpc_DbSaveDatabaseRequest", "Type Url"="nixnet_grpc.DbSaveDatabaseRequest", "Elements"=[{"Field Name"="database", "Embedded Message Name"="nidevice_grpc_Session", "Protobuf Index"=1, "MessageElementType"=enum."MessageValue", "Repeated"=FALSE, "Is in Oneof"=FALSE, "Oneof Container Name"=""}, {"Field Name"="db_filepath", "Embedded Message Name"="", "Protobuf Index"=2, "MessageElementType"=enum."StringValue", "Repeated"=FALSE, "Is in Oneof"=FALSE, "Oneof Container Name"=""}], "Has Oneof"=FALSE}, {"Version"=2, "Name"="nixnet_grpc_DbSaveDatabaseResponse", "Type Url"="nixnet_grpc.DbSaveDatabaseResponse", "Elements"=[{"Field Name"="status", "Embedded Message Name"="", "Protobuf Index"=1, "MessageElementType"=enum."Int32Value", "Repeated"=FALSE, "Is in Oneof"=FALSE, "Oneof Container Name"=""}], "Has Oneof"=FALSE}, {"Version"=2, "Name"="nixnet_grpc_DbUndeployRequest", "Type Url"="nixnet_grpc.DbUndeployRequest", "Elements"=[{"Field Name"="ip_address", "Embedded Message Name"="", "Protobuf Index"=1, "MessageElementType"=enum."StringValue", "Repeated"=FALSE, "Is in Oneof"=FALSE, "Oneof Container Name"=""}, {"Field Name"="database_alias", "Embedded Message Name"="", "Protobuf Index"=2, "MessageElementType"=enum."StringValue", "Repeated"=FALSE, "Is in Oneof"=FALSE, "Oneof Container Name"=""}], "Has Oneof"=FALSE}, {"Version"=2, "Name"="nixnet_grpc_DbUndeployResponse", "Type Url"="nixnet_grpc.DbUndeployResponse", "Elements"=[{"Field Name"="status", "Embedded Message Name"="", "Protobuf Index"=1, "MessageElementType"=enum."Int32Value", "Repeated"=FALSE, "Is in Oneof"=FALSE, "Oneof Container Name"=""}], "Has Oneof"=FALSE}, {"Version"=2, "Name"="nixnet_grpc_DisconnectTerminalsRequest", "Type Url"="nixnet_grpc.DisconnectTerminalsRequest", "Elements"=[{"Field Name"="session", "Embedded Message Name"="nidevice_grpc_Session", "Protobuf Index"=1, "MessageElementType"=enum."MessageValue", "Repeated"=FALSE, "Is in Oneof"=FALSE, "Oneof Container Name"=""}, {"Field Name"="selected_index", "Embedded Message Name"="", "Protobuf Index"=-1, "MessageElementType"=enum."Int32Value", "Repeated"=FALSE, "Is in Oneof"=TRUE, "Oneof Container Name"="nixnet_grpc_DisconnectTerminalsRequest_source_enum"}, {"Field Name"="source_mapped", "Embedded Message Name"="nixnet_grpc_TerminalName", "Protobuf Index"=2, "MessageElementType"=enum."EnumValue", "Repeated"=FALSE, "Is in Oneof"=TRUE, "Oneof Container Name"="nixnet_grpc_DisconnectTerminalsRequest_source_enum"}, {"Field Name"="source_raw", "Embedded Message Name"="", "Protobuf Index"=3, "MessageElementType"=enum."StringValue", "Repeated"=FALSE, "Is in Oneof"=TRUE, "Oneof Container Name"="nixnet_grpc_DisconnectTerminalsRequest_source_enum"}, {"Field Name"="selected_index", "Embedded Message Name"="", "Protobuf Index"=-1, "MessageElementType"=enum."Int32Value", "Repeated"=FALSE, "Is in Oneof"=TRUE, "Oneof Container Name"="nixnet_grpc_DisconnectTerminalsRequest_destination_enum"}, {"Field Name"="destination_mapped", "Embedded Message Name"="nixnet_grpc_TerminalName", "Protobuf Index"=4, "MessageElementType"=enum."EnumValue", "Repeated"=FALSE, "Is in Oneof"=TRUE, "Oneof Container Name"="nixnet_grpc_DisconnectTerminalsRequest_destination_enum"}, {"Field Name"="destination_raw", "Embedded Message Name"="", "Protobuf Index"=5, "MessageElementType"=enum."StringValue", "Repeated"=FALSE, "Is in Oneof"=TRUE, "Oneof Container Name"="nixnet_grpc_DisconnectTerminalsRequest_destination_enum"}], "Has Oneof"=TRUE}, {"Version"=2, "Name"="nixnet_grpc_DisconnectTerminalsResponse", "Type Url"="nixnet_grpc.DisconnectTerminalsResponse", "Elements"=[{"Field Name"="status", "Embedded Message Name"="", "Protobuf Index"=1, "MessageElementType"=enum."Int32Value", "Repeated"=FALSE, "Is in Oneof"=FALSE, "Oneof Container Name"=""}], "Has Oneof"=FALSE}, {"Version"=2, "Name"="nixnet_grpc_FlushRequest", "Type Url"="nixnet_grpc.FlushRequest", "Elements"=[{"Field Name"="session", "Embedded Message Name"="nidevice_grpc_Session", "Protobuf Index"=1, "MessageElementType"=enum."MessageValue", "Repeated"=FALSE, "Is in Oneof"=FALSE, "Oneof Container Name"=""}], "Has Oneof"=FALSE}, {"Version"=2, "Name"="nixnet_grpc_FlushResponse", "Type Url"="nixnet_grpc.FlushResponse", "Elements"=[{"Field Name"="status", "Embedded Message Name"="", "Protobuf Index"=1, "MessageElementType"=enum."Int32Value", "Repeated"=FALSE, "Is in Oneof"=FALSE, "Oneof Container Name"=""}], "Has Oneof"=FALSE}, {"Version"=2, "Name"="nixnet_grpc_FutureTimeTriggerRequest", "Type Url"="nixnet_grpc.FutureTimeTriggerRequest", "Elements"=[{"Field Name"="session", "Embedded Message Name"="nidevice_grpc_Session", "Protobuf Index"=1, "MessageElementType"=enum."MessageValue", "Repeated"=FALSE, "Is in Oneof"=FALSE, "Oneof Container Name"=""}, {"Field Name"="when", "Embedded Message Name"="", "Protobuf Index"=2, "MessageElementType"=enum."UInt64Value", "Repeated"=FALSE, "Is in Oneof"=FALSE, "Oneof Container Name"=""}, {"Field Name"="selected_index", "Embedded Message Name"="", "Protobuf Index"=-1, "MessageElementType"=enum."Int32Value", "Repeated"=FALSE, "Is in Oneof"=TRUE, "Oneof Container Name"="nixnet_grpc_FutureTimeTriggerRequest_timescale_enum"}, {"Field Name"="timescale", "Embedded Message Name"="nixnet_grpc_TimeScale", "Protobuf Index"=3, "MessageElementType"=enum."EnumValue", "Repeated"=FALSE, "Is in Oneof"=TRUE, "Oneof Container Name"="nixnet_grpc_FutureTimeTriggerRequest_timescale_enum"}, {"Field Name"="timescale_raw", "Embedded Message Name"="", "Protobuf Index"=4, "MessageElementType"=enum."UInt32Value", "Repeated"=FALSE, "Is in Oneof"=TRUE, "Oneof Container Name"="nixnet_grpc_FutureTimeTriggerRequest_timescale_enum"}], "Has Oneof"=TRUE}, {"Version"=2, "Name"="nixnet_grpc_FutureTimeTriggerResponse", "Type Url"="nixnet_grpc.FutureTimeTriggerResponse", "Elements"=[{"Field Name"="status", "Embedded Message Name"="", "Protobuf Index"=1, "MessageElementType"=enum."Int32Value", "Repeated"=FALSE, "Is in Oneof"=FALSE, "Oneof Container Name"=""}], "Has Oneof"=FALSE}, {"Version"=2, "Name"="nixnet_grpc_GetPropertySizeRequest", "Type Url"="nixnet_grpc.GetPropertySizeRequest", "Elements"=[{"Field Name"="session", "Embedded Message Name"="nidevice_grpc_Session", "Protobuf Index"=1, "MessageElementType"=enum."MessageValue", "Repeated"=FALSE, "Is in Oneof"=FALSE, "Oneof Container Name"=""}, {"Field Name"="selected_index", "Embedded Message Name"="", "Protobuf Index"=-1, "MessageElementType"=enum."Int32Value", "Repeated"=FALSE, "Is in Oneof"=TRUE, "Oneof Container Name"="nixnet_grpc_GetPropertySizeRequest_property_id_enum"}, {"Field Name"="property_id", "Embedded Message Name"="nixnet_grpc_Property", "Protobuf Index"=2, "MessageElementType"=enum."EnumValue", "Repeated"=FALSE, "Is in Oneof"=TRUE, "Oneof Container Name"="nixnet_grpc_GetPropertySizeRequest_property_id_enum"}, {"Field Name"="property_id_raw", "Embedded Message Name"="", "Protobuf Index"=3, "MessageElementType"=enum."UInt32Value", "Repeated"=FALSE, "Is in Oneof"=TRUE, "Oneof Container Name"="nixnet_grpc_GetPropertySizeRequest_property_id_enum"}], "Has Oneof"=TRUE}, {"Version"=2, "Name"="nixnet_grpc_GetPropertySizeResponse", "Type Url"="nixnet_grpc.GetPropertySizeResponse", "Elements"=[{"Field Name"="status", "Embedded Message Name"="", "Protobuf Index"=1, "MessageElementType"=enum."Int32Value", "Repeated"=FALSE, "Is in Oneof"=FALSE, "Oneof Container Name"=""}, {"Field Name"="property_size", "Embedded Message Name"="", "Protobuf Index"=2, "MessageElementType"=enum."UInt32Value", "Repeated"=FALSE, "Is in Oneof"=FALSE, "Oneof Container Name"=""}], "Has Oneof"=FALSE}, {"Version"=2, "Name"="nixnet_grpc_GetSubPropertySizeRequest", "Type Url"="nixnet_grpc.GetSubPropertySizeRequest", "Elements"=[{"Field Name"="session", "Embedded Message Name"="nidevice_grpc_Session", "Protobuf Index"=1, "MessageElementType"=enum."MessageValue", "Repeated"=FALSE, "Is in Oneof"=FALSE, "Oneof Container Name"=""}, {"Field Name"="active_index", "Embedded Message Name"="", "Protobuf Index"=2, "MessageElementType"=enum."UInt32Value", "Repeated"=FALSE, "Is in Oneof"=FALSE, "Oneof Container Name"=""}, {"Field Name"="selected_index", "Embedded Message Name"="", "Protobuf Index"=-1, "MessageElementType"=enum."Int32Value", "Repeated"=FALSE, "Is in Oneof"=TRUE, "Oneof Container Name"="nixnet_grpc_GetSubPropertySizeRequest_property_id_enum"}, {"Field Name"="property_id", "Embedded Message Name"="nixnet_grpc_SubProperty", "Protobuf Index"=3, "MessageElementType"=enum."EnumValue", "Repeated"=FALSE, "Is in Oneof"=TRUE, "Oneof Container Name"="nixnet_grpc_GetSubPropertySizeRequest_property_id_enum"}, {"Field Name"="property_id_raw", "Embedded Message Name"="", "Protobuf Index"=4, "MessageElementType"=enum."UInt32Value", "Repeated"=FALSE, "Is in Oneof"=TRUE, "Oneof Container Name"="nixnet_grpc_GetSubPropertySizeRequest_property_id_enum"}], "Has Oneof"=TRUE}, {"Version"=2, "Name"="nixnet_grpc_GetSubPropertySizeResponse", "Type Url"="nixnet_grpc.GetSubPropertySizeResponse", "Elements"=[{"Field Name"="status", "Embedded Message Name"="", "Protobuf Index"=1, "MessageElementType"=enum."Int32Value", "Repeated"=FALSE, "Is in Oneof"=FALSE, "Oneof Container Name"=""}, {"Field Name"="property_size", "Embedded Message Name"="", "Protobuf Index"=2, "MessageElementType"=enum."UInt32Value", "Repeated"=FALSE, "Is in Oneof"=FALSE, "Oneof Container Name"=""}], "Has Oneof"=FALSE}, {"Version"=2, "Name"="nixnet_grpc_ReadFrameRequest", "Type Url"="nixnet_grpc.ReadFrameRequest", "Elements"=[{"Field Name"="session", "Embedded Message Name"="nidevice_grpc_Session", "Protobuf Index"=1, "MessageElementType"=enum."MessageValue", "Repeated"=FALSE, "Is in Oneof"=FALSE, "Oneof Container Name"=""}, {"Field Name"="number_of_frames", "Embedded Message Name"="", "Protobuf Index"=2, "MessageElementType"=enum."Int32Value", "Repeated"=FALSE, "Is in Oneof"=FALSE, "Oneof Container Name"=""}, {"Field Name"="max_payload_per_frame", "Embedded Message Name"="", "Protobuf Index"=3, "MessageElementType"=enum."UInt32Value", "Repeated"=FALSE, "Is in Oneof"=FALSE, "Oneof Container Name"=""}, {"Field Name"="selected_index", "Embedded Message Name"="", "Protobuf Index"=-1, "MessageElementType"=enum."Int32Value", "Repeated"=FALSE, "Is in Oneof"=TRUE, "Oneof Container Name"="nixnet_grpc_ReadFrameRequest_protocol_enum"}, {"Field Name"="protocol", "Embedded Message Name"="nixnet_grpc_Protocol", "Protobuf Index"=4, "MessageElementType"=enum."EnumValue", "Repeated"=FALSE, "Is in Oneof"=TRUE, "Oneof Container Name"="nixnet_grpc_ReadFrameRequest_protocol_enum"}, {"Field Name"="protocol_raw", "Embedded Message Name"="", "Protobuf Index"=5, "MessageElementType"=enum."UInt32Value", "Repeated"=FALSE, "Is in Oneof"=TRUE, "Oneof Container Name"="nixnet_grpc_ReadFrameRequest_protocol_enum"}, {"Field Name"="selected_index", "Embedded Message Name"="", "Protobuf Index"=-1, "MessageElementType"=enum."Int32Value", "Repeated"=FALSE, "Is in Oneof"=TRUE, "Oneof Container Name"="nixnet_grpc_ReadFrameRequest_timeout_enum"}, {"Field Name"="timeout", "Embedded Message Name"="nixnet_grpc_TimeOut", "Protobuf Index"=6, "MessageElementType"=enum."EnumValue", "Repeated"=FALSE, "Is in Oneof"=TRUE, "Oneof Container Name"="nixnet_grpc_ReadFrameRequest_timeout_enum"}, {"Field Name"="timeout_raw", "Embedded Message Name"="", "Protobuf Index"=7, "MessageElementType"=enum."DoubleValue", "Repeated"=FALSE, "Is in Oneof"=TRUE, "Oneof Container Name"="nixnet_grpc_ReadFrameRequest_timeout_enum"}], "Has Oneof"=TRUE}, {"Version"=2, "Name"="nixnet_grpc_ReadFrameResponse", "Type Url"="nixnet_grpc.ReadFrameResponse", "Elements"=[{"Field Name"="status", "Embedded Message Name"="", "Protobuf Index"=1, "MessageElementType"=enum."Int32Value", "Repeated"=FALSE, "Is in Oneof"=FALSE, "Oneof Container Name"=""}, {"Field Name"="buffer", "Embedded Message Name"="nixnet_grpc_FrameBufferResponse", "Protobuf Index"=2, "MessageElementType"=enum."MessageValue", "Repeated"=TRUE, "Is in Oneof"=FALSE, "Oneof Container Name"=""}], "Has Oneof"=FALSE}, {"Version"=2, "Name"="nixnet_grpc_ReadSignalSinglePointRequest", "Type Url"="nixnet_grpc.ReadSignalSinglePointRequest", "Elements"=[{"Field Name"="session", "Embedded Message Name"="nidevice_grpc_Session", "Protobuf Index"=1, "MessageElementType"=enum."MessageValue", "Repeated"=FALSE, "Is in Oneof"=FALSE, "Oneof Container Name"=""}, {"Field Name"="number_of_signals", "Embedded Message Name"="", "Protobuf Index"=2, "MessageElementType"=enum."UInt32Value", "Repeated"=FALSE, "Is in Oneof"=FALSE, "Oneof Container Name"=""}], "Has Oneof"=FALSE}, {"Version"=2, "Name"="nixnet_grpc_ReadSignalSinglePointResponse", "Type Url"="nixnet_grpc.ReadSignalSinglePointResponse", "Elements"=[{"Field Name"="status", "Embedded Message Name"="", "Protobuf Index"=1, "MessageElementType"=enum."Int32Value", "Repeated"=FALSE, "Is in Oneof"=FALSE, "Oneof Container Name"=""}, {"Field Name"="value_buffer", "Embedded Message Name"="", "Protobuf Index"=2, "MessageElementType"=enum."DoubleValue", "Repeated"=TRUE, "Is in Oneof"=FALSE, "Oneof Container Name"=""}, {"Field Name"="timestamp_buffer", "Embedded Message Name"="", "Protobuf Index"=3, "MessageElementType"=enum."UInt64Value", "Repeated"=TRUE, "Is in Oneof"=FALSE, "Oneof Container Name"=""}], "Has Oneof"=FALSE}, {"Version"=2, "Name"="nixnet_grpc_ReadSignalWaveformRequest", "Type Url"="nixnet_grpc.ReadSignalWaveformRequest", "Elements"=[{"Field Name"="session", "Embedded Message Name"="nidevice_grpc_Session", "Protobuf Index"=1, "MessageElementType"=enum."MessageValue", "Repeated"=FALSE, "Is in Oneof"=FALSE, "Oneof Container Name"=""}, {"Field Name"="selected_index", "Embedded Message Name"="", "Protobuf Index"=-1, "MessageElementType"=enum."Int32Value", "Repeated"=FALSE, "Is in Oneof"=TRUE, "Oneof Container Name"="nixnet_grpc_ReadSignalWaveformRequest_timeout_enum"}, {"Field Name"="timeout", "Embedded Message Name"="nixnet_grpc_TimeOut", "Protobuf Index"=2, "MessageElementType"=enum."EnumValue", "Repeated"=FALSE, "Is in Oneof"=TRUE, "Oneof Container Name"="nixnet_grpc_ReadSignalWaveformRequest_timeout_enum"}, {"Field Name"="timeout_raw", "Embedded Message Name"="", "Protobuf Index"=3, "MessageElementType"=enum."DoubleValue", "Repeated"=FALSE, "Is in Oneof"=TRUE, "Oneof Container Name"="nixnet_grpc_ReadSignalWaveformRequest_timeout_enum"}, {"Field Name"="samples_per_signal", "Embedded Message Name"="", "Protobuf Index"=4, "MessageElementType"=enum."UInt32Value", "Repeated"=FALSE, "Is in Oneof"=FALSE, "Oneof Container Name"=""}, {"Field Name"="number_of_signals", "Embedded Message Name"="", "Protobuf Index"=5, "MessageElementType"=enum."UInt32Value", "Repeated"=FALSE, "Is in Oneof"=FALSE, "Oneof Container Name"=""}], "Has Oneof"=TRUE}, {"Version"=2, "Name"="nixnet_grpc_ReadSignalWaveformResponse", "Type Url"="nixnet_grpc.ReadSignalWaveformResponse", "Elements"=[{"Field Name"="status", "Embedded Message Name"="", "Protobuf Index"=1, "MessageElementType"=enum."Int32Value", "Repeated"=FALSE, "Is in Oneof"=FALSE, "Oneof Container Name"=""}, {"Field Name"="start_time", "Embedded Message Name"="", "Protobuf Index"=2, "MessageElementType"=enum."UInt64Value", "Repeated"=FALSE, "Is in Oneof"=FALSE, "Oneof Container Name"=""}, {"Field Name"="delta_time", "Embedded Message Name"="", "Protobuf Index"=3, "MessageElementType"=enum."DoubleValue", "Repeated"=FALSE, "Is in Oneof"=FALSE, "Oneof Container Name"=""}, {"Field Name"="value_buffer", "Embedded Message Name"="", "Protobuf Index"=4, "MessageElementType"=enum."DoubleValue", "Repeated"=TRUE, "Is in Oneof"=FALSE, "Oneof Container Name"=""}], "Has Oneof"=FALSE}, {"Version"=2, "Name"="nixnet_grpc_ReadSignalXYRequest", "Type Url"="nixnet_grpc.ReadSignalXYRequest", "Elements"=[{"Field Name"="session", "Embedded Message Name"="nidevice_grpc_Session", "Protobuf Index"=1, "MessageElementType"=enum."MessageValue", "Repeated"=FALSE, "Is in Oneof"=FALSE, "Oneof Container Name"=""}, {"Field Name"="time_limit", "Embedded Message Name"="", "Protobuf Index"=2, "MessageElementType"=enum."UInt64Value", "Repeated"=FALSE, "Is in Oneof"=FALSE, "Oneof Container Name"=""}, {"Field Name"="samples_per_signal", "Embedded Message Name"="", "Protobuf Index"=3, "MessageElementType"=enum."UInt32Value", "Repeated"=FALSE, "Is in Oneof"=FALSE, "Oneof Container Name"=""}, {"Field Name"="number_of_signals", "Embedded Message Name"="", "Protobuf Index"=4, "MessageElementType"=enum."UInt32Value", "Repeated"=FALSE, "Is in Oneof"=FALSE, "Oneof Container Name"=""}], "Has Oneof"=FALSE}, {"Version"=2, "Name"="nixnet_grpc_ReadSignalXYResponse", "Type Url"="nixnet_grpc.ReadSignalXYResponse", "Elements"=[{"Field Name"="status", "Embedded Message Name"="", "Protobuf Index"=1, "MessageElementType"=enum."Int32Value", "Repeated"=FALSE, "Is in Oneof"=FALSE, "Oneof Container Name"=""}, {"Field Name"="value_buffer", "Embedded Message Name"="", "Protobuf Index"=2, "MessageElementType"=enum."DoubleValue", "Repeated"=TRUE, "Is in Oneof"=FALSE, "Oneof Container Name"=""}, {"Field Name"="timestamp_buffer", "Embedded Message Name"="", "Protobuf Index"=3, "MessageElementType"=enum."UInt64Value", "Repeated"=TRUE, "Is in Oneof"=FALSE, "Oneof Container Name"=""}, {"Field Name"="num_pairs_buffer", "Embedded Message Name"="", "Protobuf Index"=4, "MessageElementType"=enum."UInt32Value", "Repeated"=TRUE, "Is in Oneof"=FALSE, "Oneof Container Name"=""}], "Has Oneof"=FALSE}, {"Version"=2, "Name"="nixnet_grpc_ReadStateRequest", "Type Url"="nixnet_grpc.ReadStateRequest", "Elements"=[{"Field Name"="session", "Embedded Message Name"="nidevice_grpc_Session", "Protobuf Index"=1, "MessageElementType"=enum."MessageValue", "Repeated"=FALSE, "Is in Oneof"=FALSE, "Oneof Container Name"=""}, {"Field Name"="selected_index", "Embedded Message Name"="", "Protobuf Index"=-1, "MessageElementType"=enum."Int32Value", "Repeated"=FALSE, "Is in Oneof"=TRUE, "Oneof Container Name"="nixnet_grpc_ReadStateRequest_state_id_enum"}, {"Field Name"="state_id", "Embedded Message Name"="nixnet_grpc_ReadState", "Protobuf Index"=2, "MessageElementType"=enum."EnumValue", "Repeated"=FALSE, "Is in Oneof"=TRUE, "Oneof Container Name"="nixnet_grpc_ReadStateRequest_state_id_enum"}, {"Field Name"="state_id_raw", "Embedded Message Name"="", "Protobuf Index"=3, "MessageElementType"=enum."UInt32Value", "Repeated"=FALSE, "Is in Oneof"=TRUE, "Oneof Container Name"="nixnet_grpc_ReadStateRequest_state_id_enum"}], "Has Oneof"=TRUE}, {"Version"=2, "Name"="nixnet_grpc_ReadStateResponse", "Type Url"="nixnet_grpc.ReadStateResponse", "Elements"=[{"Field Name"="status", "Embedded Message Name"="", "Protobuf Index"=1, "MessageElementType"=enum."Int32Value", "Repeated"=FALSE, "Is in Oneof"=FALSE, "Oneof Container Name"=""}, {"Field Name"="state_value", "Embedded Message Name"="nixnet_grpc_ReadStateValue", "Protobuf Index"=2, "MessageElementType"=enum."MessageValue", "Repeated"=FALSE, "Is in Oneof"=FALSE, "Oneof Container Name"=""}, {"Field Name"="fault", "Embedded Message Name"="", "Protobuf Index"=3, "MessageElementType"=enum."Int32Value", "Repeated"=FALSE, "Is in Oneof"=FALSE, "Oneof Container Name"=""}], "Has Oneof"=FALSE}, {"Version"=2, "Name"="nixnet_grpc_ReadStateTimeTriggerRequest", "Type Url"="nixnet_grpc.ReadStateTimeTriggerRequest", "Elements"=[{"Field Name"="session", "Embedded Message Name"="nidevice_grpc_Session", "Protobuf Index"=1, "MessageElementType"=enum."MessageValue", "Repeated"=FALSE, "Is in Oneof"=FALSE, "Oneof Container Name"=""}, {"Field Name"="selected_index", "Embedded Message Name"="", "Protobuf Index"=-1, "MessageElementType"=enum."Int32Value", "Repeated"=FALSE, "Is in Oneof"=TRUE, "Oneof Container Name"="nixnet_grpc_ReadStateTimeTriggerRequest_timeout_enum"}, {"Field Name"="timeout", "Embedded Message Name"="nixnet_grpc_TimeOut", "Protobuf Index"=2, "MessageElementType"=enum."EnumValue", "Repeated"=FALSE, "Is in Oneof"=TRUE, "Oneof Container Name"="nixnet_grpc_ReadStateTimeTriggerRequest_timeout_enum"}, {"Field Name"="timeout_raw", "Embedded Message Name"="", "Protobuf Index"=3, "MessageElementType"=enum."DoubleValue", "Repeated"=FALSE, "Is in Oneof"=TRUE, "Oneof Container Name"="nixnet_grpc_ReadStateTimeTriggerRequest_timeout_enum"}], "Has Oneof"=TRUE}, {"Version"=2, "Name"="nixnet_grpc_ReadStateTimeTriggerResponse", "Type Url"="nixnet_grpc.ReadStateTimeTriggerResponse", "Elements"=[{"Field Name"="status", "Embedded Message Name"="", "Protobuf Index"=1, "MessageElementType"=enum."Int32Value", "Repeated"=FALSE, "Is in Oneof"=FALSE, "Oneof Container Name"=""}, {"Field Name"="state_value", "Embedded Message Name"="nixnet_grpc_TimeLocalNetwork", "Protobuf Index"=2, "MessageElementType"=enum."MessageValue", "Repeated"=FALSE, "Is in Oneof"=FALSE, "Oneof Container Name"=""}], "Has Oneof"=FALSE}, {"Version"=2, "Name"="nixnet_grpc_StartRequest", "Type Url"="nixnet_grpc.StartRequest", "Elements"=[{"Field Name"="session", "Embedded Message Name"="nidevice_grpc_Session", "Protobuf Index"=1, "MessageElementType"=enum."MessageValue", "Repeated"=FALSE, "Is in Oneof"=FALSE, "Oneof Container Name"=""}, {"Field Name"="selected_index", "Embedded Message Name"="", "Protobuf Index"=-1, "MessageElementType"=enum."Int32Value", "Repeated"=FALSE, "Is in Oneof"=TRUE, "Oneof Container Name"="nixnet_grpc_StartRequest_scope_enum"}, {"Field Name"="scope", "Embedded Message Name"="nixnet_grpc_StartStopScope", "Protobuf Index"=2, "MessageElementType"=enum."EnumValue", "Repeated"=FALSE, "Is in Oneof"=TRUE, "Oneof Container Name"="nixnet_grpc_StartRequest_scope_enum"}, {"Field Name"="scope_raw", "Embedded Message Name"="", "Protobuf Index"=3, "MessageElementType"=enum."UInt32Value", "Repeated"=FALSE, "Is in Oneof"=TRUE, "Oneof Container Name"="nixnet_grpc_StartRequest_scope_enum"}], "Has Oneof"=TRUE}, {"Version"=2, "Name"="nixnet_grpc_StartResponse", "Type Url"="nixnet_grpc.StartResponse", "Elements"=[{"Field Name"="status", "Embedded Message Name"="", "Protobuf Index"=1, "MessageElementType"=enum."Int32Value", "Repeated"=FALSE, "Is in Oneof"=FALSE, "Oneof Container Name"=""}], "Has Oneof"=FALSE}, {"Version"=2, "Name"="nixnet_grpc_StatusToStringRequest", "Type Url"="nixnet_grpc.StatusToStringRequest", "Elements"=[{"Field Name"="status_id", "Embedded Message Name"="", "Protobuf Index"=1, "MessageElementType"=enum."Int32Value", "Repeated"=FALSE, "Is in Oneof"=FALSE, "Oneof Container Name"=""}], "Has Oneof"=FALSE}, {"Version"=2, "Name"="nixnet_grpc_StatusToStringResponse", "Type Url"="nixnet_grpc.StatusToStringResponse", "Elements"=[{"Field Name"="status", "Embedded Message Name"="", "Protobuf Index"=1, "MessageElementType"=enum."Int32Value", "Repeated"=FALSE, "Is in Oneof"=FALSE, "Oneof Container Name"=""}, {"Field Name"="status_description", "Embedded Message Name"="", "Protobuf Index"=2, "MessageElementType"=enum."StringValue", "Repeated"=FALSE, "Is in Oneof"=FALSE, "Oneof Container Name"=""}], "Has Oneof"=FALSE}, {"Version"=2, "Name"="nixnet_grpc_StopRequest", "Type Url"="nixnet_grpc.StopRequest", "Elements"=[{"Field Name"="session", "Embedded Message Name"="nidevice_grpc_Session", "Protobuf Index"=1, "MessageElementType"=enum."MessageValue", "Repeated"=FALSE, "Is in Oneof"=FALSE, "Oneof Container Name"=""}, {"Field Name"="selected_index", "Embedded Message Name"="", "Protobuf Index"=-1, "MessageElementType"=enum."Int32Value", "Repeated"=FALSE, "Is in Oneof"=TRUE, "Oneof Container Name"="nixnet_grpc_StopRequest_scope_enum"}, {"Field Name"="scope", "Embedded Message Name"="nixnet_grpc_StartStopScope", "Protobuf Index"=2, "MessageElementType"=enum."EnumValue", "Repeated"=FALSE, "Is in Oneof"=TRUE, "Oneof Container Name"="nixnet_grpc_StopRequest_scope_enum"}, {"Field Name"="scope_raw", "Embedded Message Name"="", "Protobuf Index"=3, "MessageElementType"=enum."UInt32Value", "Repeated"=FALSE, "Is in Oneof"=TRUE, "Oneof Container Name"="nixnet_grpc_StopRequest_scope_enum"}], "Has Oneof"=TRUE}, {"Version"=2, "Name"="nixnet_grpc_StopResponse", "Type Url"="nixnet_grpc.StopResponse", "Elements"=[{"Field Name"="status", "Embedded Message Name"="", "Protobuf Index"=1, "MessageElementType"=enum."Int32Value", "Repeated"=FALSE, "Is in Oneof"=FALSE, "Oneof Container Name"=""}], "Has Oneof"=FALSE}, {"Version"=2, "Name"="nixnet_grpc_SystemCloseRequest", "Type Url"="nixnet_grpc.SystemCloseRequest", "Elements"=[{"Field Name"="system", "Embedded Message Name"="nidevice_grpc_Session", "Protobuf Index"=1, "MessageElementType"=enum."MessageValue", "Repeated"=FALSE, "Is in Oneof"=FALSE, "Oneof Container Name"=""}], "Has Oneof"=FALSE}, {"Version"=2, "Name"="nixnet_grpc_SystemCloseResponse", "Type Url"="nixnet_grpc.SystemCloseResponse", "Elements"=[{"Field Name"="status", "Embedded Message Name"="", "Protobuf Index"=1, "MessageElementType"=enum."Int32Value", "Repeated"=FALSE, "Is in Oneof"=FALSE, "Oneof Container Name"=""}], "Has Oneof"=FALSE}, {"Version"=2, "Name"="nixnet_grpc_SystemOpenRequest", "Type Url"="nixnet_grpc.SystemOpenRequest", "Elements"=[{"Field Name"="session_name", "Embedded Message Name"="", "Protobuf Index"=1, "MessageElementType"=enum."StringValue", "Repeated"=FALSE, "Is in Oneof"=FALSE, "Oneof Container Name"=""}, {"Field Name"="initialization_behavior", "Embedded Message Name"="nidevice_grpc_SessionInitializationBehavior", "Protobuf Index"=2, "MessageElementType"=enum."EnumValue", "Repeated"=FALSE, "Is in Oneof"=FALSE, "Oneof Container Name"=""}], "Has Oneof"=FALSE}, {"Version"=2, "Name"="nixnet_grpc_SystemOpenResponse", "Type Url"="nixnet_grpc.SystemOpenResponse", "Elements"=[{"Field Name"="status", "Embedded Message Name"="", "Protobuf Index"=1, "MessageElementType"=enum."Int32Value", "Repeated"=FALSE, "Is in Oneof"=FALSE, "Oneof Container Name"=""}, {"Field Name"="system", "Embedded Message Name"="nidevice_grpc_Session", "Protobuf Index"=2, "MessageElementType"=enum."MessageValue", "Repeated"=FALSE, "Is in Oneof"=FALSE, "Oneof Container Name"=""}, {"Field Name"="new_session_initialized", "Embedded Message Name"="", "Protobuf Index"=3, "MessageElementType"=enum."BoolValue", "Repeated"=FALSE, "Is in Oneof"=FALSE, "Oneof Container Name"=""}], "Has Oneof"=FALSE}, {"Version"=2, "Name"="nixnet_grpc_WaitRequest", "Type Url"="nixnet_grpc.WaitRequest", "Elements"=[{"Field Name"="session", "Embedded Message Name"="nidevice_grpc_Session", "Protobuf Index"=1, "MessageElementType"=enum."MessageValue", "Repeated"=FALSE, "Is in Oneof"=FALSE, "Oneof Container Name"=""}, {"Field Name"="selected_index", "Embedded Message Name"="", "Protobuf Index"=-1, "MessageElementType"=enum."Int32Value", "Repeated"=FALSE, "Is in Oneof"=TRUE, "Oneof Container Name"="nixnet_grpc_WaitRequest_condition_enum"}, {"Field Name"="condition", "Embedded Message Name"="nixnet_grpc_WaitCondition", "Protobuf Index"=2, "MessageElementType"=enum."EnumValue", "Repeated"=FALSE, "Is in Oneof"=TRUE, "Oneof Container Name"="nixnet_grpc_WaitRequest_condition_enum"}, {"Field Name"="condition_raw", "Embedded Message Name"="", "Protobuf Index"=3, "MessageElementType"=enum."UInt32Value", "Repeated"=FALSE, "Is in Oneof"=TRUE, "Oneof Container Name"="nixnet_grpc_WaitRequest_condition_enum"}, {"Field Name"="param_in", "Embedded Message Name"="", "Protobuf Index"=4, "MessageElementType"=enum."UInt32Value", "Repeated"=FALSE, "Is in Oneof"=FALSE, "Oneof Container Name"=""}, {"Field Name"="timeout", "Embedded Message Name"="", "Protobuf Index"=5, "MessageElementType"=enum."DoubleValue", "Repeated"=FALSE, "Is in Oneof"=FALSE, "Oneof Container Name"=""}], "Has Oneof"=TRUE}, {"Version"=2, "Name"="nixnet_grpc_WaitResponse", "Type Url"="nixnet_grpc.WaitResponse", "Elements"=[{"Field Name"="status", "Embedded Message Name"="", "Protobuf Index"=1, "MessageElementType"=enum."Int32Value", "Repeated"=FALSE, "Is in Oneof"=FALSE, "Oneof Container Name"=""}, {"Field Name"="param_out", "Embedded Message Name"="", "Protobuf Index"=2, "MessageElementType"=enum."UInt32Value", "Repeated"=FALSE, "Is in Oneof"=FALSE, "Oneof Container Name"=""}], "Has Oneof"=FALSE}, {"Version"=2, "Name"="nixnet_grpc_WriteFrameRequest", "Type Url"="nixnet_grpc.WriteFrameRequest", "Elements"=[{"Field Name"="session", "Embedded Message Name"="nidevice_grpc_Session", "Protobuf Index"=1, "MessageElementType"=enum."MessageValue", "Repeated"=FALSE, "Is in Oneof"=FALSE, "Oneof Container Name"=""}, {"Field Name"="buffer", "Embedded Message Name"="nixnet_grpc_FrameBufferRequest", "Protobuf Index"=2, "MessageElementType"=enum."MessageValue", "Repeated"=TRUE, "Is in Oneof"=FALSE, "Oneof Container Name"=""}, {"Field Name"="selected_index", "Embedded Message Name"="", "Protobuf Index"=-1, "MessageElementType"=enum."Int32Value", "Repeated"=FALSE, "Is in Oneof"=TRUE, "Oneof Container Name"="nixnet_grpc_WriteFrameRequest_timeout_enum"}, {"Field Name"="timeout", "Embedded Message Name"="nixnet_grpc_TimeOut", "Protobuf Index"=3, "MessageElementType"=enum."EnumValue", "Repeated"=FALSE, "Is in Oneof"=TRUE, "Oneof Container Name"="nixnet_grpc_WriteFrameRequest_timeout_enum"}, {"Field Name"="timeout_raw", "Embedded Message Name"="", "Protobuf Index"=4, "MessageElementType"=enum."DoubleValue", "Repeated"=FALSE, "Is in Oneof"=TRUE, "Oneof Container Name"="nixnet_grpc_WriteFrameRequest_timeout_enum"}], "Has Oneof"=TRUE}, {"Version"=2, "Name"="nixnet_grpc_WriteFrameResponse", "Type Url"="nixnet_grpc.WriteFrameResponse", "Elements"=[{"Field Name"="status", "Embedded Message Name"="", "Protobuf Index"=1, "MessageElementType"=enum."Int32Value", "Repeated"=FALSE, "Is in Oneof"=FALSE, "Oneof Container Name"=""}], "Has Oneof"=FALSE}, {"Version"=2, "Name"="nixnet_grpc_WriteSignalSinglePointRequest", "Type Url"="nixnet_grpc.WriteSignalSinglePointRequest", "Elements"=[{"Field Name"="session", "Embedded Message Name"="nidevice_grpc_Session", "Protobuf Index"=1, "MessageElementType"=enum."MessageValue", "Repeated"=FALSE, "Is in Oneof"=FALSE, "Oneof Container Name"=""}, {"Field Name"="value_buffer", "Embedded Message Name"="", "Protobuf Index"=2, "MessageElementType"=enum."DoubleValue", "Repeated"=TRUE, "Is in Oneof"=FALSE, "Oneof Container Name"=""}], "Has Oneof"=FALSE}, {"Version"=2, "Name"="nixnet_grpc_WriteSignalSinglePointResponse", "Type Url"="nixnet_grpc.WriteSignalSinglePointResponse", "Elements"=[{"Field Name"="status", "Embedded Message Name"="", "Protobuf Index"=1, "MessageElementType"=enum."Int32Value", "Repeated"=FALSE, "Is in Oneof"=FALSE, "Oneof Container Name"=""}], "Has Oneof"=FALSE}, {"Version"=2, "Name"="nixnet_grpc_WriteSignalWaveformRequest", "Type Url"="nixnet_grpc.WriteSignalWaveformRequest", "Elements"=[{"Field Name"="session", "Embedded Message Name"="nidevice_grpc_Session", "Protobuf Index"=1, "MessageElementType"=enum."MessageValue", "Repeated"=FALSE, "Is in Oneof"=FALSE, "Oneof Container Name"=""}, {"Field Name"="selected_index", "Embedded Message Name"="", "Protobuf Index"=-1, "MessageElementType"=enum."Int32Value", "Repeated"=FALSE, "Is in Oneof"=TRUE, "Oneof Container Name"="nixnet_grpc_WriteSignalWaveformRequest_timeout_enum"}, {"Field Name"="timeout", "Embedded Message Name"="nixnet_grpc_TimeOut", "Protobuf Index"=2, "MessageElementType"=enum."EnumValue", "Repeated"=FALSE, "Is in Oneof"=TRUE, "Oneof Container Name"="nixnet_grpc_WriteSignalWaveformRequest_timeout_enum"}, {"Field Name"="timeout_raw", "Embedded Message Name"="", "Protobuf Index"=3, "MessageElementType"=enum."DoubleValue", "Repeated"=FALSE, "Is in Oneof"=TRUE, "Oneof Container Name"="nixnet_grpc_WriteSignalWaveformRequest_timeout_enum"}, {"Field Name"="value_buffer", "Embedded Message Name"="", "Protobuf Index"=4, "MessageElementType"=enum."DoubleValue", "Repeated"=TRUE, "Is in Oneof"=FALSE, "Oneof Container Name"=""}], "Has Oneof"=TRUE}, {"Version"=2, "Name"="nixnet_grpc_WriteSignalWaveformResponse", "Type Url"="nixnet_grpc.WriteSignalWaveformResponse", "Elements"=[{"Field Name"="status", "Embedded Message Name"="", "Protobuf Index"=1, "MessageElementType"=enum."Int32Value", "Repeated"=FALSE, "Is in Oneof"=FALSE, "Oneof Container Name"=""}], "Has Oneof"=FALSE}, {"Version"=2, "Name"="nixnet_grpc_WriteSignalXYRequest", "Type Url"="nixnet_grpc.WriteSignalXYRequest", "Elements"=[{"Field Name"="session", "Embedded Message Name"="nidevice_grpc_Session", "Protobuf Index"=1, "MessageElementType"=enum."MessageValue", "Repeated"=FALSE, "Is in Oneof"=FALSE, "Oneof Container Name"=""}, {"Field Name"="selected_index", "Embedded Message Name"="", "Protobuf Index"=-1, "MessageElementType"=enum."Int32Value", "Repeated"=FALSE, "Is in Oneof"=TRUE, "Oneof Container Name"="nixnet_grpc_WriteSignalXYRequest_timeout_enum"}, {"Field Name"="timeout", "Embedded Message Name"="nixnet_grpc_TimeOut", "Protobuf Index"=2, "MessageElementType"=enum."EnumValue", "Repeated"=FALSE, "Is in Oneof"=TRUE, "Oneof Container Name"="nixnet_grpc_WriteSignalXYRequest_timeout_enum"}, {"Field Name"="timeout_raw", "Embedded Message Name"="", "Protobuf Index"=3, "MessageElementType"=enum."DoubleValue", "Repeated"=FALSE, "Is in Oneof"=TRUE, "Oneof Container Name"="nixnet_grpc_WriteSignalXYRequest_timeout_enum"}, {"Field Name"="value_buffer", "Embedded Message Name"="", "Protobuf Index"=4, "MessageElementType"=enum."DoubleValue", "Repeated"=TRUE, "Is in Oneof"=FALSE, "Oneof Container Name"=""}, {"Field Name"="timestamp_buffer", "Embedded Message Name"="", "Protobuf Index"=5, "MessageElementType"=enum."UInt64Value", "Repeated"=TRUE, "Is in Oneof"=FALSE, "Oneof Container Name"=""}, {"Field Name"="num_pairs_buffer", "Embedded Message Name"="", "Protobuf Index"=6, "MessageElementType"=enum."UInt32Value", "Repeated"=TRUE, "Is in Oneof"=FALSE, "Oneof Container Name"=""}], "Has Oneof"=TRUE}, {"Version"=2, "Name"="nixnet_grpc_WriteSignalXYResponse", "Type Url"="nixnet_grpc.WriteSignalXYResponse", "Elements"=[{"Field Name"="status", "Embedded Message Name"="", "Protobuf Index"=1, "MessageElementType"=enum."Int32Value", "Repeated"=FALSE, "Is in Oneof"=FALSE, "Oneof Container Name"=""}], "Has Oneof"=FALSE}, {"Version"=2, "Name"="nixnet_grpc_WriteStateRequest", "Type Url"="nixnet_grpc.WriteStateRequest", "Elements"=[{"Field Name"="session", "Embedded Message Name"="nidevice_grpc_Session", "Protobuf Index"=1, "MessageElementType"=enum."MessageValue", "Repeated"=FALSE, "Is in Oneof"=FALSE, "Oneof Container Name"=""}, {"Field Name"="selected_index", "Embedded Message Name"="", "Protobuf Index"=-1, "MessageElementType"=enum."Int32Value", "Repeated"=FALSE, "Is in Oneof"=TRUE, "Oneof Container Name"="nixnet_grpc_WriteStateRequest_state_id_enum"}, {"Field Name"="state_id", "Embedded Message Name"="nixnet_grpc_WriteState", "Protobuf Index"=2, "MessageElementType"=enum."EnumValue", "Repeated"=FALSE, "Is in Oneof"=TRUE, "Oneof Container Name"="nixnet_grpc_WriteStateRequest_state_id_enum"}, {"Field Name"="state_id_raw", "Embedded Message Name"="", "Protobuf Index"=3, "MessageElementType"=enum."UInt32Value", "Repeated"=FALSE, "Is in Oneof"=TRUE, "Oneof Container Name"="nixnet_grpc_WriteStateRequest_state_id_enum"}, {"Field Name"="state_value", "Embedded Message Name"="nixnet_grpc_WriteStateValue", "Protobuf Index"=4, "MessageElementType"=enum."MessageValue", "Repeated"=FALSE, "Is in Oneof"=FALSE, "Oneof Container Name"=""}], "Has Oneof"=TRUE}, {"Version"=2, "Name"="nixnet_grpc_WriteStateResponse", "Type Url"="nixnet_grpc.WriteStateResponse", "Elements"=[{"Field Name"="status", "Embedded Message Name"="", "Protobuf Index"=1, "MessageElementType"=enum."Int32Value", "Repeated"=FALSE, "Is in Oneof"=FALSE, "Oneof Container Name"=""}], "Has Oneof"=FALSE}, {"Version"=2, "Name"="nidevice_grpc_Session", "Type Url"="nidevice_grpc.Session", "Elements"=[{"Field Name"="name", "Embedded Message Name"="", "Protobuf Index"=1, "MessageElementType"=enum."StringValue", "Repeated"=FALSE, "Is in Oneof"=FALSE, "Oneof Container Name"=""}], "Has Oneof"=FALSE}]  # Messages MetaData
      n2 = call <vilib>:"Register Message Metadata.vi"("error in"=w10, "Messages"=w11, "gRPCid in"=w9) -> ("error out"=w7:errorcluster, "gRPCid out"=w8:T1)  [unwired: 7 in]
      n3 = call <vilib>:"Register Enum Metadata.vi"("error in"=w7, "Enum Metadata"=w5, "gRPCid in"=w8) -> ("error out"=w6:errorcluster)  [unwired: 7 in, 1 out]
    }
    frame Error {
    }
  }
  "error out" <- w4
  "gRPC ID Out" <- w1
